vi "Main.vi"() -> ()   [LabVIEW 2011]
uses:
  GUI/Graph/Plot selector.ctl
  Application Structure/User Control/User Indikator.ctl
  Application Structure/User Control/Super User bool indikator.ctl
  GUI/Shart Time Selector.ctl
  GUI/Analog Var Disp 0 sif.ctl
  GUI/Status indicator Black Small.ctl
  GUI/Controls/Graphical rep/Tool Angle.ctl
  Measurments Handling/Cat Alm temp.ctl
  GUI/Status indicator white.ctl
  Measurments Handling/Cat Alm Press.ctl
  Measurments Handling/Cat Alm Gen.ctl
  Measurments Handling/Cat Alm Pow.ctl
  Measurments Handling/Digital GUI/Digital Display cluster.ctl
  Measurments Handling/Digital GUI/Digital Disp small indicator.ctl
  Measurments Handling/Digital GUI/Digital Tricolour Display cluster.ctl
  Measurments Handling/Digital GUI/Digital Tricolour Disp small indicator.ctl
  GUI/Controls/Tristate/Tristate left.ctl
  GUI/Controls/Tristate/Tristate right.ctl
  GUI/Controls/Slips boolean.ctl
  GUI/Controls/Pressure failing boolean long.ctl
  Tool/Tab with tool type tabs.ctl
  GUI/Analog Var Disp Large.ctl
  GUI/Controls/Signal Bar Graph.ctl
  Application Structure/Loop ID.ctl
  emi Lib/System 01/1 - GUI/Background/emi_System Colors.ctl
  emi Lib/System 01/1 - GUI/Background/Private/_emi_ Color defenition.ctl
  emi Lib/Basic/0 - General/Graphix/Private/emi_List Of Graphix.ctl
  Application Structure/System ID.ctl
  emi Lib/System 01/0 - General/S&E reporting/Private/_emi_ S&E Message type.ctl
  emi cndiates/E&S/Monitor/Actino S&E monitor.ctl
  Application Structure/QSM State List.ctl
  Sequence automation/Sequence steps config..ctl
  Sequence automation/Single criteria cluster.ctl
  Sequence automation/Criteria types.ctl
  Sequence automation/Boolean operation.ctl
  Application Structure/Options/Action GFV Settings.ctl
  <vilib>/Platform/TimedLoop/XDataNode/timing_clust.ctl
  <vilib>/Platform/TimedLoop/XDataNode/nitl_modes.ctl
  <vilib>/Platform/TimedLoop/XDataNode/wakeup.ctl
  PCP interface/High Level/PCP High Level Commands.ctl
  PCP interface/PSU Type.ctl
  GUI/Controll refrence groups.ctl
  GUI/Graph/Annotations Tip Strip FGV_cluster.ctl
  Application Structure/Dialog Loop/Dialog selection cluster.ctl
  Application Structure/Dialog box ID.ctl
  Application Structure/Mem Ctls/Mem Ctl Custer.ctl
  Application Structure/Mem Ctls/Mem Graph Ctl Custer.ctl
  GUI/Graph/Y scale cluster.ctl
  GUI/Graph vindu/Settigner fra Main.ctl
  Annotation/Annotation Message.ctl
  Annotation/Actin Annotatino Holder.ctl
  PCP interface/High Level/PCP High Level Telegram.ctl
  Tool/Stroker/def/Tool specific commands.ctl
  Tool/List of tools.ctl
  Events/User Event List.ctl
  emi cndiates/E&S/reate/S&E Event source.ctl
  Tool/Variable List Tool Analog.ctl
  Measurments Handling/Common/Variable List Common Digital.ctl
  Tool/Variable List Tool Digital.ctl
  Measurments Handling/Status Digitalish.ctl
  GUI/Graph/Annotations Tip Strip FGV_data cluster.ctl
  <vilib>/Utility/miscctls.llb/LVPoint32TypeDef.ctl
  <vilib>/event_ctls.llb/eventvkey.ctl
  Sequence automation/Complete sequence cluster holder.ctl
  Sequence automation/User input.ctl
  Measurments Handling/Common/Variable List Common Analog.ctl
  emi Lib/System 01/0 - General/App/Loop control 2/Private/_emi_SMLoop Control Single.vi
  emi Lib/System 01/0 - General/App/Loop control 2/Private/_emi_SMLoop Get State Single.vi
  emi Lib/System 01/0 - General/emi_Set System ID.vi
  emi Lib/System 01/0 - General/App/Loop control 2/Private/_emi_ SMLoop start condition.vi
  emi Lib/System 01/0 - General/App/Loop control 2/Private/_emi_ SMLoop Error Check.vi
  emi Lib/Basic/0 - General/Error/emi_Is Error.vi
  emi Lib/System 01/0 - General/App/Loop control 2/Private/_emi_SMLoop Register new.vi
  emi Lib/System 01/0 - General/emi_Read System ID.vi
  emi Lib/Basic/0 - General/App/emi_Is Dev enviroment.vi
  emi Lib/System 01/0 - General/S&E reporting/emi_Send S&E Error message.vi
  emi Lib/Basic/0 - General/Error/emi_ Is Error state.vi
  emi Lib/System 01/0 - General/Private/_emi_GFV System ID.vi
  emi Lib/System 01/0 - General/S&E reporting/Private/_emi_S&E Q Generator.vi
  Application Structure/QSM/QSM Q holder.vi
  emi Lib/System 01/1 - GUI/Profiling Mar-In/Splash & About/Private/emi_Splash&About Screen.vi
  <vilib>/Utility/VariantDataType/GetNumericInfo.vi
  emi Lib/System 01/0 - General/App/Loop control/Private/_emi_GFV Loop Enable.vi
  emi Lib/System 01/0 - General/App/Loop control/Private/_emi_GFV Loop Linking.vi
  GUI/GFV GUI PCP shown connected.vi
  emi Lib/Basic/1 - GUI/Control tools/emi_Control Enable & Visibility.vi
  emi Lib/Basic/1 - GUI/Control tools/Private/emi_Control enable and visibility array.vi
  emi Lib/System 01/0 - General/Debug/Private/_emi_GFV Debug Disp.vi
  emi Lib/System 01/0 - General/App/Private/_emi_GFV App Close.vi
  emi Lib/System 01/0 - General/App/Loop control/Private/_emi_GFV Loop Running.vi
  emi Lib/Basic/0 - General/App/emi_Application Folder.vi
  emi Lib/System 01/0 - General/App/Loop control 2/Private/_emi_ SMLoop Restart.vi
  emi Lib/System 01/0 - General/App/Loop control 2/Private/_emi_ SMLoop Restart Counter.vi
  emi Lib/System 01/0 - General/App/Loop control/Private/_emi_GFV stop a loop so it can reset.vi
  emi Lib/Basic/0 - General/Time/Private/emi_Time offset holder.vi
  Measurments Handling/Get Modem Status Digital Vars.vi
  <vilib>/Platform/TimedLoop/XDataNode/XDataNode.xnode
  <vilib>/Platform/TimedLoop/XDataNode/XDNodeRunTimeDep.lvlib
  Measurments Handling/Action Analog Handler.ctl
panel:
  out "Subsea Bar Graph":T1 {"Gain" format="%#.0f"; "Signal Quality" format="%#.0f"}
  out "Topside Bar Graph":T1 {"Gain" format="%#.0f"; "Signal Quality" format="%#.0f"}
  in  "Annotation Tip Strip":string
  out "Chart 1":dbl[][](graph)
  in  "Start Run":bool
  in  "String Check Rec":bool
  out "Recording":bool
  in  "Inspect Upper Chart":bool caption="Inspect Chart"
  out "Beagle Panel":T2 caption="Depth"
  out "Annotation Chart":dbl(graph)
  in  "Calculate resistance":bool caption="Upd"
  in  "Start Motor":bool
  in  "Start Telemetry":bool
  out "Tool":T2 caption="Depth"
  out "PCP Control":T5 caption="Depth"
  out "Type tab 2":T7
  out "Str Error Tens1":u16(ring) caption="Error Strk P2"
  out "Strok Tension Sub 1":T2 caption="Upper Tension Sub"
  out "Stroker  2":dbl(slide) caption="Stroker position" scale=0.0..500.0
  out "Strok Pressure 1":T2 caption="Pressure1"
  out "Strok Pressure 2":T2 caption="Pressure2"
  out "Strok Solenoid":T2 caption="Solenoid"
  out "Str Error P1":u16(ring) caption="Error Strk P1"
  out "Str Error P2":u16(ring) caption="Error Strk P2"
  out "Str Error Sol":u16(ring) caption="Error Strk olenoid"
  out "Error Dr Sol":u16(ring)
  out "Error Dr P2":u16(ring)
  out "Error Dr P1":u16(ring)
  out "Dr Solenoid":T2 caption="Solenoid"
  out "Dr Pressure 2":T2 caption="Pressure2"
  out "Dr Pressure 1":T2 caption="Pressure1"
  out "Error Tr Tension Sub 1":u16(ring) caption="Error Dr Sol"
  out "Trac Tension Sub 1":T2 caption="Upper Tension Sub"
  out "Trac Tension Sub 2":T2 caption="Lower Tension Sub"
  out "Error Tr Tension Sub 2":u16(ring) caption="Error Dr Sol"
  out "Type tab 3":T7
  in  "Stroker Tension Sub Zero":bool caption="Solonoid 1 On"
  out "Upper Tension Sub":T8={"Value"=nan, "Unit"="", "Status"=0}
  out "Trac - Lower Tension Sub":T8={"Value"=nan, "Unit"="", "Status"=0} caption="Lower Tension Sub"
  out "Trac - Upper Tension Sub":T8={"Value"=nan, "Unit"="", "Status"=0} caption="Upper Tension Sub"
  in  "Tractor Tension Sub Zero":bool caption="Solonoid 1 On"
  out "Type tab 1":T7
  in  "Force Zero":bool caption="Solonoid 1 On"
  in  "Stroker force limit":dbl=0.5 caption="tonne" min=0.5 step=0.1
  out "Slips total":bool
  out "Stroker":dbl(slide) caption="Stroker position" scale=0.0..500.0
  in  "Stroker Anchor out":bool caption="Solonoid 1 On"
  in  "Stroker Anchor in":bool caption="Solonoid 1 On"
  out "Stroke extenstion":T10={"Value"=nan, "Unit"="", "Status"=0} caption="Resistance" {"Value" format="%#.0f"}
  out "Moving left":T11
  out "Moving right":T12
  out "Stroke force":T10={"Value"=nan, "Unit"="", "Status"=0} caption="Resistance" {"Value" format="%.1f"}
  out "\"Stroke in\" Pressure":T10={"Value"=nan, "Unit"="", "Status"=0} caption="Resistance"
  out "\"Stroke out\" Pressure":T10={"Value"=nan, "Unit"="", "Status"=0} caption="Resistance"
  out "Slips Venstre":T13
  out "Slips Høyre":T13
  out "pressure falling":T14
  in  "Stroker Stroke Stop":bool caption="Solonoid 1 On"
  in  "Stroke setpoint":dbl(slide) caption="mm" min=0.0 step=1.0 scale=0.0..500.0 scale format="%.0g"
  in  "Stroker Stroke Go To":bool caption="Solonoid 1 On"
  in  "Stroker Stroke In":bool caption="Solonoid 1 On"
  in  "Stroker Stroke Out":bool caption="Solonoid 1 On"
  out "Distance from target:":dbl caption="Target seeking" format="%.1f"
  in  "Driller Anchor in":bool caption="Solonoid 1 On"
  in  "Driller Anchor out":bool caption="Solonoid 1 On"
  out "Dr Oil filling mode":T2 caption="Oil filling mode"
  out "Drill bit direaction":T2 caption="Mill Bit direction"
  in  "Driller Stroke out":bool caption="Solonoid 1 On"
  in  "Driller Stroke in":bool caption="Solonoid 1 On"
  in  "Driller Oil filling mode":bool caption="Solonoid 1 On"
  out "Weight on bit":T10={"Value"=nan, "Unit"="", "Status"=0} caption="Resistance" {"Value" format="%#.1f"}
  out "Driller RPM":T10={"Value"=nan, "Unit"="", "Status"=0} caption="RPM" {"Value" format="%#.1f"}
  out "Torque":T10={"Value"=nan, "Unit"="", "Status"=0} caption="Resistance" {"Value" format="%#.1f"}
  in  "Driller RPM":dbl(slide) caption="RPM" min=0.0 max=600.0 scale=0.0..600.0
  in  "Driller Stop":bool
  in  "Driller A Dir":bool
  in  "Driller Dir B":bool
  out "Slips":T13
  out "Sequence user input name":string
  in  "Sequence user input":dbl min=25.0 max=500.0
  out "Next step":string
  out "Current step":string
  out "Time spent on sequence step":string
  out "Sequence progress":string
  in  "Approve step":bool
  in  "Stopp sequence":bool
  in  "Start sequence":bool
  in  "Sequence to run":u16(ring) items=["Default", "demo", "tyts"]
  in  "Relays off":bool caption="Solenoid 1 Off"
  in  "Relays on":bool caption="All Relays"
  out "Tool Rotation":T15 scale=0.0..360.0 scale format="%#.0f"
  out "Relay Status":T5 caption="Depth"
  in  "Upd Default resistance":bool caption="Upd"
  in  "Force Default resistance":bool caption="Force"
  in  "Resistance(Ohm)":dbl=40.0 min=0.0 max=1200.0 format="%#.0f"
  out "HV out":T5 caption="Depth"
  out "PSU":T2 caption="Depth"
  out "PCP":T2 caption="Depth"
  out "Alarms":string[][](table)
  out "Power Level":T16
  out "General level":T17
  out "Press level":T18
  out "Temp level":T19
  out "Tool Angle":T15 caption="Tool Inclination" scale=0.0..180.0
  in  "Create Anotation":bool
  in  "Inspect Lower Chart":bool caption="Inspect Chart"
  out "Controller Temp.":T10={"Value"=nan, "Unit"="", "Status"=0} caption="Tool Temperature"
  in  "Plot G2 R2":T20 {"Line Width" items=["0", "1", "2", "3", "4", "5"]; "Var Tag" items=[""=0, "HVPSU Head Voltage(V)"=1, "HVPSU Current(A)"=3, "Winch Depth(m)"=5, "Winch Line Speed(m/min)"=6, "Winch Wire Tension(kg)"=7, "Tool Max Temperature(degC)"=8, "Tool Acceleration Sum(g)"=15, "Tool Inclination(deg)"=16, "Tool Rotation(deg)"=17, "Head Voltage(V)"=27, "Stroke Extension(mm)"=38, "Stroke Force(tonne)"=41, "Stroker Upper Tension Sub(kg)"=44, "Tractor Upper Tension Sub(kg)"=48, "Tractor Lower Tension Sub(kg)"=49, "-"=100, "HVPSU TS Voltage(V)"=2, "Tool (Controller) Temperature(degC)"=9, "Tool Acceleration X(g)"=12, "Tool Acceleration Y(g)"=13, "Tool Acceleration Z(g)"=14, "PSU Temp(degC)"=26, "Upper Tension Sub Temp(degC)"=30, "Tool Upper Tension Sub Raw(kg)"=31, "Lower Tension Sub Temp(degC)"=32, "Tool Lower Tension Sub Raw(kg)"=33, "Stroke In Force(tonne)"=39, "Stroke Out Force(tonne)"=40, "Stroker Pressure 1(bar)"=42, "Stroker Pressure 2(bar)"=43, "Tool Temperature sensor(degC)"=52, "Tool Motor Current(A)"=54, "TS_Signal_Quality(NA)"=58, "TS_Gain(NA)"=60, "DH_Signal_Quality(NA)"=61, "DH_Gain(NA)"=63, "Link_Status(NA)"=64, "-"=101, "PCP Cable Resistance(Ohm)"=4, "Tool Supply Voltage(V)"=10, "Tool (Controller) Current(A)"=11, "Tool GP Sensor 1(V)"=18, "Tool GP Sensor 2(V)"=19, "Tool (Pressure 1) Temperature(degC)"=20, "Tool Pressure 1 RAW(bar)"=21, "Tool (Pressure 2) Temperature(degC)"=22, "Tool Pressure 2 RAW(bar)"=23, "Tool (Solenoid) Temperature(degC)"=24, "Tool Solenoid Position(m)"=25, "PSU Main Voltage out(V)"=28, "PSU Main Current out(A)"=29, "Tool Motor Voltage(V)"=53, "Tool Motor Torque(tonne)"=55, "Tool weight on bit(tonne)"=56, "Tool Motor RPM(RPM)"=57, "TS_PCB_Temp(degC)"=59, "DH_PCB_Temp(degC)"=62]}
  in  "Plot G2 R1":T20 {"Line Width" items=["0", "1", "2", "3", "4", "5"]; "Var Tag" items=[""=0, "HVPSU Head Voltage(V)"=1, "HVPSU Current(A)"=3, "Winch Depth(m)"=5, "Winch Line Speed(m/min)"=6, "Winch Wire Tension(kg)"=7, "Tool Max Temperature(degC)"=8, "Tool Acceleration Sum(g)"=15, "Tool Inclination(deg)"=16, "Tool Rotation(deg)"=17, "Head Voltage(V)"=27, "Stroke Extension(mm)"=38, "Stroke Force(tonne)"=41, "Stroker Upper Tension Sub(kg)"=44, "Tractor Upper Tension Sub(kg)"=48, "Tractor Lower Tension Sub(kg)"=49, "-"=100, "HVPSU TS Voltage(V)"=2, "Tool (Controller) Temperature(degC)"=9, "Tool Acceleration X(g)"=12, "Tool Acceleration Y(g)"=13, "Tool Acceleration Z(g)"=14, "PSU Temp(degC)"=26, "Upper Tension Sub Temp(degC)"=30, "Tool Upper Tension Sub Raw(kg)"=31, "Lower Tension Sub Temp(degC)"=32, "Tool Lower Tension Sub Raw(kg)"=33, "Stroke In Force(tonne)"=39, "Stroke Out Force(tonne)"=40, "Stroker Pressure 1(bar)"=42, "Stroker Pressure 2(bar)"=43, "Tool Temperature sensor(degC)"=52, "Tool Motor Current(A)"=54, "TS_Signal_Quality(NA)"=58, "TS_Gain(NA)"=60, "DH_Signal_Quality(NA)"=61, "DH_Gain(NA)"=63, "Link_Status(NA)"=64, "-"=101, "PCP Cable Resistance(Ohm)"=4, "Tool Supply Voltage(V)"=10, "Tool (Controller) Current(A)"=11, "Tool GP Sensor 1(V)"=18, "Tool GP Sensor 2(V)"=19, "Tool (Pressure 1) Temperature(degC)"=20, "Tool Pressure 1 RAW(bar)"=21, "Tool (Pressure 2) Temperature(degC)"=22, "Tool Pressure 2 RAW(bar)"=23, "Tool (Solenoid) Temperature(degC)"=24, "Tool Solenoid Position(m)"=25, "PSU Main Voltage out(V)"=28, "PSU Main Current out(A)"=29, "Tool Motor Voltage(V)"=53, "Tool Motor Torque(tonne)"=55, "Tool weight on bit(tonne)"=56, "Tool Motor RPM(RPM)"=57, "TS_PCB_Temp(degC)"=59, "DH_PCB_Temp(degC)"=62]}
  out "Chart 2":dbl[][](graph)
  in  "Plot G2 L2":T20 {"Line Width" items=["0", "1", "2", "3", "4", "5"]; "Var Tag" items=[""=0, "HVPSU Head Voltage(V)"=1, "HVPSU Current(A)"=3, "Winch Depth(m)"=5, "Winch Line Speed(m/min)"=6, "Winch Wire Tension(kg)"=7, "Tool Max Temperature(degC)"=8, "Tool Acceleration Sum(g)"=15, "Tool Inclination(deg)"=16, "Tool Rotation(deg)"=17, "Head Voltage(V)"=27, "Stroke Extension(mm)"=38, "Stroke Force(tonne)"=41, "Stroker Upper Tension Sub(kg)"=44, "Tractor Upper Tension Sub(kg)"=48, "Tractor Lower Tension Sub(kg)"=49, "-"=100, "HVPSU TS Voltage(V)"=2, "Tool (Controller) Temperature(degC)"=9, "Tool Acceleration X(g)"=12, "Tool Acceleration Y(g)"=13, "Tool Acceleration Z(g)"=14, "PSU Temp(degC)"=26, "Upper Tension Sub Temp(degC)"=30, "Tool Upper Tension Sub Raw(kg)"=31, "Lower Tension Sub Temp(degC)"=32, "Tool Lower Tension Sub Raw(kg)"=33, "Stroke In Force(tonne)"=39, "Stroke Out Force(tonne)"=40, "Stroker Pressure 1(bar)"=42, "Stroker Pressure 2(bar)"=43, "Tool Temperature sensor(degC)"=52, "Tool Motor Current(A)"=54, "TS_Signal_Quality(NA)"=58, "TS_Gain(NA)"=60, "DH_Signal_Quality(NA)"=61, "DH_Gain(NA)"=63, "Link_Status(NA)"=64, "-"=101, "PCP Cable Resistance(Ohm)"=4, "Tool Supply Voltage(V)"=10, "Tool (Controller) Current(A)"=11, "Tool GP Sensor 1(V)"=18, "Tool GP Sensor 2(V)"=19, "Tool (Pressure 1) Temperature(degC)"=20, "Tool Pressure 1 RAW(bar)"=21, "Tool (Pressure 2) Temperature(degC)"=22, "Tool Pressure 2 RAW(bar)"=23, "Tool (Solenoid) Temperature(degC)"=24, "Tool Solenoid Position(m)"=25, "PSU Main Voltage out(V)"=28, "PSU Main Current out(A)"=29, "Tool Motor Voltage(V)"=53, "Tool Motor Torque(tonne)"=55, "Tool weight on bit(tonne)"=56, "Tool Motor RPM(RPM)"=57, "TS_PCB_Temp(degC)"=59, "DH_PCB_Temp(degC)"=62]}
  in  "Plot G2 L1":T20 {"Line Width" items=["0", "1", "2", "3", "4", "5"]; "Var Tag" items=[""=0, "HVPSU Head Voltage(V)"=1, "HVPSU Current(A)"=3, "Winch Depth(m)"=5, "Winch Line Speed(m/min)"=6, "Winch Wire Tension(kg)"=7, "Tool Max Temperature(degC)"=8, "Tool Acceleration Sum(g)"=15, "Tool Inclination(deg)"=16, "Tool Rotation(deg)"=17, "Head Voltage(V)"=27, "Stroke Extension(mm)"=38, "Stroke Force(tonne)"=41, "Stroker Upper Tension Sub(kg)"=44, "Tractor Upper Tension Sub(kg)"=48, "Tractor Lower Tension Sub(kg)"=49, "-"=100, "HVPSU TS Voltage(V)"=2, "Tool (Controller) Temperature(degC)"=9, "Tool Acceleration X(g)"=12, "Tool Acceleration Y(g)"=13, "Tool Acceleration Z(g)"=14, "PSU Temp(degC)"=26, "Upper Tension Sub Temp(degC)"=30, "Tool Upper Tension Sub Raw(kg)"=31, "Lower Tension Sub Temp(degC)"=32, "Tool Lower Tension Sub Raw(kg)"=33, "Stroke In Force(tonne)"=39, "Stroke Out Force(tonne)"=40, "Stroker Pressure 1(bar)"=42, "Stroker Pressure 2(bar)"=43, "Tool Temperature sensor(degC)"=52, "Tool Motor Current(A)"=54, "TS_Signal_Quality(NA)"=58, "TS_Gain(NA)"=60, "DH_Signal_Quality(NA)"=61, "DH_Gain(NA)"=63, "Link_Status(NA)"=64, "-"=101, "PCP Cable Resistance(Ohm)"=4, "Tool Supply Voltage(V)"=10, "Tool (Controller) Current(A)"=11, "Tool GP Sensor 1(V)"=18, "Tool GP Sensor 2(V)"=19, "Tool (Pressure 1) Temperature(degC)"=20, "Tool Pressure 1 RAW(bar)"=21, "Tool (Pressure 2) Temperature(degC)"=22, "Tool Pressure 2 RAW(bar)"=23, "Tool (Solenoid) Temperature(degC)"=24, "Tool Solenoid Position(m)"=25, "PSU Main Voltage out(V)"=28, "PSU Main Current out(A)"=29, "Tool Motor Voltage(V)"=53, "Tool Motor Torque(tonne)"=55, "Tool weight on bit(tonne)"=56, "Tool Motor RPM(RPM)"=57, "TS_PCB_Temp(degC)"=59, "DH_PCB_Temp(degC)"=62]}
  in  "HV AV":bool
  in  "HV ON":bool caption="HV PÅ"
  out "Tension":T10={"Value"=nan, "Unit"="", "Status"=0}
  out "Speed":T10={"Value"=nan, "Unit"="", "Status"=0} {"Value" format="%.1f"}
  out "Depth":T10={"Value"=nan, "Unit"="", "Status"=0} {"Value" format="%.1f"}
  out "Resistance":T10={"Value"=nan, "Unit"="", "Status"=0}
  out "Current":T10={"Value"=nan, "Unit"="", "Status"=0} {"Value" format="%.1f"}
  out "Alarm":bool
  out "Voltage Topside":T10={"Value"=nan, "Unit"="", "Status"=0}
  in  "Chart Visible Time selector":T21=enum."1 minute" caption="Time"
  in  "Plot G1 R2":T20 {"Line Width" items=["0", "1", "2", "3", "4", "5"]; "Var Tag" items=[""=0, "HVPSU Head Voltage(V)"=1, "HVPSU Current(A)"=3, "Winch Depth(m)"=5, "Winch Line Speed(m/min)"=6, "Winch Wire Tension(kg)"=7, "Tool Max Temperature(degC)"=8, "Tool Acceleration Sum(g)"=15, "Tool Inclination(deg)"=16, "Tool Rotation(deg)"=17, "Head Voltage(V)"=27, "Stroke Extension(mm)"=38, "Stroke Force(tonne)"=41, "Stroker Upper Tension Sub(kg)"=44, "Tractor Upper Tension Sub(kg)"=48, "Tractor Lower Tension Sub(kg)"=49, "-"=100, "HVPSU TS Voltage(V)"=2, "Tool (Controller) Temperature(degC)"=9, "Tool Acceleration X(g)"=12, "Tool Acceleration Y(g)"=13, "Tool Acceleration Z(g)"=14, "PSU Temp(degC)"=26, "Upper Tension Sub Temp(degC)"=30, "Tool Upper Tension Sub Raw(kg)"=31, "Lower Tension Sub Temp(degC)"=32, "Tool Lower Tension Sub Raw(kg)"=33, "Stroke In Force(tonne)"=39, "Stroke Out Force(tonne)"=40, "Stroker Pressure 1(bar)"=42, "Stroker Pressure 2(bar)"=43, "Tool Temperature sensor(degC)"=52, "Tool Motor Current(A)"=54, "TS_Signal_Quality(NA)"=58, "TS_Gain(NA)"=60, "DH_Signal_Quality(NA)"=61, "DH_Gain(NA)"=63, "Link_Status(NA)"=64, "-"=101, "PCP Cable Resistance(Ohm)"=4, "Tool Supply Voltage(V)"=10, "Tool (Controller) Current(A)"=11, "Tool GP Sensor 1(V)"=18, "Tool GP Sensor 2(V)"=19, "Tool (Pressure 1) Temperature(degC)"=20, "Tool Pressure 1 RAW(bar)"=21, "Tool (Pressure 2) Temperature(degC)"=22, "Tool Pressure 2 RAW(bar)"=23, "Tool (Solenoid) Temperature(degC)"=24, "Tool Solenoid Position(m)"=25, "PSU Main Voltage out(V)"=28, "PSU Main Current out(A)"=29, "Tool Motor Voltage(V)"=53, "Tool Motor Torque(tonne)"=55, "Tool weight on bit(tonne)"=56, "Tool Motor RPM(RPM)"=57, "TS_PCB_Temp(degC)"=59, "DH_PCB_Temp(degC)"=62]}
  in  "Plot G1 R1":T20={"Var Tag"=0, "Color"=16776704, "Line Width"=0} {"Line Width" items=["0", "1", "2", "3", "4", "5"]; "Var Tag" items=[""=0, "HVPSU Head Voltage(V)"=1, "HVPSU Current(A)"=3, "Winch Depth(m)"=5, "Winch Line Speed(m/min)"=6, "Winch Wire Tension(kg)"=7, "Tool Max Temperature(degC)"=8, "Tool Acceleration Sum(g)"=15, "Tool Inclination(deg)"=16, "Tool Rotation(deg)"=17, "Head Voltage(V)"=27, "Stroke Extension(mm)"=38, "Stroke Force(tonne)"=41, "Stroker Upper Tension Sub(kg)"=44, "Tractor Upper Tension Sub(kg)"=48, "Tractor Lower Tension Sub(kg)"=49, "-"=100, "HVPSU TS Voltage(V)"=2, "Tool (Controller) Temperature(degC)"=9, "Tool Acceleration X(g)"=12, "Tool Acceleration Y(g)"=13, "Tool Acceleration Z(g)"=14, "PSU Temp(degC)"=26, "Upper Tension Sub Temp(degC)"=30, "Tool Upper Tension Sub Raw(kg)"=31, "Lower Tension Sub Temp(degC)"=32, "Tool Lower Tension Sub Raw(kg)"=33, "Stroke In Force(tonne)"=39, "Stroke Out Force(tonne)"=40, "Stroker Pressure 1(bar)"=42, "Stroker Pressure 2(bar)"=43, "Tool Temperature sensor(degC)"=52, "Tool Motor Current(A)"=54, "TS_Signal_Quality(NA)"=58, "TS_Gain(NA)"=60, "DH_Signal_Quality(NA)"=61, "DH_Gain(NA)"=63, "Link_Status(NA)"=64, "-"=101, "PCP Cable Resistance(Ohm)"=4, "Tool Supply Voltage(V)"=10, "Tool (Controller) Current(A)"=11, "Tool GP Sensor 1(V)"=18, "Tool GP Sensor 2(V)"=19, "Tool (Pressure 1) Temperature(degC)"=20, "Tool Pressure 1 RAW(bar)"=21, "Tool (Pressure 2) Temperature(degC)"=22, "Tool Pressure 2 RAW(bar)"=23, "Tool (Solenoid) Temperature(degC)"=24, "Tool Solenoid Position(m)"=25, "PSU Main Voltage out(V)"=28, "PSU Main Current out(A)"=29, "Tool Motor Voltage(V)"=53, "Tool Motor Torque(tonne)"=55, "Tool weight on bit(tonne)"=56, "Tool Motor RPM(RPM)"=57, "TS_PCB_Temp(degC)"=59, "DH_PCB_Temp(degC)"=62]}
  in  "Plot G1 L2":T20={"Var Tag"=0, "Color"=11776947, "Line Width"=0} {"Line Width" items=["0", "1", "2", "3", "4", "5"]; "Var Tag" items=[""=0, "HVPSU Head Voltage(V)"=1, "HVPSU Current(A)"=3, "Winch Depth(m)"=5, "Winch Line Speed(m/min)"=6, "Winch Wire Tension(kg)"=7, "Tool Max Temperature(degC)"=8, "Tool Acceleration Sum(g)"=15, "Tool Inclination(deg)"=16, "Tool Rotation(deg)"=17, "Head Voltage(V)"=27, "Stroke Extension(mm)"=38, "Stroke Force(tonne)"=41, "Stroker Upper Tension Sub(kg)"=44, "Tractor Upper Tension Sub(kg)"=48, "Tractor Lower Tension Sub(kg)"=49, "-"=100, "HVPSU TS Voltage(V)"=2, "Tool (Controller) Temperature(degC)"=9, "Tool Acceleration X(g)"=12, "Tool Acceleration Y(g)"=13, "Tool Acceleration Z(g)"=14, "PSU Temp(degC)"=26, "Upper Tension Sub Temp(degC)"=30, "Tool Upper Tension Sub Raw(kg)"=31, "Lower Tension Sub Temp(degC)"=32, "Tool Lower Tension Sub Raw(kg)"=33, "Stroke In Force(tonne)"=39, "Stroke Out Force(tonne)"=40, "Stroker Pressure 1(bar)"=42, "Stroker Pressure 2(bar)"=43, "Tool Temperature sensor(degC)"=52, "Tool Motor Current(A)"=54, "TS_Signal_Quality(NA)"=58, "TS_Gain(NA)"=60, "DH_Signal_Quality(NA)"=61, "DH_Gain(NA)"=63, "Link_Status(NA)"=64, "-"=101, "PCP Cable Resistance(Ohm)"=4, "Tool Supply Voltage(V)"=10, "Tool (Controller) Current(A)"=11, "Tool GP Sensor 1(V)"=18, "Tool GP Sensor 2(V)"=19, "Tool (Pressure 1) Temperature(degC)"=20, "Tool Pressure 1 RAW(bar)"=21, "Tool (Pressure 2) Temperature(degC)"=22, "Tool Pressure 2 RAW(bar)"=23, "Tool (Solenoid) Temperature(degC)"=24, "Tool Solenoid Position(m)"=25, "PSU Main Voltage out(V)"=28, "PSU Main Current out(A)"=29, "Tool Motor Voltage(V)"=53, "Tool Motor Torque(tonne)"=55, "Tool weight on bit(tonne)"=56, "Tool Motor RPM(RPM)"=57, "TS_PCB_Temp(degC)"=59, "DH_PCB_Temp(degC)"=62]}
  in  "Plot G1 L1":T20={"Var Tag"=0, "Color"=16860, "Line Width"=0} {"Line Width" items=["0", "1", "2", "3", "4", "5"]; "Var Tag" items=[""=0, "HVPSU Head Voltage(V)"=1, "HVPSU Current(A)"=3, "Winch Depth(m)"=5, "Winch Line Speed(m/min)"=6, "Winch Wire Tension(kg)"=7, "Tool Max Temperature(degC)"=8, "Tool Acceleration Sum(g)"=15, "Tool Inclination(deg)"=16, "Tool Rotation(deg)"=17, "Head Voltage(V)"=27, "Stroke Extension(mm)"=38, "Stroke Force(tonne)"=41, "Stroker Upper Tension Sub(kg)"=44, "Tractor Upper Tension Sub(kg)"=48, "Tractor Lower Tension Sub(kg)"=49, "-"=100, "HVPSU TS Voltage(V)"=2, "Tool (Controller) Temperature(degC)"=9, "Tool Acceleration X(g)"=12, "Tool Acceleration Y(g)"=13, "Tool Acceleration Z(g)"=14, "PSU Temp(degC)"=26, "Upper Tension Sub Temp(degC)"=30, "Tool Upper Tension Sub Raw(kg)"=31, "Lower Tension Sub Temp(degC)"=32, "Tool Lower Tension Sub Raw(kg)"=33, "Stroke In Force(tonne)"=39, "Stroke Out Force(tonne)"=40, "Stroker Pressure 1(bar)"=42, "Stroker Pressure 2(bar)"=43, "Tool Temperature sensor(degC)"=52, "Tool Motor Current(A)"=54, "TS_Signal_Quality(NA)"=58, "TS_Gain(NA)"=60, "DH_Signal_Quality(NA)"=61, "DH_Gain(NA)"=63, "Link_Status(NA)"=64, "-"=101, "PCP Cable Resistance(Ohm)"=4, "Tool Supply Voltage(V)"=10, "Tool (Controller) Current(A)"=11, "Tool GP Sensor 1(V)"=18, "Tool GP Sensor 2(V)"=19, "Tool (Pressure 1) Temperature(degC)"=20, "Tool Pressure 1 RAW(bar)"=21, "Tool (Pressure 2) Temperature(degC)"=22, "Tool Pressure 2 RAW(bar)"=23, "Tool (Solenoid) Temperature(degC)"=24, "Tool Solenoid Position(m)"=25, "PSU Main Voltage out(V)"=28, "PSU Main Current out(A)"=29, "Tool Motor Voltage(V)"=53, "Tool Motor Torque(tonne)"=55, "Tool weight on bit(tonne)"=56, "Tool Motor RPM(RPM)"=57, "TS_PCB_Temp(degC)"=59, "DH_PCB_Temp(degC)"=62]}
  in  "Voltage Output Override enable":bool caption="HV Manual"
  in  "Tool voltage setpoint(V)":dbl(slide) caption="Tool Voltage" min=0.0 max=450.0 step=1.0 scale=0.0..450.0
  in  "Common Wire Res OR enable":bool caption="OR"
  in  "About":bool
  in  "Options":bool
  out "Voltage Down Hole":T10={"Value"=nan, "Unit"="", "Status"=0} caption="Voltage Downhole(PCP)"
  out "Recording Status":string
  out "User ID":T22
  # "Beagle"
  # "Current Alarms"
  # "Winch"
  # "PSU"
  # "Tool"
  # "Relays"
  # "PCP Control"
  # "Sequence automation"
  # "G"
  # "G"
  # "Tension Subs"
  # "Tension Subs"
  # "Anchor"
  # "Stroke"
  # "Anchor"
  # "Stroke"
  # "Bit control"
  # "Mill Bit"
  # "Mode"
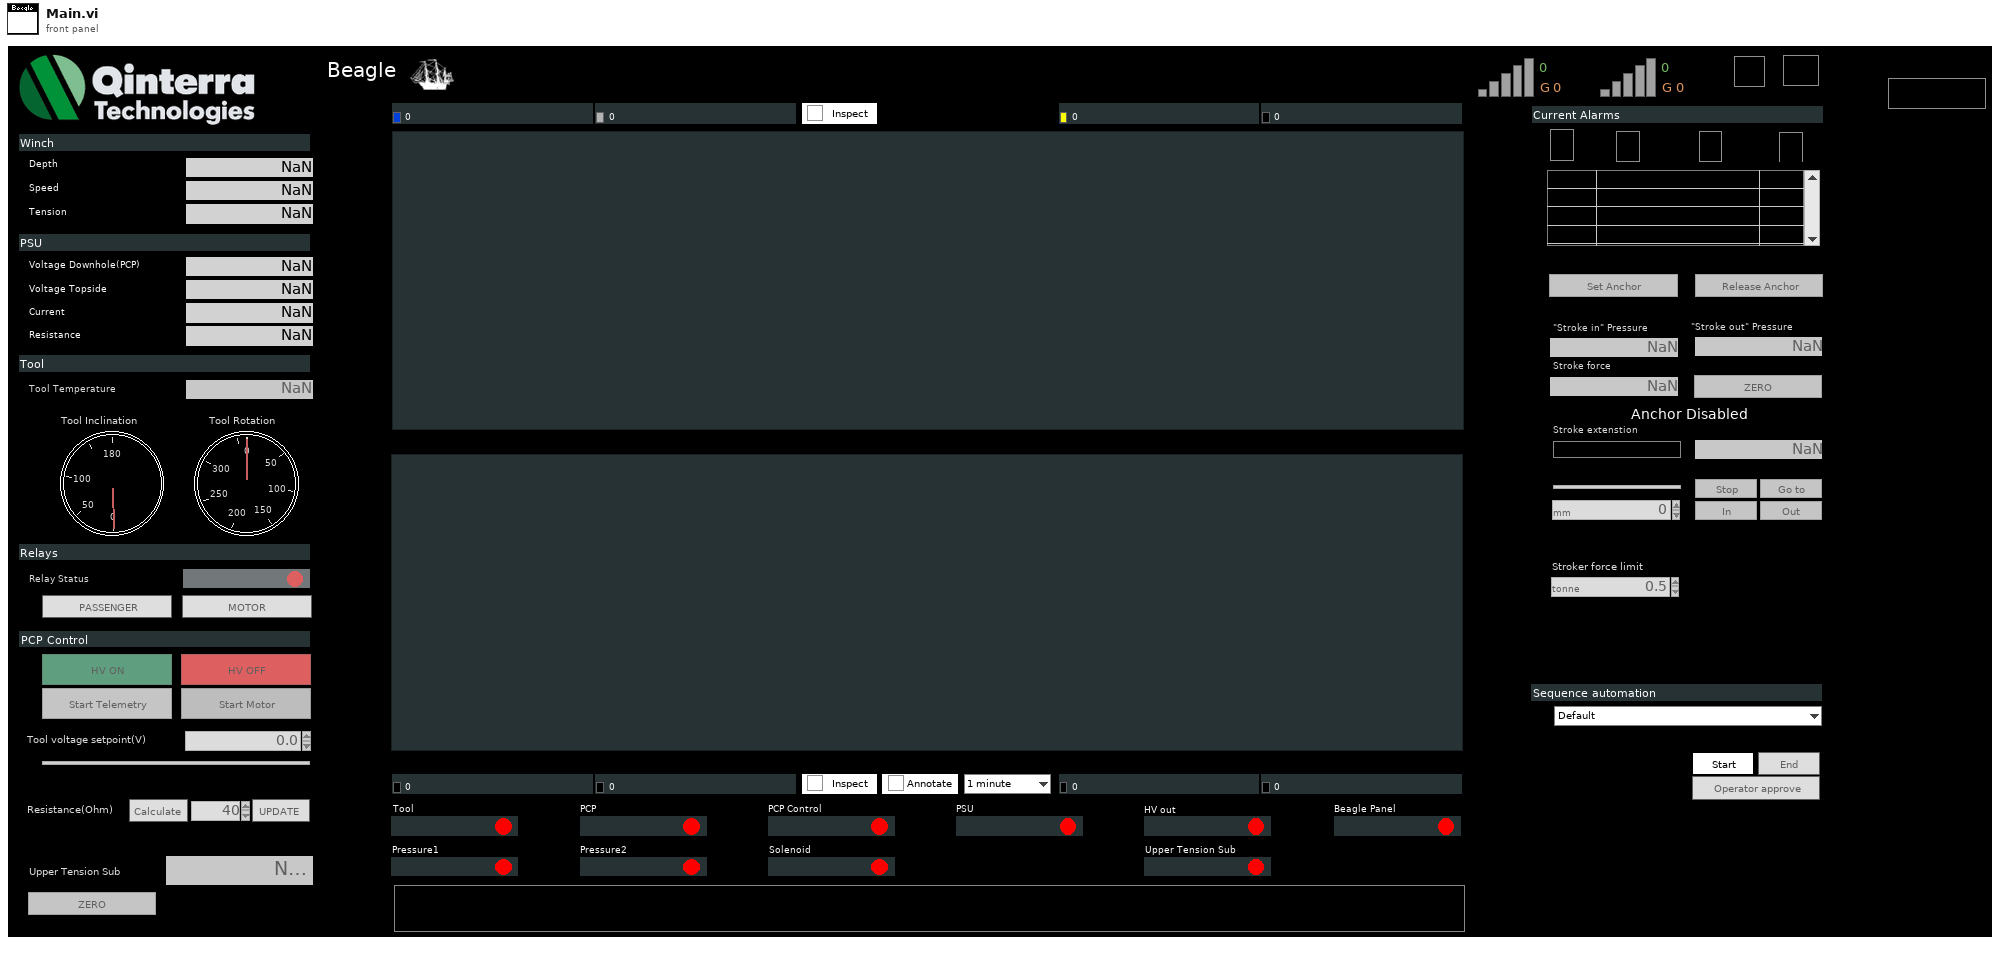
[diagram p1: front panel]
types:
  T1 = typedef "Signal Bar Graph.ctl" = cluster{"Bar Graph":cluster{"Boolean":bool, "Boolean 2":bool, "Boolean 3":bool, "Boolean 4":bool, "Boolean 5":bool}, "Signal Quality":dbl, "Gain":dbl}
  T2 = typedef "Digital Display cluster.ctl" = cluster{"ON/OFF TEXT":string, "Val":T3, "Status":T4}
  T3 = typedef "Digital Disp small indicator.ctl" = u16
  T4 = typedef "Status indicator white.ctl" = u16
  T5 = typedef "Digital Tricolour Display cluster.ctl" = cluster{"ON/OFF TEXT":string, "Val":T6, "Status":T4}
  T6 = typedef "Digital Tricolour Disp small indicator.ctl" = u16
  T7 = typedef "Tab with tool type tabs.ctl" = enum32{"Stroker", "Driller", "Tractor"}
  T8 = typedef "Analog Var Disp Large.ctl" = cluster{"Value":dbl, "Unit":string, "Status":T9}
  T9 = typedef "Status indicator Black Small.ctl" = u16
  T10 = typedef "Analog Var Disp 0 sif.ctl" = cluster{"Value":dbl, "Unit":string, "Status":T9}
  T11 = typedef "Tristate left.ctl" = u16
  T12 = typedef "Tristate right.ctl" = u16
  T13 = typedef "Slips boolean.ctl" = bool
  T14 = typedef "Pressure failing boolean long.ctl" = bool
  T15 = typedef "Tool Angle.ctl" = dbl
  T16 = typedef "Cat Alm Pow.ctl" = cluster{"Power Alarm":bool, "Power Level":T4}
  T17 = typedef "Cat Alm Gen.ctl" = cluster{"General Alarm":bool, "General level":T4}
  T18 = typedef "Cat Alm Press.ctl" = cluster{"Pressure Alarm":bool, "Pressure level":T4}
  T19 = typedef "Cat Alm temp.ctl" = cluster{"Temperature Alarm":bool, "Tempreature level":T4}
  T20 = typedef "Plot selector.ctl" = cluster{"Var Tag":u16, "Color":u32, "Line Width":u16}
  T21 = typedef "Shart Time Selector.ctl" = enum16{"10 Seconds", "1 minute", "5 minutes", "10 minutes", "30 minutes", "1 Hour"}
  T22 = typedef "User Indikator.ctl" = cluster{"User Name":string, "Super User":T23}
  T23 = typedef "Super User bool indikator.ctl" = bool
  T24 = typedef "Loop ID.ctl" = enum16{"Main-QSM", "Main-Dialog", "Main-Ind Upd", "Main-Graph Upd", "Main-Debug", "Main-DebugW1", "Main-DebugW2", "Main-SE Handler", "Interface-PCP", "Interface-CANbus", "Interface-Modem", "Var Handling-Beat", "Var Handling-From PCP", "Var Handling-File storage", "Var Handling-From Simulator", "GUI-GrphW Mast", "GUI-GrphW Slav", "SIM-Tool W1", "SIM-Tool W2", "Alm-Sound", "LEIN-motor", "Tool data gatherer Qer", "Tool Data LEIN STAT2 dekoder", "Indicator Value Update", "Tool STAT2 dedicated reader", "Tool ID handler", "Detail View L1", "Detail View L2", "Main display enable view", "Sequence runner", "Voltage setpoint", "Resistance setpoint", "Stroker Wizard L1", "Stroker Wizard L2", "Alarm Handling", "Annotations Tip Strip", "Magna Interface", "Modem Status", "Var Handling - Modem Status", "Power interface detector"}
  T25 = typedef "Sequence steps config..ctl" = cluster{"Enabled":bool, "Criteria 1":T26, "C1 op C2":T28, "Criteria 2":T26, "Action index":i32, "Action Name":string, "Action value":dbl}
  T26 = typedef "Single criteria cluster.ctl" = cluster{"Criteria":T27, "Time or analog value":dbl, "Primary IO index":i32, "Secondary  IO index":i32, "User_input":bool}
  T27 = typedef "Criteria types.ctl" = enum16{"No criteria(True)", "Time(s)", "Analog IO over", "Analog IO over or equal", "Analog IO under", "Analog IO under or equal", "Analog IO 1 minus Analog IO 2 over", "Digital IO True", "Digital IO False", "Operator approval"}
  T28 = typedef "Boolean operation.ctl" = enum16{"And", "Or", "Xor", "Nand", "Nor", "Nxor", "Implies"}
  T29 = enum16{"GET", "SET", "Get from Ini", "Put in Ini"}
  T30 = typedef "QSM State List.ctl" = enum16{"Idle", "Init <<<Start>>>", "Init Reg Controlers", "Init Stroker Ref FGV", "Init Driller Ref FGV", "Init Tractor Ref FGV", "Init All loops", "Init Mem Ctls", "Init GUI", "Init<<<End>>>", "Show options", "Options updated", "Show User Dialog", "User Updated", "Show About", "Show Help", "Debug Visibility", "End Application", "Mem Ctls", "Mem Graphs", "Post", "-------------", "Dialog Common Analog", "Chart Init", "Chart Var Selector Rings init", "Chart Read Settings from INI", "Chart Clear", "Chart Selection Changed", "Chart Time Changed", "Graph Dialog Show", "Annotation, New", "Annotation Created", "PCP CMD", "Show Welcome screen", "Dialog Tool analog", "Update PCP resistance", "Tool CMD", "Chart single autoscale", "Tool connenction state", "Show detailed view", "Sequences updated", "Show stroker wizard", "Change tool", "Reset Telemetry", "Update control units", "Stop Logging", "Start New Loggfile", "Log Init", "Copy INI files"}
  T31 = typedef "Actino S&E monitor.ctl" = enum16{"GET(type history)", "SET S&E", "(Re)Init", "Get Error state", "Get  Alarm state", "Get All", "Get last  250", "Get Alarm History"}
  T32 = typedef "_emi_ S&E Message type.ctl" = enum16{"Error/Warning", "Note", "Debug", "Event", "Alarm Analog", "Alarm Digital", "Annotation"}
  T33 = typedef "emi_System Colors.ctl" = cluster{"Main Top Panels":T34, "Main Botom Panels":T34, "Graphs":T34, "Dialogs":T34}
  T34 = typedef "_emi_ Color defenition.ctl" = cluster{"Type":T35, "Dark/Primary Color":u32, "Light/Secondary Color":u32, "Extra Color":u32}
  T35 = typedef "emi_List Of Graphix.ctl" = enum16{"FlatColor", "SharpGrad", "ShallowGrad", "GlasGradBord", "GlasGrad", "GlasGradBord 2"}
  T36 = typedef "System ID.ctl" = enum16{"Host"}
  T37 = typedef "XDNodeRunTimeDep.lvlib/timing_clust.ctl" = cluster{"Expected End [f-1]":u64, "Actual End [f-1]":u64, "Finished Late? [f-1]":bool, "Expected End [i-1]":u64, "Actual End [i-1]":u64, "Finished Late? [i-1]":bool, "Expected Start [i]":u64, "Actual Start [i]":u64, "Expected Start [f]":u64, "Actual Start [f]":u64, "Source Name":string, "Structure Name":string, "Period":i64, "Deadline":i64, "Offset":i64, "Start":i64, "Priority":i32, "Timeout":i32, "Mode":T38, "Wakeup Reason":T39, "Error":errorcluster, "Source Type":string, "Secondary Source Type":string, "Global End Time":u64, "Global Start Time":u64, "Frame Duration":u64, "Iteration Duration":u64, "Assigned CPU":i32, "I/O Scan Engine Mode":u32}
  T38 = typedef "XDNodeRunTimeDep.lvlib/nitl_modes.ctl" = enum32{"No Change", "Process missed periods, maintain original phase", "Discard missed periods, maintain original phase", "Process missed periods, ignore original phase", "Discard missed periods, ignore original phase"}
  T39 = typedef "XDNodeRunTimeDep.lvlib/wakeup.ctl" = enum32{"Normal", "Aborted", "Asynchronous wakeup", "Timing source error", "Timed loop error", "Timeout"}
  T40 = typedef "PCP High Level Commands.ctl" = enum16{"HVPSU HV ON", "HVPSU HV OFF", "PCP PC", "PCP Local", "Update Motor Voltage", "Update Cable Resistance", "Final Motor Voltage", "Final Resistance"}
  T41 = typedef "PSU Type.ctl" = enum16{"Unipower", "Magna 8.3A", "Magna 12A", "None"}
  T42 = typedef "Action GFV Settings.ctl" = enum16{"Init", "Get From INI", "Put In INI", "Get Settings", "Get Update Index", "Set Setting"}
  T43 = typedef "Controll refrence groups.ctl" = enum16{"Controller. gen", "Controller . High G", "Stroker", "PCP Online", "PCP Local", "PCP HV On", "Driller", "Stroker Cmd Buttons", "Stroker Anchor Cmd Buttons", "Controller Relay Buttons", "PCP Start Telemetry", "PCP Start Motor", "Tractor", "Modem Status"}
  T44 = typedef "Annotations Tip Strip FGV_cluster.ctl" = cluster{"Annotation Chart Ref":refnum<vi>, "Tip Strip Ref":refnum<vi>}
  T45 = enum8{"Enabled", "Disabled", "Disabled and Grayed Out"}
  T46 = typedef "Dialog selection cluster.ctl" = cluster{"ID":T47, "Details":variant}
  T47 = typedef "Dialog box ID.ctl" = enum16{"About dialog Box", "Options dialog box", "User dialog Box", "Custom dialog...", "Variables Common Analog", "Annotation", "Welcome screen", "Variables Tool Analog", "High G graph display", "Sequence setup", "Unused"}
  T48 = typedef "Mem Ctl Custer.ctl" = cluster{"Tool Voltage  SP":dbl, "Default Resistance(Ohm)":dbl, "Force Default resistance":bool, "Upd Default resistance":bool, "Sequence user input":dbl}
  T49 = typedef "Mem Graph Ctl Custer.ctl" = cluster{"Chart Visible Time selector":T21, "Plot G1 L1":T20, "Plot G1 L2":T20, "Plot G1 R1":T20, "Plot G1 R2":T20, "Plot G2 L1":T20, "Plot G2 L2":T20, "Plot G2 R1":T20, "Plot G2 R2":T20, "G1 Y scale 0":T50, "G1 Y scale 1":T50, "G2 Y scale 0":T50, "G2 Y scale 1":T50}
  T50 = typedef "Y scale cluster.ctl" = cluster{"Maximum":dbl, "Minimum":dbl, "Autoscaling":i32}
  T51 = typedef "Settigner fra Main.ctl" = cluster{"Start Time":timestamp, "Numb Sec Shown":i32, "Plot  L1":T20, "Plot  L2":T20, "Plot  R1":T20, "Plot  R2":T20, "Left Y-scale":T50, "Right Y-scale":T50}
  T52 = typedef "Annotation Message.ctl" = cluster{"Annotation":string, "User":string, "time":timestamp}
  T53 = typedef "Actin Annotatino Holder.ctl" = enum16{"GET Single", "GET All", "GET Time Period", "GET Index", "Get Size", "Add Single", "Replace Single", "Delete Single", "SET All"}
  T54 = typedef "PCP High Level Telegram.ctl" = cluster{"PCP":T40, "SP":dbl}
  T55 = typedef "Tool specific commands.ctl" = enum16{"controller relay 1 on", "controller relay 1 off", "controller relay 2 on", "controller relay 2 off", "Solonoid 1 (master) on", "Solonoid 1 (master) off", "Solonoid 2 (Stroker) on", "Solonoid 2 (Stroker) off", "Solonoid 3 (Anchor) on", "Solonoid 3 (Anchor) off", "Controller relay 1 & 2 on", "Controller relay 1 & 2 off", "Controller relay 1 on, 2 off", "Controller relay 1 off, 2 on", "STROKER tool: Stop Force Mon", "High-G Stop", "High-G Get data", "High-G Stop Get data", "STROKER tool: Stroke out", "STROKER tool: Stroke in", "STROKER tool: Stroke stop", "STROKER tool: Stroke go to", "STROKER tool: Stop Homing", "STROKER tool: Start Force Mon dir in", "STROKER tool: Start Force Mon dir out", "Controller STOP"}
  T56 = typedef "List of tools.ctl" = enum16{"Stroker", "Driller", "Tractor"}
  T57 = typedef "S&E Event source.ctl" = enum16{"User", "Instrument", "Application", "Windows"}
  T58 = typedef "Action Analog Handler.ctl" = enum16{"GET value", "GET Single Frequenzy", "GET All Values", "GET Waveform", "Get Numb Var", "SET Value", "START Buffer", "REG Variable", "BUF size(total antal sekund)", "PULS", "Get a Value at time", "Set initial waveform"}
  T59 = cluster{"Graphs Updated":bool, "Do motor update":bool, "Motor voltage":dbl, "P 3.PSU type DO NOT USE":T41}
  T60 = typedef "Options  All pages and custom.ctl" = cluster{"P 1 (App)":T61, "P 2":T62, "P 3":T63, "P 4":T65, "P 5":T70, "P 6 (Err)":T71, "P 7 (Expert)":T72, "P 8 (Depth)":T74, "C 1":T75, "C 2":T76}
  T61 = typedef "Options Page 1 (App).ctl" = cluster{"Result files":path, "PCP Interface":string, "Tractor/Stroker Interface":string, "Tractor Interface":string, "Modem Status Interface":string, "Audible Alarm":bool, "Force alarm on Technical":bool, "Force alarm on HH":bool, "Force alarm on LL":bool, "Force alarm on H":bool, "Force alarm on L":bool}
  T62 = typedef "Options Page 2.ctl" = cluster{"Solenoid & Relay latching time":u16, "Tractor relay 1":dbl, "Tractor relay 2":dbl, "Tractor Solenoid limit":dbl}
  T63 = typedef "Options Page 3.ctl" = cluster{"Min resistance":dbl, "Max resistance":dbl, "Head voltage range":T64, "Max voltage jump":dbl, "Maximum resistance change":dbl, "Start Telemetry Voltage":dbl, "Start Telemetry Timeout":dbl, "Start Motor Voltage":dbl, "Stop Motor Voltage":dbl, "Pass Mode Warning Voltage":dbl, "Relay Switch Voltage":dbl, "Relay Status Loss Voltage":dbl, "Samples to average":i32, "PSU type DO NOT USE":T41, "Magna OVP":dbl, "Magna Current Limit":dbl}
  T64 = typedef "PCP type List.ctl" = enum16{"0 - 350V", "0 - 450V", "0 - 600V"}
  T65 = typedef "Options Page 4.ctl" = cluster{"Solenoid & Relay latching time":u16, "Stroker relay 1":dbl, "Stroker Relay 2":dbl, "Stroker Solenoid limit":dbl, "Force det.":T66, "Stroke force lim.":dbl, "Anchor Enabled Pressure":dbl, "Tacometer puls":dbl, "Default anchor behavior":T67, "Default stroker behavior":T68, "Default stroker force limit (tonne)":dbl, "Slips Size":T69}
  T66 = typedef "Stroke force selector.ctl" = enum16{"Stroke in = node 1", "Strok out = node 1"}
  T67 = typedef "Default anchor behavior.ctl" = enum16{"Do nothing", "Set Anchor", "Release Anchor"}
  T68 = typedef "Default stroker behavior.ctl" = enum16{"Do nothing", "Stop", "Go Out", "Go In"}
  T69 = typedef "Slips Type Radio.ctl" = enum32{"No Selection", "338 MRS", "3,9 MRS"}
  T70 = typedef "Options Page 5.ctl" = cluster{"Solenoid & Relay latching time":u16, "Driller relay 1":dbl, "Driller Relay 2":dbl, "Driller  Solenoid limit":dbl}
  T71 = typedef "Options Page 6 (Err).ctl" = cluster{"Error and event files":path}
  T72 = typedef "Options Page 7 (Expert).ctl" = cluster{"Show Debug":bool, "Log debug messages":bool, "Additional debug messages":bool, "Start Beagle with Simulator data":bool, "Workshop mode":bool, "Modem baud":u16, "enumCANCOM":bool, "Modem sim":T73, "Telemetry Timeout Disable":i32, "Buffer size":i32, "Upd regular data":bool, "Cable comp":cluster{"VMOD1 Voltage(V)":dbl, "VMOD2 Voltage(V)":dbl}}
  T73 = typedef "Modem simulation setup.ctl" = cluster{"Modem dealay sim":bool, "Sim baud Tx":u16, "Bit Error fraction Tx":dbl, "Sim baud Rx":u16, "Bit Error fraction Rx":dbl}
  T74 = typedef "Options Page 8 (Depth).ctl" = cluster{"Winch Spool Circumference":dbl, "Winch Pulses per Revolution":dbl, "Current Depth":dbl}
  T75 = typedef "Options Custom 1.ctl" = cluster{"Depth Updated":bool, "Depth Offset":dbl}
  T76 = typedef "Options Custom 2.ctl" = cluster{"Placeholder":bool}
  T77 = typedef "RDd return.ctl" = cluster{"AI":T78, "Depth counter(Raw)":i32, "General Ratemeter":dbl, "Digital ports":T79}
  T78 = typedef "RA return Analog I.ctl" = cluster{"HVPSU voltage output (AI 1)":dbl, "HVPSU current output (AI 2)":dbl, "PCP Motor voltage, head voltage (AI 3)":dbl, "PCP Cable resistance (AI 4)":dbl, "Cable tension (AI 5)":dbl, "CCL (AI 6)":dbl}
  T79 = typedef "RP return digital IO.ctl" = cluster{"DO -  HVPSU HV Off":bool, "DO -  HVPSU HV On":bool, "DI -  Unused 1":bool, "DO -  Local(T) / PC(F) mode":bool, "DI - Unused 2":bool, "DI - HVPSU HV On(T)":bool, "DI - PCP Local control(T)":bool, "DI - HVPSU On(T)":bool}
  T80 = typedef "Graph default cluseter.ctl" = cluster{"UL1":T20, "UL2":T20, "UR1":T20, "UR2":T20, "LL1":T20, "LL2":T20, "LR1":T20, "LR2":T20}
  T81 = typedef "Complete sequence cluster holder.ctl" = cluster{"Sequence Name":string, "User input 1":T82, "Steps":T25[]}
  T82 = typedef "User input.ctl" = cluster{"Input name":string, "Minimum value ":dbl, "Maximum value":dbl, "Default value":dbl, "User inp enabled":bool}
  T83 = typedef "User Event List.ctl" = enum16{"ESCAPE", "HV ON", "HV OFF", "HV SP Start adjusting", "HV SP Adjusted", "Sequence Started", "Stop Tool Operation", "Start Telemetry Operation", "Start Motor Operation", "Stroker Activated", "Driller Activated", "Tractor Activated", "Reset Telemetry", "Stop Telemetry", "Stop Motor Operation", "Cable Resistance Updated", "Cable Resistance Update Failed", "String Check Recording Started", "String Check Recording Stopped", "STROKER tool: Stroke enable Solenoid ON", "STROKER tool: Stroke enable Solenoid OFF", "STROKER tool: Stroke direction Solenoid ON", "STROKER tool: Stroke direction Solenoid OFF", "STROKER tool: Anchor Solenoid ON", "STROKER tool: Anchor Solenoid OFF", "Stroker - Set force and pressure to ZERO", "Stroker - Set tension subs to ZERO", "Mono Relay ON - PASS mode", "Hepta Relay ON - PASS mode", "Mono Relay OFF - MOTOR mode", "Hepta Relay OFF - MOTOR mode", "Relays set to passenger mode", "Relays set to motor mode", "Tractor - Set Tension Subs to ZERO", "High-G monitoring Stop", "High-G data retreival requested", "High-G data stop retreival requested", "High-G data retreived", "STROKER tool: Stroker position override sent", "Stroker Stop", "Stroker Extend", "Stroker Retract", "Stroker go to Position", "Controller Stop command", "Node clear error", "STROKER tool: Stroke stop homing", "STROKER tool: Start Monitoring", "STROKER tool: Stop Monitoring", "Sequence start", "Sequence stop", "Sequence stopped", "Sequence step approved", "Sequence action", "Failed sequence step, Retry", "Failed sequence step, Continue", "Failed sequence step, Abort", "Run Started", "Run Stopped"}
  T84 = typedef "Variable List Tool Analog.ctl" = enum16{"Tool Max Temperature", "Tool (Controller) Temperature", "Tool Supply Voltage", "Tool (Controller) Current", "Tool Acceleration X", "Tool Acceleration Y", "Tool Acceleration Z", "Tool Acceleration Sum", "Tool Inclination", "Tool Rotation", "Tool GP Sensor 1", "Tool GP Sensor 2", "Tool (Pressure 1) Temperature", "Tool Pressure 1 RAW", "Tool (Pressure 2) Temperature", "Tool Pressure 2 RAW", "Tool (Solenoid) Temperature", "Tool Solenoid Position", "PSU Temp", "Head Voltage", "PSU Main Voltage out", "PSU Main Current out", "Upper Tension Sub Temp", "Tool Upper Tension Sub Raw", "Lower Tension Sub Temp", "Tool Lower Tension Sub Raw", "Tool Var27 - Reserved", "Tool Var28 - Reserved", "Tool Var29 - Reserved", "Tool Var30 - Reserved", "Stroke Extension", "Stroke In Force", "Stroke Out Force", "Stroke Force", "Stroker Pressure 1", "Stroker Pressure 2", "Stroker Upper Tension Sub", "Stroker Lower Tension Sub", "Stroker Var09 - Reserved", "Stroker Var10 - Reserved", "Tractor Upper Tension Sub", "Tractor Lower Tension Sub", "Tractor Var03 - Reserved", "Tractor Var04 - Reserved", "Tool Temperature sensor", "Tool Motor Voltage", "Tool Motor Current", "Tool Motor Torque", "Tool weight on bit", "Tool Motor RPM"}
  T85 = typedef "Fixed Analog Channel Definition.ctl" = cluster{"ID":u16, "Name":string, "Quantity":T86, "Unit":string, "Maximum upd":T87, "Comment":string, "Help file Name":string, "Help file Section ":string, "Category":T88, "User adjustable Scaling":bool, "Default Scaling":T89, "Default Unit":i32, "Classification":T90}
  T86 = typedef "Quantity enum.ctl" = enum16{"NA", "Acceleration", "Angle", "Current", "Force", "Distance", "Pressure", "Resistance", "Rotational Speed", "Speed", "Temperature", "Tension", "Torque", "Voltage", "Weight"}
  T87 = typedef "Update frequensies.ctl" = enum16{"2 Hz", "1 Hz", "0.1 Hz"}
  T88 = typedef "Channel catagory Enum.ctl" = enum16{"No Category", "Power", "Temperature", "Pressure"}
  T89 = typedef "Scaling.ctl" = cluster{"Gain":dbl, "Offset":dbl}
  T90 = typedef "Channel Classification Enum.ctl" = enum16{"Basic", "Advanced", "Expert", "Unused"}
  T91 = typedef "User Setting Analog Channel Bg.ctl" = cluster{"Scaling":T89, "Limits and responces":T92, "Allow Graph selection by user":bool, "Unit":u16}
  T92 = typedef "Alarm Setup Analog.ctl" = cluster{"Technical Error(NA)":T93, "LL":T93, "L":T93, "H":T93, "HH":T93, "Limits":T95}
  T93 = typedef "Alarm Responce.ctl" = cluster{"Action":T94, "Alarm":bool}
  T94 = typedef "Action List.ctl" = enum16{"No Action", "Stop Motor", "Turn Off HV"}
  T95 = typedef "Limits.ctl" = cluster{"LL":dbl, "L":dbl, "H":dbl, "HH":dbl}
  T96 = typedef "Project infor with project path.ctl" = cluster{"Project path":path, "data":T97, "Comment":string}
  T97 = typedef "Project in icluster.ctl" = cluster{"Job and Site":T98, "Tool":T100, "Run Information":T101}
  T98 = typedef "Job and site cluster.ctl" = cluster{"Project Number":string, "Client Company":string, "Country":T99, "Field":string, "Rig":string, "Well":string}
  T99 = typedef "List of all contrys(combo box).ctl" = string
  T100 = typedef "Tool registration ID.ctl" = cluster{"Tractor type":string, "Tool":string, "Serial #":string}
  T101 = typedef "Run Information.ctl" = cluster{"Active Run":bool, "String Check Rec":bool, "Run Number":i32, "Time of File Start":string}
  T102 = typedef "_emi_ SMLoop sates.ctl" = enum16{"Init", "Standby", "Start", "Normal Operation", "Stop", "Error Handling", "End", "Post"}
  T103 = cluster{"Op button disabled":bool, "Perform action":bool, "Step index":i32, "Action time":timestamp, "Sequences":T81}
  T104 = typedef "Variable List Common Digital.ctl" = enum16{"PCP Connected", "PCP PC Control", "HV PSU connected", "HV PSU HV Active", "Modem Connected", "Tool Connected", "CanBus interface"}
  T105 = typedef "Variable List Tool Digital.ctl" = enum16{"Tool Error Controller", "Tool Stopped Controller", "Tool Relay 1", "Tool Relay 2", "Tool Both Relays", "Tool node Pressure 1", "Tool Error Pressure 1", "Tool Stopped Pressure 1", "Tool node Pressure 2", "Tool Error Pressure 2", "Tool Stopped Pressure 2", "Tool node Solenoid", "Tool Error Solenoid", "Tool Stopped Solenoid", "Tool Solenoid 1", "Tool Solenoid 2", "Tool Solenoid 3", "Tool node PSU", "Tool Error PSU", "Tool Stopped PSU", "Upper Tension Sub", "Tool Error Upper Tension Sub", "Tool Stopped Upper Tension Sub", "Lower Tension Sub", "Tool Error Lower Tension Sub", "Tool Stopped Lower Tension Sub", "Stroke Target seeking", "Stroke Moving Out", "Stroke Moving Inn", "Stroke valves set for Out", "Stroke valves set for In", "Stroke In (force)", "Stroke Out (force)", "Stroke Force decreasing(in)", "Stroke Force decreasing(out)", "Stroke Force change not correct", "Stroke SLIPS established P1", "Stroke SLIPS established P2", "Stroke SLIPS established", "Stroke Pressure Monitor Ongoing", "Stroke Pressure Monitor Ending ", "Tool Stroke enable Valve", "Tool Stroke direction Valve", "Tool Anchor Valve", "Stroker Var19 - Reserved", "Stroker Var20 - Reserved", "Stroker Var21 - Reserved", "Stroker Var22 - Reserved", "Stroker Var23 - Reserved", "Stroker Var24 - Reserved", "Tractor Var1 - Reserved", "Tractor Var2 - Reserved", "Tractor Var3 - Reserved", "Tractor Var4 - Reserved", "Tractor Var5 - Reserved", "Tractor Var6 - Reserved", "Tractor Var7 - Reserved", "Tractor Var8 - Reserved", "Oil filling mode", "Mill Bit Direction", "Position control", "Anchor", "Driller Var5 - Reserved", "Driller Var6 - Reserved", "Driller Var7 - Reserved", "Driller Var8 - Reserved"}
  T106 = typedef "Catagorised alarm state.ctl" = cluster{"Alarm":bool, "Status":T107}
  T107 = typedef "Status Indikator Helper.ctl" = enum16{"Norm", "L", "H", "LL", "HH", "Value", "Technical"}
  T108 = typedef "Status Digitalish.ctl" = enum16{"NA", "False", "True"}
  T109 = typedef "Variable List Common Analog.ctl" = enum16{"HVPSU Head Voltage", "HVPSU TS Voltage", "HVPSU Current", "PCP Cable Resistance", "Winch Depth", "Winch Line Speed", "Winch Wire Tension"}
  T110 = cluster{"Delayed update":bool, "Itt between upd":i32}
  T111 = typedef "Annotations Tip Strip FGV_data cluster.ctl" = cluster{"Enabled":bool, "Point32":T112}
  T112 = typedef "LVPoint32TypeDef.ctl" = cluster{"Horizontal":i32, "Vertical":i32}
  T113 = typedef "eventvkey.ctl" = enum16{"ASCII", "Enter", "Return", "Shift", "Ctrl", "Alt", "Cmd", "Opt", "Caps", "NumLock", "Clear", "Break", "Up", "Down", "Left", "Right", "Insert", "Delete", "Home", "End", "PageUp", "PageDown", "Escape", "Help", "Pause", "ScrollLock", "F1", "F2", "F3", "F4", "F5", "F6", "F7", "F8", "F9", "F10", "F11", "F12", "F13", "F14", "F15", "F16", "F17", "F18", "F19", "F20", "F21", "F22", "F23", "F24", "Play", "VolumeUp", "VolumeDown", "Mute", "Two Byte Char"}
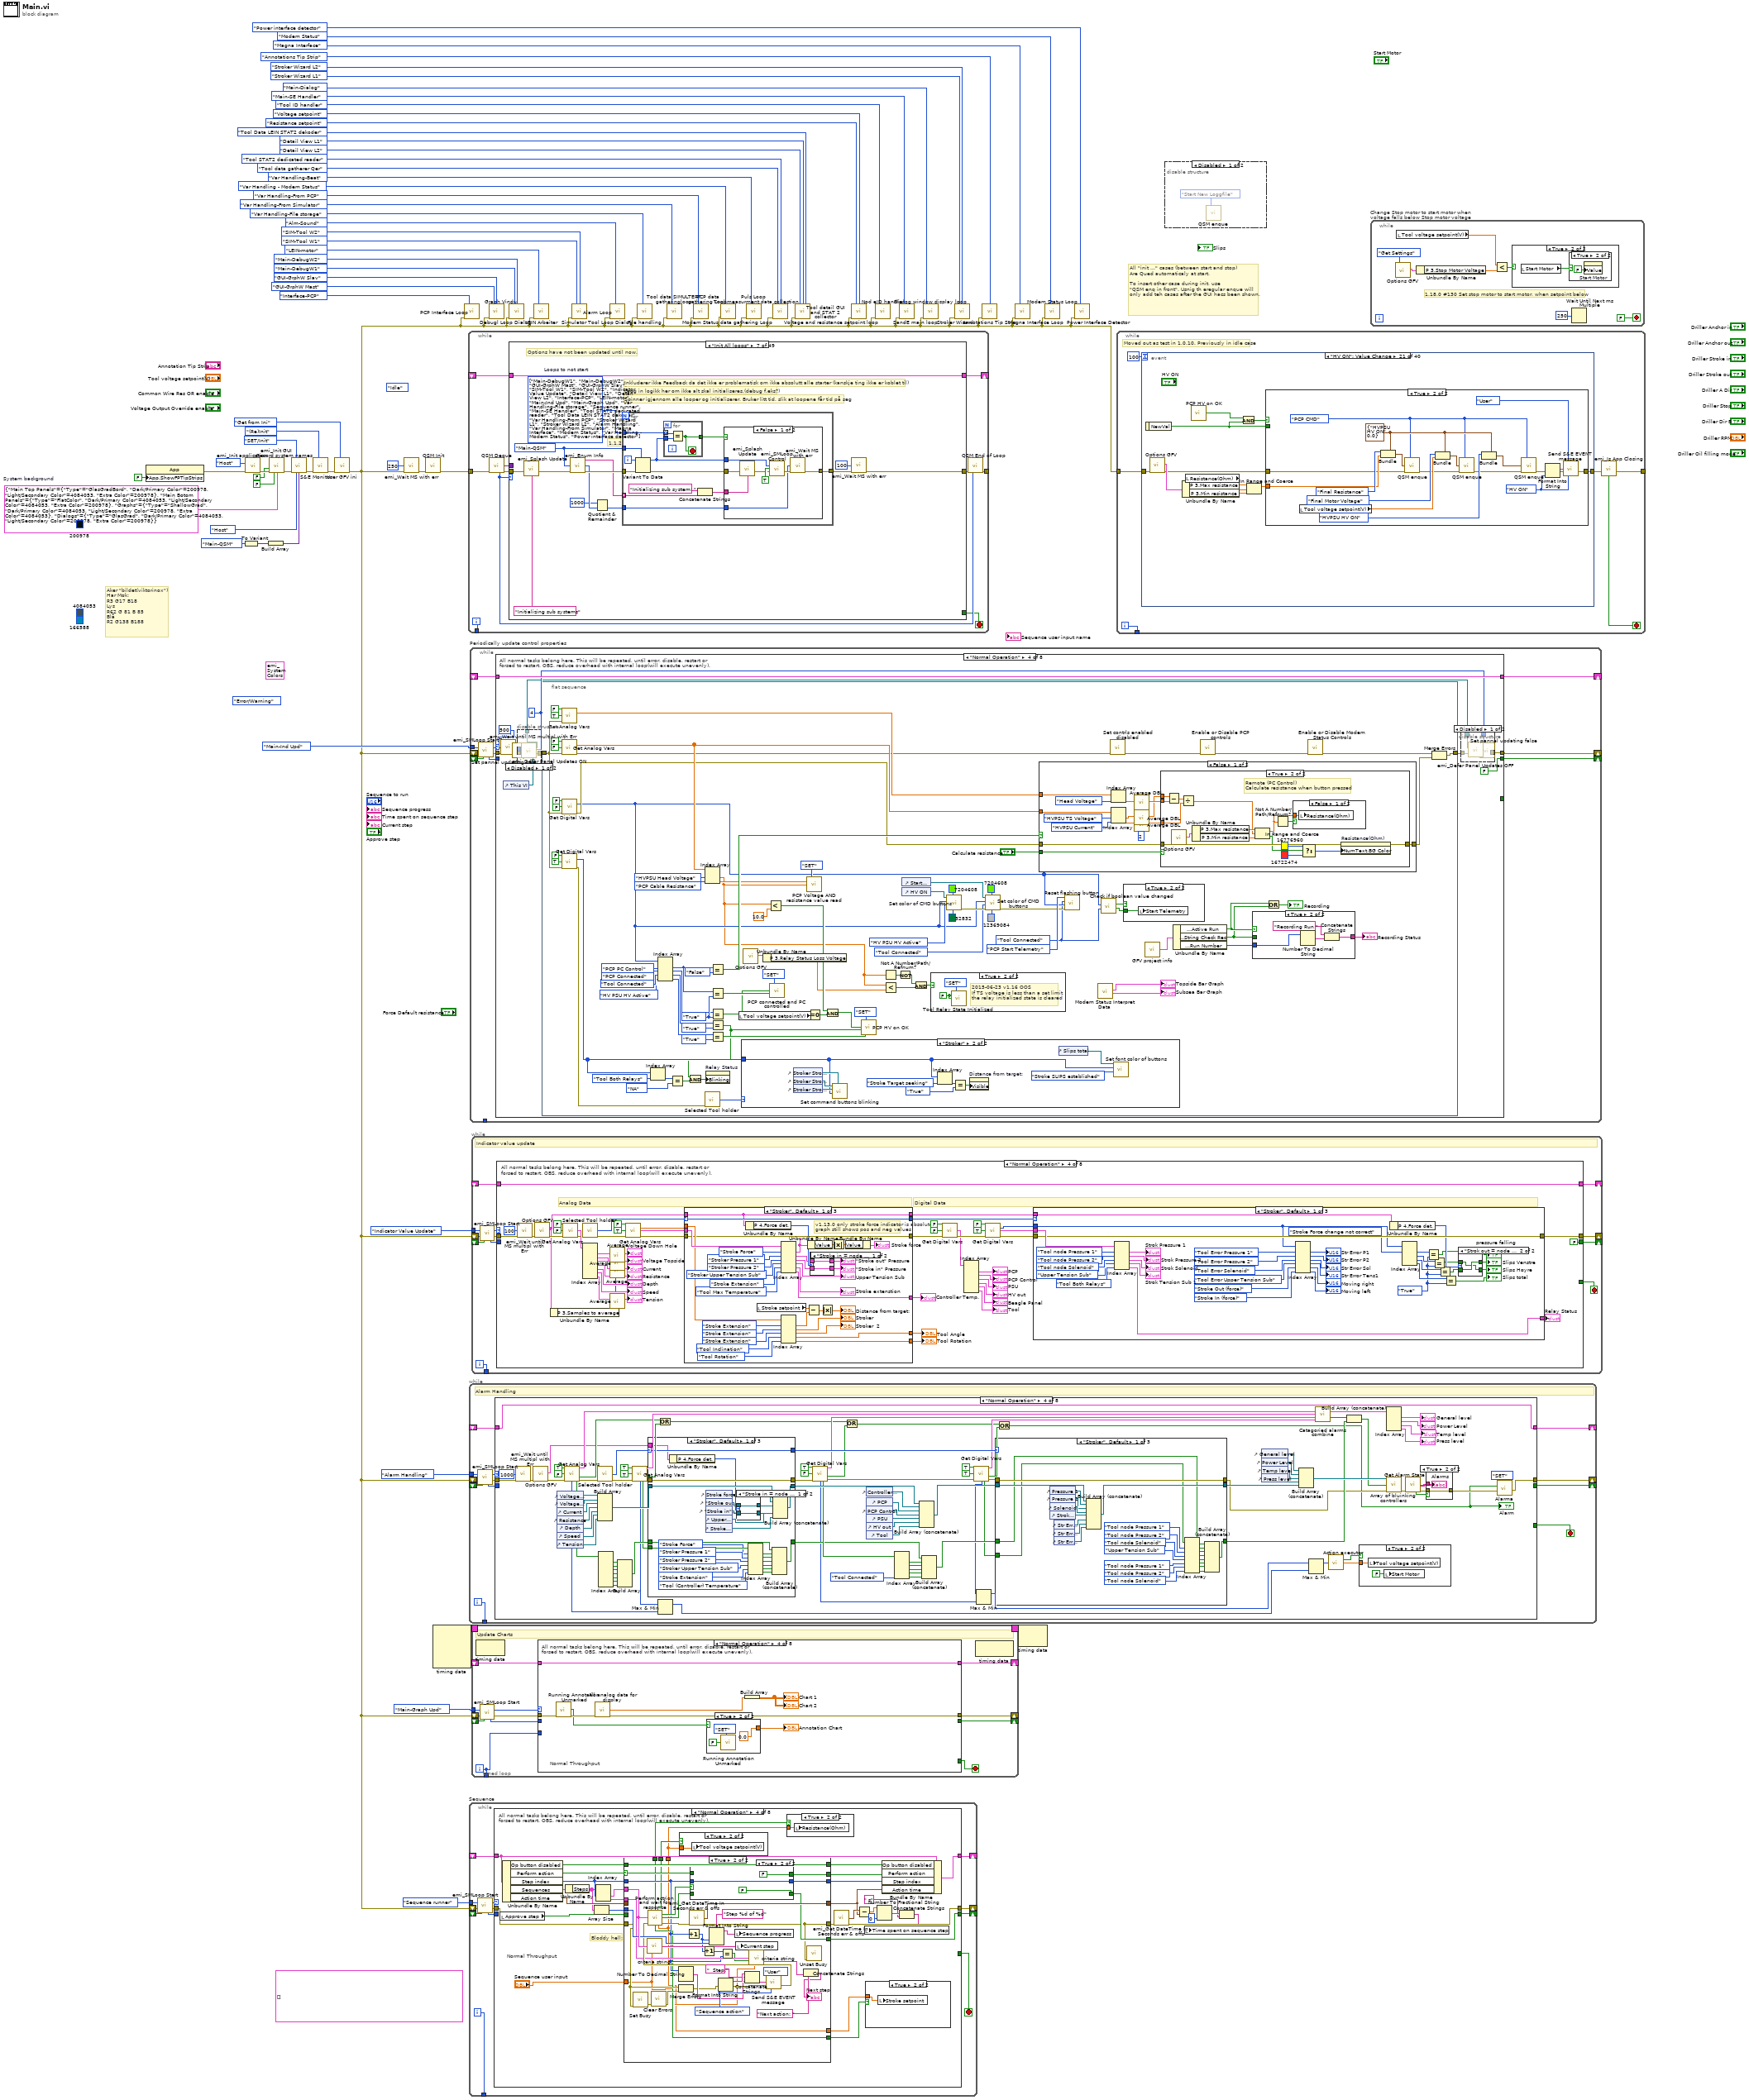
[diagram p0: block diagram]
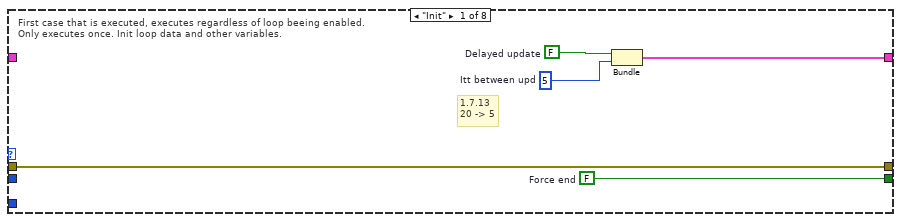
[diagram p5: hidden frame]
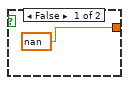
[diagram p8: hidden frame]
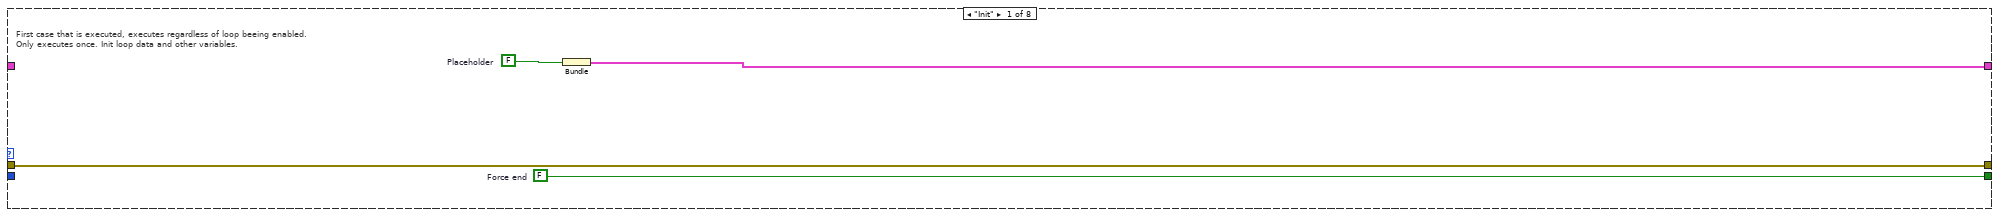
[diagram p13: hidden frame]
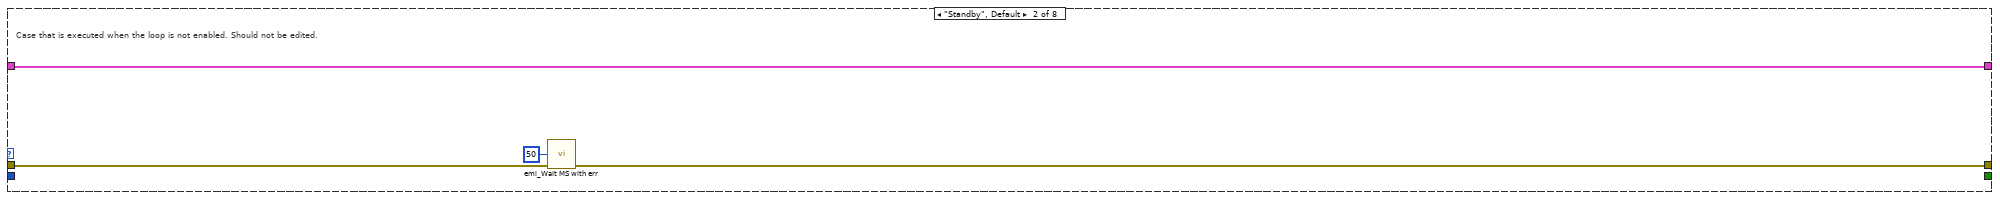
[diagram p14: hidden frame]
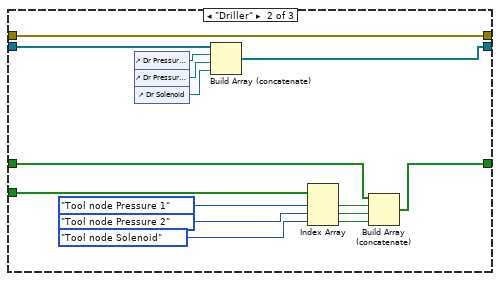
[diagram p18: hidden frame]
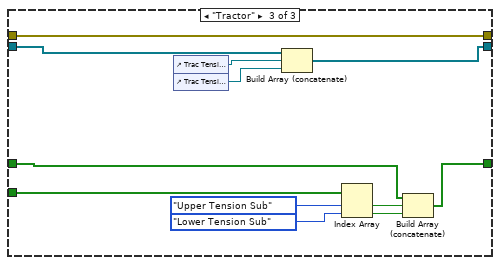
[diagram p19: hidden frame]
diagram:
  (unwired) T25[] [] ("Steps")
  (unwired) QSM_State_List."Idle" ("State")
  (unwired) _emi__S&E_Message_type."Error/Warning" ("Type")
  (unwired) u32 200978 ("Dark/Primary Color")
  (unwired) u32 4084053 ("Light/Secondary Color")
  (unwired) u32 166588 ("Extra Color")
  (unwired) T33 {"Main Top Panels"={"Type"=enum."GlasGradBord 2", "Dark/Primary Color"=0, "Light/Secondary Color"=9868950, "Extra Color"=0}, "Main Botom Panels"={"Type"=enum."FlatColor", "Dark/Primary Color"=11776947, "Light/Secondary Color"=11776947, "Extra Color"=0}, "Graphs"={"Type"=enum."ShallowGrad", "Dark/Primary Color"=11776947, "Light/Secondary Color"=0, "Extra Color"=11776947}, "Dialogs"={"Type"=enum."GlasGrad", "Dark/Primary Color"=16448250, "Light/Secondary Color"=11776947, "Extra Color"=0}} ("System background")
  w57 = T33 {"Main Top Panels"={"Type"=enum."GlasGradBord", "Dark/Primary Color"=200978, "Light/Secondary Color"=4084053, "Extra Color"=200978}, "Main Botom Panels"={"Type"=enum."FlatColor", "Dark/Primary Color"=4084053, "Light/Secondary Color"=4084053, "Extra Color"=200978}, "Graphs"={"Type"=enum."ShallowGrad", "Dark/Primary Color"=4084053, "Light/Secondary Color"=200978, "Extra Color"=4084053}, "Dialogs"={"Type"=enum."GlasGrad", "Dark/Primary Color"=4084053, "Light/Secondary Color"=200978, "Extra Color"=200978}}  # System background
  # "Aker \"bildet(viktorinox\")\nHar Møk:\nR3 G17 B18\nLys\nR62 G 81 B 85\nBlå\nR2 G138 B188"
  # "All \"init ...\" cases (between start and stop)\nAre Qued automaticaly at start.\n\nTo insert other case during init, use\n\"QSM enq in front\". Usnig th eregular enque will \nonly add teh cases after the GUI hacs been shown."
  n1 = property class="App"("App.ShowFPTipStrips"=FALSE ("Application:Show FP Tip Strips")) -> (error out=w9:errorcluster)  [unwired: 2 in, 1 out]
  n2 = To Variant(anything=Loop_ID."Main-QSM" ("Loop ID")) -> (Variant=w48:variant)
  n3 = call "emi_Init application.vi"("System ID(0)"=System_ID."Host" ("Loop ID"), "error in (no error)"=w9) -> ("error out"=w58:errorcluster)  [unwired: 13 in]
  n4 = Build Array(w48) -> (w47:variant[])
  n5 = call "emi_Init GUI.vi"("Change GUI background(T)"=FALSE ("Change graph backgrounds(T)"), "error in"=w58, "Change graph backgrounds(T)"=FALSE, "System background"=w57) -> ("error out"=w52:errorcluster)  [unwired: 11 in]
  n6 = call "Record system names.vi"("Action(GET)"=enum16{"GET", "SET/Init"}."SET/Init", "error in (no error)"=w52, "System type"=System_ID."Host" ("Loop ID"), "System Loops"=w47) -> ("error out"=w36:errorcluster)  [unwired: 7 in, 4 out]
  n7 = call "S&E Monitor.vi"("Action(GET 250)"=Actino_S&E_monitor."(Re)Init", "error in (no error)"=w36) -> ("error out"=w21:errorcluster)  [unwired: 12 in, 1 out]
  n8 = call "User GFV ini.vi"("Action(GET)"=T29."Get from Ini", "error in (no error)"=w21) -> ("error out"=w2:errorcluster)  [unwired: 12 in, 1 out]
  n9 = call "emi_Wait MS with err.vi"("milliseconds to wait(0)"=u32 250, "error in (no error)"=w2) -> ("error out"=w23:errorcluster)  [unwired: 13 in]
  n10 = call "QSM Init.vi"("error in"=w23) -> ("error out"=w24:errorcluster)  [unwired: 14 in]
  n11 = node-c288() -> (w12:T37)  [unwired: 4 in]
  n12 = call "PCP Interface Loop.vi"("PCP IO Loop ID"=Loop_ID."Interface-PCP" ("Loop ID"), "error in (no error)"=w2) -> ()  [unwired: 14 in]
  n13 = while {
    shift-right: [w66] -> _
    shift-left: _ -> [w65]
    tunnel: [w60] -> _
    tunnel: [w63] -> _
    tunnel: w24 -> [w59]
    i -> [w60]
    stop <- w61 stop-if-true
    n14 = call "QSM Deque.vi"("error in"=w59) -> ("Anything"=w67:variant, "State"=w62:T30, "error out"=w68:errorcluster)  [unwired: 12 in]
    n15 = case shown="\"Init All loops\"" w62 {
      tunnel: w68 -> [w71 w112 w162 w190 w209 w217 w230 w257 w300 w317 w370 w404 w414 w440 w453 w458 w469 w480 w500 w518 w559 w565 w571 w578 w609 w631 w704 w745 w802 w842 w870 w894 w910 w937 w946 w948 w961 w990 w999 w1004 w1011 w1021 w1031 w1052 w1062 w1071 w1083 w1114 w1213]
      tunnel: w67 -> [_ _ _ _ _ _ _ _ _ _ _ _ _ _ _ w460 _ _ _ _ _ _ _ _ _ _ _ _ _ w831 _ w893 w911 _ _ _ w960 w989 w998 _ _ _ w1026 _ _ _ _ _ _]
      tunnel: [w75 w115 w163 w191 w210 w218 w232 w267 w302 w322 w374 w405 w418 w441 w454 w462 w470 w472 w512 w516 w564 w566 w572 w580 w610 w657 w705 w722 w803 w848 w882 w896 w902 w941 w947 w949 w962 w992 w1000 w1005 w1012 w1022 w1035 w1060 w1065 w1073 w1085 w1112 w1223] -> w66
      tunnel: w65 -> [w76 _ w163 w191 w210 w218 w232 w267 w302 w322 w374 w405 w418 w441 w454 w462 w470 w472 w512 w516 w564 w566 w572 w580 w610 w657 w705 w723 w803 w848 w882 w896 w898 w941 w947 w949 w962 w992 w1000 w1005 w1012 w1022 w1035 w1060 w1065 w1073 w1085 w1112 w1223]
      tunnel: [w77 w102 w162 w190 w209 w217 w219 w259 w276 w304 w369 w397 w413 w419 w449 w461 w467 w493 w508 w521 w556 w565 w567 w577 w608 w638 w687 w725 w801 w847 w878 w885 w904 w936 w942 w948 w952 w976 w994 w1003 w1007 w1020 w1024 w1049 w1061 w1067 w1084 w1113 w1212] -> w64
      tunnel: [FALSE _ _ _ _ _ _ _ _ _ _ _ _ _ _ _ _ _ _ _ _ _ _ _ _ _ _ _ _ _ _ _ _ _ _ _ _ _ _ _ _ _ _ _ _ _ _ _ _] -> w61
      frame "Idle", Default {
        n16 = flat-sequence {
          tunnel: w71 -> [w79]
          tunnel: [w79] -> w70
          frame #0 {
            # "Pre 1.0.10 this \nheld the event \ncase"
            n17 = Wait Until Next ms Multiple(millisecond multiple=u32 25) -> ()  [unwired: 1 out]
          }
        }
        n18 = call "PSU interface to use GFV.vi"() -> ("PSU type  out"=w69:T41)  [unwired: 14 in, 1 out]
        n19 = Unbundle By Name(w76) -> ("Do motor update"=w73:bool, "Motor voltage"=w72:dbl)
        n20 = case shown="True" w73 {
          tunnel: w70 -> [w81 w84]
          tunnel: w72 -> [_ w86]
          tunnel: [w81 w83] -> w77
          tunnel: w69 -> [_ w82]
          frame False {
          }
          frame True {
            n21 = call "Send PCP command.vi"("PSU type"=w82, "PCP"=PCP_High_Level_Commands."Final Motor Voltage", "SP"=w86, "error out 2"=w84) -> ("error out"=w87:errorcluster)  [unwired: 8 in, 3 out]
            n22 = call <vilib>:"Clear Errors.vi"("error in (no error)"=w87) -> ("error out"=w83:errorcluster)  [unwired: 6 in]
          }
        }
        n23 = Bundle By Name(cluster=w76, "Do motor update"=FALSE ("Do moter update")) -> (w75:T59)
      }
      frame "Init <<<Start>>>" {
        w99 = FALSE  # Do motor update
        w100 = 0.0  # Motor voltage
        w116 = FALSE  # Graphs Updated
        # "v1.17 2015-09-10\nMoved reading of all INI files here so\nthe old values are not lost when the\n\noperator use the Exit buttons in the \nearly project configuration dialogs"
        # "Changes to the PSU type setting will not be\napplied until the next time Beagle is started\nhence the original status has to be maintained"
        # "Loopene skal ikke være startet her, så holder"
        n24 = call "emi_Splash Update.vi"("error In"=w112, "Task Text"="Initializing main QSM data carrier" ("Status text")) -> ("error out"=w107:errorcluster)  [unwired: 13 in]
        n25 = call "emi_Splash Update.vi"("error In"=w107, "Task Text"="Retrieving stored settings" ("Status text")) -> ("error out"=w97:errorcluster)  [unwired: 13 in]
        n26 = call "Options GFV.vi"("error in (no error)"=w97, "Action(Get Settings)"=Action_GFV_Settings."Init") -> ("error out"=w109:errorcluster)  [unwired: 15 in, 2 out]
        n27 = call "Options GFV.vi"("error in (no error)"=w109, "Action(Get Settings)"=Action_GFV_Settings."Get From INI") -> ("error out"=w92:errorcluster)  [unwired: 15 in, 2 out]
        n28 = call "Normal User Default Chart holder FGV.vi"("Action(GET)"=T29."Get from Ini", "error in (no error)"=w92) -> ("error out"=w91:errorcluster)  [unwired: 12 in, 1 out]
        n29 = call "MEM Graph Holder.vi"("Action(GET)"=T29."Get from Ini", "error in (no error)"=w91) -> ("error out"=w90:errorcluster)  [unwired: 12 in, 1 out]
        n30 = call "MEM Ctl Holder.vi"("Action(GET)"=T29."Get from Ini", "error in (no error)"=w90) -> ("error out"=w89:errorcluster)  [unwired: 12 in, 1 out]
        n31 = call "emi_Splash Update.vi"("error In"=w89, "Task Text"="Loading automation sequences" ("Status text")) -> ("error out"=w98:errorcluster)  [unwired: 13 in]
        n32 = call "emi_Splash Update.vi"("error In"=w98, "Task Text"="Implementing stored options" ("Status text")) -> ("error out"=w104:errorcluster)  [unwired: 13 in]
        n33 = call "QSM enque in front.vi"("State"=QSM_State_List."Options updated", "error in"=w104) -> ("error out"=w103:errorcluster)  [unwired: 13 in]
        n34 = call "QSM enque in front.vi"("State"=QSM_State_List."Tool connenction state", "Value"=FALSE, "error in"=w103) -> ("error out"=w102:errorcluster)  [unwired: 12 in]
        n35 = Bundle("Graphs Updated"=w116, "Do motor update"=w99, "Motor voltage"=w100, "P 3.PSU type DO NOT USE"=PSU_Type."None") -> (w115:T59)  [unwired: 1 in]
      }
      frame "Init Reg Controlers" {
        n36 = control-ref of="Controller Temp."() -> (w147:refnum<vi>)
        n37 = control-ref of="Relay Status"() -> (w146:refnum<vi>)
        n38 = control-ref of="Tool Angle"() -> (w149:refnum<vi>)
        n39 = control-ref of="Tool Rotation"() -> (w148:refnum<vi>)
        n40 = control-ref of="Relays off"() -> (w159:refnum<vi>)
        n41 = control-ref of="Relays on"() -> (w117:refnum<vi>)
        n42 = Build Array(w159, w117) -> (w161:refnum<vi>[])
        n43 = Build Array(w149, w148, w147, w146) -> (w150:refnum<vi>[])
        n44 = control-ref of="Upd Default resistance"() -> (w133:refnum<vi>)
        n45 = control-ref of="Calculate resistance"() -> (w130:refnum<vi>)
        n46 = control-ref of="Resistance(Ohm)"() -> (w134:refnum<vi>)
        n47 = control-ref of="Tool voltage setpoint(V)"() -> (w128:refnum<vi>)
        n48 = call "Control refrence holder.vi"("Action(GET)"=enum16{"GET", "SET"}."SET", "Controll collection"=Controll_refrence_groups."Controller Relay Buttons", "Controlls in"=w161) -> ()  [unwired: 11 in, 2 out]
        n49 = call "Control refrence holder.vi"("Action(GET)"=enum16{"GET", "SET"}."SET", "Controll collection"=Controll_refrence_groups."Controller. gen", "Controlls in"=w150) -> ()  [unwired: 11 in, 2 out]
        n50 = Build Array(w128, w134, w133, w130) -> (w132:refnum<vi>[])
        n51 = call "Control refrence holder.vi"("Action(GET)"=enum16{"GET", "SET"}."SET", "Controll collection"=Controll_refrence_groups."PCP Local", "Controlls in"=w132) -> ()  [unwired: 11 in, 2 out]
        n52 = control-ref of="HV ON"() -> (w141:refnum<vi>)
        n53 = Build Array(w141) -> (w139:refnum<vi>[])
        n54 = control-ref of="Annotation Chart"() -> (w124:refnum<vi>)
        n55 = control-ref of="Annotation Tip Strip"() -> (w123:refnum<vi>)
        n56 = call "Control refrence holder.vi"("Action(GET)"=enum16{"GET", "SET"}."SET", "Controll collection"=Controll_refrence_groups."PCP HV On", "Controlls in"=w139) -> ()  [unwired: 11 in, 2 out]
        n57 = control-ref of="HV AV"() -> (w152:refnum<vi>)
        n58 = control-ref of="Topside Bar Graph"() -> (w122:refnum<vi>)
        n59 = control-ref of="Subsea Bar Graph"() -> (w121:refnum<vi>)
        n60 = Bundle(cluster=T44 {"Annotation Chart Ref"=refnum, "Tip Strip Ref"=refnum} ("References in"), "Annotation Chart Ref"=w124, "Tip Strip Ref"=w123) -> (w125:T44)
        n61 = Build Array(w152) -> (w155:refnum<vi>[])
        n62 = Build Array(w122, w121) -> (w119:refnum<vi>[])
        n63 = call "Annotations Tip Strip Ref FGV.vi"("Action(GET)"=T29."SET", "References in"=w125) -> ()  [unwired: 12 in, 2 out]
        n64 = call "Control refrence holder.vi"("Action(GET)"=enum16{"GET", "SET"}."SET", "Controll collection"=Controll_refrence_groups."PCP Online", "Controlls in"=w155) -> ()  [unwired: 11 in, 2 out]
        n65 = control-ref of="Start Motor"() -> (w140:refnum<vi>)
        n66 = Build Array(w140) -> (w142:refnum<vi>[])
        n67 = call "Control refrence holder.vi"("Action(GET)"=enum16{"GET", "SET"}."SET", "Controll collection"=Controll_refrence_groups."Modem Status", "Controlls in"=w119) -> ()  [unwired: 11 in, 2 out]
        n68 = control-ref of="Start Telemetry"() -> (w135:refnum<vi>)
        n69 = call "Control refrence holder.vi"("Action(GET)"=enum16{"GET", "SET"}."SET", "Controll collection"=Controll_refrence_groups."PCP Start Motor", "Controlls in"=w142) -> ()  [unwired: 11 in, 2 out]
        n70 = Build Array(w135) -> (w138:refnum<vi>[])
        n71 = call "Control refrence holder.vi"("Action(GET)"=enum16{"GET", "SET"}."SET", "Controll collection"=Controll_refrence_groups."PCP Start Telemetry", "Controlls in"=w138) -> ()  [unwired: 11 in, 2 out]
      }
      frame "Init Stroker Ref FGV" {
        # "Initialize FGV with stroker control references"
        n72 = control-ref of="Force Zero"() -> (w166:refnum<vi>)
        n73 = control-ref of="Stroker Tension Sub Zero"() -> (w165:refnum<vi>)
        n74 = control-ref of="Stroker Stroke In"() -> (w184:refnum<vi>)
        n75 = control-ref of="Stroker Stroke Out"() -> (w185:refnum<vi>)
        n76 = control-ref of="Stroker Stroke Go To"() -> (w188:refnum<vi>)
        n77 = control-ref of="Stroker Stroke Stop"() -> (w187:refnum<vi>)
        n78 = control-ref of="Stroke Extension"() -> (w174:refnum<vi>)
        n79 = control-ref of="\"Stroke in\" Pressure"() -> (w170:refnum<vi>)
        n80 = control-ref of="\"Stroke out\" Pressure"() -> (w169:refnum<vi>)
        n81 = control-ref of="Stroke force"() -> (w168:refnum<vi>)
        n82 = control-ref of="Upper Tension Sub"() -> (w164:refnum<vi>)
        n83 = control-ref of="Stroker force limit"() -> (w167:refnum<vi>)
        n84 = control-ref of="Stroke setpoint"() -> (w172:refnum<vi>)
        n85 = control-ref of="Stroker"() -> (w173:refnum<vi>)
        n86 = control-ref of="Stroker  2"() -> (w171:refnum<vi>)
        n87 = Build Array(w184, w185, w188, w187) -> (w186:refnum<vi>[])
        n88 = Build Array(w172, w173, w174, w171, w170, w169, w168, w167, w166, w164, w165) -> (w176:refnum<vi>[])
        n89 = call "Control refrence holder.vi"("Action(GET)"=enum16{"GET", "SET"}."SET", "Controll collection"=Controll_refrence_groups."Stroker Cmd Buttons", "Controlls in"=w186) -> ()  [unwired: 11 in, 2 out]
        n90 = call "Control refrence holder.vi"("Action(GET)"=enum16{"GET", "SET"}."SET", "Controll collection"=Controll_refrence_groups."Stroker", "Controlls in"=w176) -> ()  [unwired: 11 in, 2 out]
        n91 = control-ref of="Stroker Anchor in"() -> (w179:refnum<vi>)
        n92 = control-ref of="Stroker Anchor out"() -> (w178:refnum<vi>)
        n93 = Build Array(w179, w178) -> (w182:refnum<vi>[])
        n94 = call "Control refrence holder.vi"("Action(GET)"=enum16{"GET", "SET"}."SET", "Controll collection"=Controll_refrence_groups."Stroker Anchor Cmd Buttons", "Controlls in"=w182) -> ()  [unwired: 11 in, 2 out]
      }
      frame "Init Driller Ref FGV" {
        # "Initialize FGV with driller control references"
        n95 = control-ref of="Driller Anchor out"() -> (w205:refnum<vi>)
        n96 = control-ref of="Driller Anchor in"() -> (w204:refnum<vi>)
        n97 = control-ref of="Driller Stroke in"() -> (w203:refnum<vi>)
        n98 = control-ref of="Driller Stroke out"() -> (w202:refnum<vi>)
        n99 = control-ref of="Driller Oil filling mode"() -> (w198:refnum<vi>)
        n100 = control-ref of="Driller A Dir"() -> (w196:refnum<vi>)
        n101 = control-ref of="Driller Stop"() -> (w194:refnum<vi>)
        n102 = control-ref of="Driller Dir B"() -> (w192:refnum<vi>)
        n103 = control-ref of="Dr Oil filling mode"() -> (w201:refnum<vi>)
        n104 = control-ref of="Drill bit direaction"() -> (w200:refnum<vi>)
        n105 = control-ref of="Weight on drill bit"() -> (w199:refnum<vi>)
        n106 = control-ref of="Torque"() -> (w197:refnum<vi>)
        n107 = control-ref of="RPM"() -> (w195:refnum<vi>)
        n108 = control-ref of="Driller RPM"() -> (w193:refnum<vi>)
        n109 = Build Array(w205, w204, w203, w202, w201, w200, w199, w198, w197, w196, w195, w194, w193, w192) -> (w206:refnum<vi>[])
        n110 = call "Control refrence holder.vi"("Action(GET)"=enum16{"GET", "SET"}."SET", "Controll collection"=Controll_refrence_groups."Driller", "Controlls in"=w206) -> ()  [unwired: 11 in, 2 out]
      }
      frame "Init Tractor Ref FGV" {
        # "Initialize FGV with tractor control references"
        n111 = control-ref of="Tractor Tension Sub Zero"() -> (w213:refnum<vi>)
        n112 = control-ref of="Trac - Upper Tension Sub"() -> (w211:refnum<vi>)
        n113 = control-ref of="Trac - Lower Tension Sub"() -> (w212:refnum<vi>)
        n114 = Build Array(w211, w212, w213) -> (w214:refnum<vi>[])
        n115 = call "Control refrence holder.vi"("Action(GET)"=enum16{"GET", "SET"}."SET", "Controll collection"=Controll_refrence_groups."Tractor", "Controlls in"=w214) -> ()  [unwired: 11 in, 2 out]
      }
      frame "Init All loops" {
        w225 = T24[] [enum."Main-DebugW1", enum."Main-DebugW2", enum."GUI-GrphW Mast", enum."GUI-GrphW Slav", enum."SIM-Tool W1", enum."SIM-Tool W2", enum."Indicator Value Update", enum."Detail View L1", enum."Detail View L2", enum."Interface-PCP", enum."LEIN-motor", enum."Main-Ind Upd", enum."Main-Graph Upd", enum."Var Handling-File storage", enum."Sequence runner", enum."Main-SE Handler", enum."Tool STAT2 dedicated reader", enum."Tool Data LEIN STAT2 dekoder", enum."Var Handling-From PCP", enum."Stroker Wizard L1", enum."Stroker Wizard L2", enum."Alarm Handling", enum."Var Handling-From Simulator", enum."Magna Interface", enum."Modem Status", enum."Var Handling - Modem Status", enum."Power interface detector"] items=["Main-QSM", "Main-Dialog", "Main-Ind Upd", "Main-Graph Upd", "Main-Debug", "Main-DebugW1", "Main-DebugW2", "Main-SE Handler", "Interface-PCP", "Interface-CANbus", "Interface-Modem", "Var Handling-Beat", "Var Handling-From PCP", "Var Handling-File storage", "Var Handling-From Simulator", "GUI-GrphW Mast", "GUI-GrphW Slav", "SIM-Tool W1", "SIM-Tool W2", "Alm-Sound", "LEIN-motor", "Tool data gatherer Qer", "Tool Data LEIN STAT2 dekoder", "Indicator Value Update", "Tool STAT2 dedicated reader", "Tool ID handler", "Detail View L1", "Detail View L2", "Main display enable view", "Sequence runner", "Voltage setpoint", "Resistance setpoint", "Stroker Wizard L1", "Stroker Wizard L2", "Alarm Handling", "Annotations Tip Strip", "Magna Interface", "Modem Status", "Var Handling - Modem Status", "Power interface detector"]  # Loops to not start
        w227 = Loop_ID."Main-QSM" ("Loop ID")
        # "1.1.2"
        # "Spinner igjennom alle looper og initialiserer. Bruker litt tid, slik at loopene får tid på seg"
        # "Legg in logikk her om ikke alt skal initialiseres.(debug f.eks?)"
        # "Options have not been updated until now,"
        # "Inkluderer ikke Feedback da det ikke er problematisk om ikke absolutt alle starter (kanskje ting ikke er koblet til)"
        n116 = call "emi_Splash Update.vi"("error In"=w230, "Task Text"="Initializing sub systems" ("Status text")) -> ("error out"=w226:errorcluster)  [unwired: 13 in]
        n117 = call "emi_Enum Info.vi"("Enum"=w227, "error in (no error)"=w226) -> ("Text Elements"=w228:string[], "Numeric Value"=w224:u64, "error out"=w229:errorcluster)  [unwired: 10 in, 1 out]
        n118 = Quotient & Remainder(x=u64 1000 ("y"), y=w224) -> (floor(x/y)=w222:u64)  [unwired: 1 out]
        n119 = for {
          tunnel: w229 -> [w238]
          tunnel: w228 -> [w243] mode=indexing
          tunnel: w227 -> [w240]
          tunnel: [w239] -> w221
          tunnel: w225 -> [w236]
          tunnel: w222 -> [w233]
          i -> [w241]
          n120 = Variant To Data(error in=w238, type=w240, Variant=w241) -> (data=w235:T24, error out=w237:errorcluster)
          n121 = for {
            tunnel: w236 -> [w246] mode=indexing
            tunnel: w235 -> [w247]
            tunnel: [w245] -> w234
            stop <- w245 stop-if-true
            n122 = Equal?(x=w246, y=w247) -> (x = y?=w245:bool)
          }
          n123 = Concatenate Strings("Initializing sub system: " ("Status text"), w243) -> (w242:string)
          n124 = case shown="False" w234 {
            tunnel: w242 -> [w255 _]
            tunnel: w235 -> [w254 _]
            tunnel: [w251 w256] -> w239
            tunnel: w237 -> [w250 w256]
            tunnel: w233 -> [w248 _]
            frame False {
              n125 = call "emi_Splash Update.vi"("error In"=w250, "Task Text"=w255) -> ("error out"=w249:errorcluster)  [unwired: 13 in]
              n126 = call-poly "emi_SMLoop Control.vi"("Loop ID in"=w254, "Enable"=TRUE, "error in (no error)"=w249) -> ("error out"=w252:errorcluster)  [unwired: 11 in, 1 out]
              n127 = call "emi_Wait MS with err.vi"("milliseconds to wait(0)"=w248, "error in (no error)"=w252) -> ("error out"=w251:errorcluster)  [unwired: 13 in]
            }
            frame True {
              # "Loopen skal ikke auto startes"
            }
          }
        }
        n128 = call "emi_Wait MS with err.vi"("milliseconds to wait(0)"=u32 100, "error in (no error)"=w221) -> ("error out"=w219:errorcluster)  [unwired: 13 in]
      }
      frame "Init Mem Ctls" {
        w258 = FALSE ("Start Motor")
        # "This case initializes some of the controls on the front panel"
        n129 = call "MEM Ctl Holder.vi"("Action(GET)"=T29."GET", "error in (no error)"=w257) -> ("Mem Ctl Out"=w266:T48, "error out"=w271:errorcluster)  [unwired: 12 in]
        n130 = call "Options GFV.vi"("error in (no error)"=w271) -> ("Options"=w273:T60, "error out"=w260:errorcluster)  [unwired: 16 in, 1 out]
        n131 = Unbundle By Name(w266) -> ("Default Resistance(Ohm)"=w272:dbl, "Force Default resistance"=w274:bool, "Sequence user input"=w265:dbl)
        n132 = Unbundle By Name(w273) -> ("P 3.Max resistance"=w270:dbl, "P 3.Min resistance"=w269:dbl)
        n133 = local write "Tool voltage setpoint(V)"(0.0 ("Tool voltage setpoint(V)")) -> ()
        n134 = local write "Start Motor"(w258) -> ()
        n135 = local write "Start Telemetry"(w258) -> ()
        n136 = In Range and Coerce(upper limit=w270, x=w272, lower limit=w269) -> (coerced(x)=w262:dbl)  [unwired: 1 out]
        n137 = local write "Force Default resistance"(w274) -> ()
        n138 = local write "Sequence user input"(w265) -> ()
        n139 = local write "Resistance(Ohm)"(w262) -> ()
        n140 = call "PCP Resistance Setpoint.vi"("Action(GET)"=enum16{"GET", "SET"}."SET", "PCP Res setpoint"=w262) -> ()  [unwired: 12 in, 2 out]
        n141 = property on="Resistance(Ohm)" class="DigNum (strict)"(error in=w260, "NumText.BG Color"=u32 16777216) -> (error out=w259:errorcluster)  [unwired: 1 in, 1 out]
      }
      frame "Init GUI" {
        w295 = T45."Disabled and Grayed Out" ("Disabled")
        # "trengs bare når under Labview"
        n142 = call "emi_Splash Update.vi"("error In"=w300, "Task Text"="Initializing Main GUI" ("Status text")) -> ("error out"=w291:errorcluster)  [unwired: 13 in]
        n143 = call "Enable or Disable PCP controls.vi"("error in (no error)"=w291) -> ("error out"=w290:errorcluster)  [unwired: 14 in]
        n144 = control-ref of="Options"() -> (w299:refnum<vi>)
        n145 = local write "Sequence user input name"("" ("Sequence user input name")) -> ()
        n146 = call "Set contrls enabled disabled.vi"("error in (no error)"=w290) -> ("error out"=w289:errorcluster)  [unwired: 14 in]
        n147 = property on="Sequence user input" class="DigNum (strict)"("Visible"=FALSE) -> ()  [unwired: 2 in, 2 out]
        n148 = property on="Annotation Tip Strip" class="Str"("Visible"=FALSE) -> ()  [unwired: 2 in, 2 out]
        n149 = property class="Bool (strict)"(reference=w299, error in=w289, "DisabledEnum"=T45."Enabled" ("Disabled")) -> (reference out=w296:refnum<vi>, error out=w297:errorcluster)
        n150 = Close Reference(reference=w296, error in (no error)=w297) -> (error out=w277:errorcluster)
        n151 = property on="Approve step" class="Bool (strict)"(error in=w277, "DisabledEnum"=w295) -> (error out=w294:errorcluster)  [unwired: 1 in, 1 out]
        n152 = property on="Stopp sequence" class="Bool (strict)"(error in=w294, "DisabledEnum"=w295) -> (error out=w288:errorcluster)  [unwired: 1 in, 1 out]
        n153 = call "Set pressed button green.vi"("Init"=TRUE, "error in (no error)"=w288, "Controll collection"=Controll_refrence_groups."Stroker Cmd Buttons") -> ("error out"=w287:errorcluster)  [unwired: 8 in]
        n154 = call "Set pressed button green.vi"("Init"=TRUE, "error in (no error)"=w287, "Controll collection"=Controll_refrence_groups."Stroker Anchor Cmd Buttons") -> ("error out"=w281:errorcluster)  [unwired: 8 in]
        n155 = call "Set pressed button green.vi"("Init"=TRUE, "error in (no error)"=w281, "Controll collection"=Controll_refrence_groups."PCP Start Telemetry") -> ("error out"=w280:errorcluster)  [unwired: 8 in]
        n156 = property on="Distance from target:" class="DigNum (strict)"(error in=w280, "Visible"=FALSE) -> (error out=w276:errorcluster)  [unwired: 1 in, 1 out]
      }
      frame "Init<<<End>>>" {
        # "1.3"
        # "En del ulogisk her\nTODO: Welcome en del av splash,\noppdatering under veis)"
        # "Close \nsplash \nscreen"
        n157 = call "emi_Splash Update.vi"("error In"=w317, "Task Text"="Starting Debug interface" ("Status text")) -> ("error out"=w315:errorcluster)  [unwired: 13 in]
        n158 = call "emi_Splash Update.vi"("error In"=w315, "Task Text"="Finalizing initialization" ("Status text")) -> ("error out"=w316:errorcluster)  [unwired: 13 in]
        n159 = call "emi_Splash Update.vi"("error In"=w316, "Task Text"="Displaying GUI" ("Status text")) -> ("error out"=w319:errorcluster)  [unwired: 13 in]
        n160 = call "emi_Splash Close.vi"("Fade time s(0)"=0.0, "error In"=w319) -> ("error out"=w312:errorcluster)  [unwired: 13 in]
        n161 = call "emi_Wait MS with err.vi"("milliseconds to wait(0)"=u32 0, "error in (no error)"=w312) -> ("error out"=w311:errorcluster)  [unwired: 13 in]
        n162 = call "Welcome window.vi"("error in (no error)"=w311) -> ("OK"=w309:bool, "Quick start"=w306:bool, "error out"=w308:errorcluster)  [unwired: 12 in]
        n163 = case shown="True" w309 {
          tunnel: [w326 w332] -> w310
          tunnel: w308 -> [w325 w330]
          tunnel: [w323 w331] -> w307
          tunnel: w306 -> [_ w329]
          frame False {
            w326 = T30[] [enum."End Application"] items=["Idle", "Init <<<Start>>>", "Init Reg Controlers", "Init Stroker Ref FGV", "Init Driller Ref FGV", "Init Tractor Ref FGV", "Init All loops", "Init Mem Ctls", "Init GUI", "Init<<<End>>>", "Show options", "Options updated", "Show User Dialog", "User Updated", "Show About", "Show Help", "Debug Visibility", "End Application", "Mem Ctls", "Mem Graphs", "Post", "-------------", "Dialog Common Analog", "Chart Init", "Chart Var Selector Rings init", "Chart Read Settings from INI", "Chart Clear", "Chart Selection Changed", "Chart Time Changed", "Graph Dialog Show", "Annotation, New", "Annotation Created", "PCP CMD", "Show Welcome screen", "Dialog Tool analog", "Update PCP resistance", "Tool CMD", "Chart single autoscale", "Tool connenction state", "Show detailed view", "Sequences updated", "Show stroker wizard", "Change tool", "Reset Telemetry", "Update control units", "Stop Logging", "Start New Loggfile", "Log Init", "Copy INI files"]
            n164 = call "emi_Splash Update.vi"("error In"=w325, "Task Text"="Application Closed" ("Status text")) -> ("error out"=w323:errorcluster)  [unwired: 13 in]
          }
          frame True {
            n165 = case shown="False" w329 {
              tunnel: w330 -> [w337 w344]
              tunnel: [w333 w344] -> w327
              tunnel: [w334 TRUE ("OK")] -> w328
              frame False {
                n166 = call "Project selector.vi"("error in (no error)"=w337) -> ("OK"=w335:bool, "error out"=w336:errorcluster)  [unwired: 13 in]
                n167 = case shown="True" w335 {
                  selector: w335 -> [w339 _]
                  tunnel: w336 -> [w338 w342]
                  tunnel: [w339 w341] -> w334
                  tunnel: [w338 w340] -> w333
                  frame False {
                  }
                  frame True {
                    n168 = call "COM Port Initial Dialog.vi"("error in (no error)"=w342) -> ("OK"=w341:bool, "error out"=w340:errorcluster)  [unwired: 13 in]
                  }
                }
              }
              frame True {
              }
            }
            n169 = case shown="True" w328 {
              tunnel: [w347 w364] -> w332
              tunnel: [w345 w357] -> w331
              tunnel: w327 -> [w346 w349]
              frame False {
                w347 = T30[] [enum."End Application"] items=["Idle", "Init <<<Start>>>", "Init Reg Controlers", "Init Stroker Ref FGV", "Init Driller Ref FGV", "Init Tractor Ref FGV", "Init All loops", "Init Mem Ctls", "Init GUI", "Init<<<End>>>", "Show options", "Options updated", "Show User Dialog", "User Updated", "Show About", "Show Help", "Debug Visibility", "End Application", "Mem Ctls", "Mem Graphs", "Post", "-------------", "Dialog Common Analog", "Chart Init", "Chart Var Selector Rings init", "Chart Read Settings from INI", "Chart Clear", "Chart Selection Changed", "Chart Time Changed", "Graph Dialog Show", "Annotation, New", "Annotation Created", "PCP CMD", "Show Welcome screen", "Dialog Tool analog", "Update PCP resistance", "Tool CMD", "Chart single autoscale", "Tool connenction state", "Show detailed view", "Sequences updated", "Show stroker wizard", "Change tool", "Reset Telemetry", "Update control units", "Stop Logging", "Start New Loggfile", "Log Init", "Copy INI files"]
                n170 = call "emi_Splash Update.vi"("error In"=w346, "Task Text"="Application Closed" ("Status text")) -> ("error out"=w345:errorcluster)  [unwired: 13 in]
              }
              frame True {
                # "Added 1.3\nTo allow the loops\ntime to start"
                n171 = call "Selected Tool holder.vi"("error in (no error)"=w349) -> ("Tool out"=w356:T56, "error out"=w360:errorcluster)  [unwired: 13 in]
                n172 = To Unsigned Word Integer(number=w356) -> (unsigned 16bit integer=→"Type tab 1" →"Type tab 2" →"Type tab 3":u16)
                n173 = call "Start Processes.vi"("error in (no error)"=w360) -> ("error out"=w361:errorcluster)  [unwired: 10 in]
                n174 = call "emi_Wait MS with err.vi"("milliseconds to wait(0)"=u32 100, "error in (no error)"=w361) -> ("error out"=w362:errorcluster)  [unwired: 13 in]
                n175 = call "emi_FP Show.vi"("error in (no error)"=w362) -> ("error out"=w358:errorcluster)  [unwired: 13 in, 1 out]
                n176 = call <vilib>:"Unset Busy.vi"() -> ("error out"=w359:errorcluster)  [unwired: 11 in]
                n177 = Merge Errors(w358, w359) -> (w357:errorcluster)
                n178 = Build Array(QSM_State_List."Log Init" ("element"), QSM_State_List."Chart Init" ("element"), QSM_State_List."Sequences updated" ("element"), QSM_State_List."Options updated" ("State"), QSM_State_List."User Updated" ("State"), QSM_State_List."Update control units" ("State")) -> (w364:T30[])
              }
            }
          }
        }
        n179 = for {
          tunnel: w307 -> [w368]
          tunnel: [w367] -> w303
          tunnel: w310 -> [w366] mode=indexing
          n180 = call "QSM enque in front.vi"("State"=w366, "error in"=w368) -> ("error out"=w367:errorcluster)  [unwired: 13 in]
        }
        n181 = call "emi_Wait MS with err.vi"("milliseconds to wait(0)"=u32 50, "error in (no error)"=w303) -> ("error out"=w304:errorcluster)  [unwired: 13 in]
      }
      frame "Show options" {
        n182 = call "Dialog Selector SIC.vi"("error in (no error)"=w370) -> ("Dialog Selector Q"=w372:refnum<queue>, "error out"=w373:errorcluster)  [unwired: 13 in]
        n183 = Enqueue Element At Opposite End(queue=w372, element=T46 {"ID"=enum."Options dialog box", "Details"=variant}, error in (no error)=w373) -> (error out=w369:errorcluster)  [unwired: 1 in, 2 out]
      }
      frame "Options updated" {
        w382 = u32 700  # Reply timeout
        w386 = 0.0 ("Scale.Range:Minimum")
        n184 = call "Options GFV.vi"("error in (no error)"=w404, "Action(Get Settings)"=Action_GFV_Settings."Get Settings") -> ("Options"=w376:T60, "error out"=w401:errorcluster)  [unwired: 15 in, 1 out]
        n185 = Unbundle By Name(w376) -> ("P 1 (App).PCP Interface"=w400:string, "P 3.Max resistance"=w394:dbl, "P 3.Min resistance"=w393:dbl, "P 3.Head voltage range"=w390:T64)
        n186 = Unbundle By Name(w376) -> ("P 7 (Expert).Modem baud"=w383:u16, "P 7 (Expert).Modem sim"=w384:T73)
        n187 = call "Selected Tool holder.vi"() -> ("Tool out"=w381:T56)  [unwired: 14 in, 1 out]
        n188 = Unbundle By Name(w376) -> ("P 1 (App).Modem Status Interface"=w375:string)
        n189 = case shown="\"Tractor\"" w381 {
          tunnel: w376 -> [w407 w409]
          tunnel: [w406 w408] -> w380
          frame "Stroker", Default {
            n190 = Unbundle By Name(w407) -> ("P 1 (App).Tractor/Stroker Interface"=w406:string)
          }
          frame "Tractor" {
            n191 = Unbundle By Name(w409) -> ("P 1 (App).Tractor/Stroker Interface"=w408:string)
          }
        }
        n192 = call "PCP Interface settings.vi"("Action(GET)"=enum16{"GET", "SET"}."SET", "PCP VISA  name  in"=w400, "error in (no error)"=w401) -> ("error out"=w396:errorcluster)  [unwired: 11 in, 1 out]
        n193 = call "LEIN m serial Interface settings.vi"("baud rate"=w383, "Action(GET)"=enum16{"GET", "SET"}."SET", "Reply timeout"=w382, "LEIN m serial VISA  name  in"=w380, "Modem sim in"=w384, "error in (no error)"=w396) -> ("error out"=w379:errorcluster)  [unwired: 4 in, 5 out]
        n194 = local read "Tool voltage setpoint(V)"() -> (w387:dbl)
        n195 = call "Modem Status Interface settings.vi"("Action(GET)"=enum16{"GET", "SET"}."SET", "Modem Status VISA  name  in"=w375, "error in (no error)"=w379) -> ("error out"=w378:errorcluster)  [unwired: 10 in, 2 out]
        n196 = local read "Resistance(Ohm)"() -> (w392:dbl)
        n197 = call "PCP ype to max range.vi"("PCP/PSU range"=w390) -> ("Scale.Range:Maximum"=w388:dbl)  [unwired: 14 in]
        n198 = property on="Tool voltage setpoint(V)" class="Slide (strict)"(error in=w378, "Maximum"=w388, "Scale.Maximum"=w388, "Minimum"=w386, "Scale.Minimum"=w386) -> (error out=w389:errorcluster)  [unwired: 1 in, 1 out]
        n199 = In Range and Coerce(upper limit=w388, x=w387, lower limit=w386) -> (coerced(x)=w385:dbl)  [unwired: 1 out]
        n200 = In Range and Coerce(upper limit=w394, x=w392, lower limit=w393) -> (coerced(x)=w391:dbl)  [unwired: 1 out]
        n201 = local write "Tool voltage setpoint(V)"(w385) -> ()
        n202 = local write "Resistance(Ohm)"(w391) -> ()
        n203 = Build Array(QSM_State_List."Debug Visibility" ("State")) -> (w398:T30[])
        n204 = for {
          tunnel: w389 -> [w412]
          tunnel: [w411] -> w397
          tunnel: w398 -> [w410] mode=indexing
          n205 = call "QSM enque.vi"("State"=w410, "error in"=w412) -> ("error out"=w411:errorcluster)  [unwired: 13 in]
        }
      }
      frame "Show User Dialog" {
        n206 = call "Dialog Selector SIC.vi"("error in (no error)"=w414) -> ("Dialog Selector Q"=w416:refnum<queue>, "error out"=w417:errorcluster)  [unwired: 13 in]
        n207 = Enqueue Element At Opposite End(queue=w416, element=T46 {"ID"=enum."User dialog Box", "Details"=variant}, error in (no error)=w417) -> (error out=w413:errorcluster)  [unwired: 1 in, 2 out]
      }
      frame "User Updated" {
        # "Disable controls if not superuser"
        # "Chart has to be updated with the channels\nvalid for that user. \n\nA superuser can change channels\non the fly, whereas a normal user has a fixed\ngraph selection"
        n208 = call "User GFV ini.vi"("Action(GET)"=T29."GET", "error in (no error)"=w440) -> ("User ID out"=w430:T22, "error out"=w424:errorcluster)  [unwired: 12 in]
        "User ID" <- w430
        n209 = Unbundle By Name(w430) -> ("Super User"=w428:T23)
        n210 = control-ref of="Plot G1 L1"() -> (w438:refnum<vi>)
        n211 = control-ref of="Plot G1 L2"() -> (w437:refnum<vi>)
        n212 = control-ref of="Plot G1 R1"() -> (w436:refnum<vi>)
        n213 = control-ref of="Plot G1 R2"() -> (w435:refnum<vi>)
        n214 = control-ref of="Plot G2 L1"() -> (w434:refnum<vi>)
        n215 = control-ref of="Plot G2 L2"() -> (w433:refnum<vi>)
        n216 = control-ref of="Plot G2 R1"() -> (w432:refnum<vi>)
        n217 = control-ref of="Plot G2 R2"() -> (w431:refnum<vi>)
        n218 = Select(t=T45."Enabled" ("Disabled"), s=w428, f=T45."Disabled" ("Disabled")) -> (s? t:f=w425:T45)
        n219 = Build Array(w438, w437, w436, w435, w434, w433, w432, w431) -> (w429:refnum<vi>[])
        n220 = for {
          tunnel: w429 -> [w448] mode=indexing
          tunnel: w425 -> [w447]
          shift-right: [w446] -> w420
          shift-left: w424 -> [w445]
          n221 = property class="Clust (strict)"(reference=w448, error in=w445, "DisabledEnum"=w447) -> (error out=w446:errorcluster)  [unwired: 1 out]
        }
        n222 = Build Array(QSM_State_List."Chart Read Settings from INI" ("State"), QSM_State_List."Chart Selection Changed" ("State")) -> (w421:T30[])
        n223 = for {
          tunnel: w421 -> [w442] mode=indexing
          shift-right: [w444] -> w419
          shift-left: w420 -> [w443]
          n224 = call "QSM enque.vi"("State"=w442, "error in"=w443) -> ("error out"=w444:errorcluster)  [unwired: 13 in]
        }
      }
      frame "Show About" {
        n225 = call "Dialog Selector SIC.vi"("error in (no error)"=w453) -> ("Dialog Selector Q"=w451:refnum<queue>, "error out"=w452:errorcluster)  [unwired: 13 in]
        n226 = Enqueue Element At Opposite End(queue=w451, element=T46 {"ID"=enum."About dialog Box", "Details"=variant}, error in (no error)=w452) -> (error out=w449:errorcluster)  [unwired: 1 in, 2 out]
      }
      frame "Show Help" {
        # "Lag en egen en for dette"
        n227 = Variant To Data(type="", Variant=w460) -> (data=w456:string, error out=w457:errorcluster)  [unwired: 1 in]
        n228 = case shown="No Error" w457 {
          selector: w457 -> [_ w464]
          tunnel: w456 -> [w463 _]
          tunnel: [w463 _] -> w455
          frame No Error {
          }
          frame Error {
            n229 = call <vilib>:"Clear Errors.vi"("error in (no error)"=w464) -> ()  [unwired: 6 in, 1 out]
          }
        }
        n230 = call "Open App Help file.vi"("Help Tag (\"\")"=w455, "error In"=w458) -> ("error out"=w461:errorcluster)  [unwired: 13 in]
      }
      frame "Debug Visibility" {
        n231 = call "emi_Get Debug Disp status.vi"("error in (no error)"=w469) -> ("Debug Disp"=w466:bool, "error out"=w468:errorcluster)  [unwired: 13 in]
        n232 = call-poly "emi_SMLoop Control.vi"("Loop ID in"=Loop_ID."Main-DebugW1" ("Loop ID"), "Enable"=w466, "error in (no error)"=w468) -> ("error out"=w467:errorcluster)  [unwired: 11 in, 1 out]
      }
      frame "End Application" {
        w487 = u32 1000  # ms
        # "Do not need to send when Magna is used\nthis is handled by the process"
        # "Send PSU Shutdown command and\ngive time for completion of the command\nbefore all the loops are terminated"
        # "Perform aditional \nend tasks here.\nApplication will be ended in post"
        n233 = call "PCP Last data GFV.vi"("Action(GET)"=enum16{"GET", "SET"}."GET", "error in (no error)"=w480) -> ("ms since last data"=w488:u32, "PCP Data out"=w486:T77, "error out"=w485:errorcluster)  [unwired: 11 in]
        n234 = call "PSU interface to use GFV.vi"() -> ("PSU type  out"=w471:T41)  [unwired: 14 in, 1 out]
        n235 = Unbundle By Name(w486) -> ("Digital ports.DO -  HVPSU HV On"=w475:bool)
        n236 = Less?(x=w488, y=w487) -> (x < y?=w476:bool)
        n237 = Equal?(x=w471, y=PSU_Type."Unipower") -> (x = y?=w474:bool)
        n238 = Compound Arithmetic op=AND(w474, w476, w475) -> (w473:bool)
        n239 = case shown="True" w473 {
          tunnel: w485 -> [w496 w499]
          tunnel: [w496 w497] -> w479
          tunnel: w471 -> [_ w498]
          frame False {
          }
          frame True {
            n240 = call "PCP OFF With the Power.vi"("PSU type"=w498, "error In"=w499) -> ("error out"=w497:errorcluster)  [unwired: 13 in]
          }
        }
        n241 = call "emi_Window Store Position in Ini.vi"("error in (no error)"=w479) -> ("error out"=w494:errorcluster)  [unwired: 13 in, 1 out]
        n242 = call "emi_Defer Panel Updates ON(w.cursor).vi"("error in (no error)"=w494) -> ("error out"=w495:errorcluster)  [unwired: 13 in, 1 out]
        n243 = call "emi_Close all Loops.vi"("error in (no error)"=w495) -> ("error out"=w478:errorcluster)  [unwired: 14 in]
        n244 = call "QSM enque.vi"("State"=QSM_State_List."Copy INI files", "error in"=w478) -> ("error out"=w481:errorcluster)  [unwired: 13 in]
        n245 = call "QSM enque.vi"("State"=QSM_State_List."Mem Graphs", "error in"=w481) -> ("error out"=w483:errorcluster)  [unwired: 13 in]
        n246 = call "QSM enque.vi"("State"=QSM_State_List."Mem Ctls", "error in"=w483) -> ("error out"=w490:errorcluster)  [unwired: 13 in]
        n247 = call "QSM enque.vi"("State"=QSM_State_List."Post", "error in"=w490) -> ("error out"=w493:errorcluster)  [unwired: 13 in]
      }
      frame "Mem Ctls" {
        # "Write settings to INI file when shutting down. \nSettings will be remembered at next startup"
        n248 = local read "Tool voltage setpoint(V)"() -> (w506:dbl)
        n249 = local read "Force Default resistance"() -> (w504:bool)
        n250 = local read "Sequence user input"() -> (w502:dbl)
        n251 = local read "Resistance(Ohm)"() -> (w505:dbl)
        n252 = Bundle By Name(cluster=T48 {"Tool Voltage  SP"=0.0, "Default Resistance(Ohm)"=0.0, "Force Default resistance"=FALSE, "Upd Default resistance"=FALSE, "Sequence user input"=1.0} ("Mem Ctl In"), "Tool Voltage  SP"=w506, "Default Resistance(Ohm)"=w505, "Force Default resistance"=w504, "Upd Default resistance"=FALSE, "Sequence user input"=w502) -> (w501:T48)
        n253 = call "MEM Ctl Holder.vi"("Action(GET)"=T29."SET", "Mem Ctl In"=w501, "error in (no error)"=w500) -> ("error out"=w510:errorcluster)  [unwired: 11 in, 1 out]
        n254 = call "MEM Ctl Holder.vi"("Action(GET)"=T29."Put in Ini", "error in (no error)"=w510) -> ("error out"=w508:errorcluster)  [unwired: 12 in, 1 out]
      }
      frame "Mem Graphs" {
        # "Writes the graph configuration to INI file if Super user"
        n255 = Unbundle By Name(w516) -> ("Graphs Updated"=w515:bool)
        n256 = call "User GFV ini.vi"("Action(GET)"=T29."GET", "error in (no error)"=w518) -> ("User ID out"=w519:T22, "error out"=w517:errorcluster)  [unwired: 12 in]
        n257 = Unbundle(w519) -> ("Super User"=w514:T23)  [unwired: 1 out]
        n258 = And(x=w515, y=w514) -> (x .and. y?=w513:T23)
        n259 = case shown="True" w513 {
          tunnel: [w522 w525] -> w521
          tunnel: w517 -> [w522 w524]
          frame False {
          }
          frame True {
            w547 = 1 ("Active Y Scale")
            w546 = 0 ("Active Y Scale")
            n260 = control-ref of="Chart 2"() -> (w548:refnum<vi>)
            n261 = control-ref of="Chart 1"() -> (w549:refnum<vi>)
            n262 = Build Array(w549, w549, w548, w548) -> (w545:refnum<vi>[])
            n263 = Build Array(w546, w547, w546, w547) -> (w544:i32[])
            n264 = local read "Chart Visible Time selector"() -> (w540:T21)
            n265 = for {
              shift-right: [w554] -> w523
              shift-left: w524 -> [w555]
              tunnel: [w553] -> w550 mode=indexing
              tunnel: w545 -> [w552] mode=indexing
              tunnel: w544 -> [w551] mode=indexing
              n266 = call "Graph Get Y scale Settings.vi"("error in (no error)"=w555, "Active Y Scale"=w551, "Chart Ref"=w552) -> ("error out"=w554:errorcluster, "Y scale"=w553:T50)  [unwired: 7 in]
            }
            n267 = local read "Plot G1 R1"() -> (w535:T20)
            n268 = local read "Plot G1 R2"() -> (w534:T20)
            n269 = local read "Plot G2 R1"() -> (w531:T20)
            n270 = local read "Plot G2 R2"() -> (w530:T20)
            n271 = local read "Plot G1 L1"() -> (w537:T20)
            n272 = local read "Plot G1 L2"() -> (w536:T20)
            n273 = local read "Plot G2 L1"() -> (w533:T20)
            n274 = local read "Plot G2 L2"() -> (w532:T20)
            n275 = Index Array(array=w550) -> (element #1=w529:T50, element #2=w528:T50, element #3=w527:T50, element #4=w526:T50)  [unwired: 4 in]
            n276 = Bundle By Name(cluster=T49 {"Chart Visible Time selector"=enum."1 minute", "Plot G1 L1"={"Var Tag"=0, "Color"=0, "Line Width"=0}, "Plot G1 L2"={"Var Tag"=0, "Color"=0, "Line Width"=0}, "Plot G1 R1"={"Var Tag"=0, "Color"=0, "Line Width"=0}, "Plot G1 R2"={"Var Tag"=0, "Color"=0, "Line Width"=0}, "Plot G2 L1"={"Var Tag"=0, "Color"=0, "Line Width"=0}, "Plot G2 L2"={"Var Tag"=0, "Color"=0, "Line Width"=0}, "Plot G2 R1"={"Var Tag"=0, "Color"=0, "Line Width"=0}, "Plot G2 R2"={"Var Tag"=0, "Color"=0, "Line Width"=0}, "G1 Y scale 0"={"Maximum"=0.0, "Minimum"=0.0, "Autoscaling"=0}, "G1 Y scale 1"={"Maximum"=0.0, "Minimum"=0.0, "Autoscaling"=0}, "G2 Y scale 0"={"Maximum"=0.0, "Minimum"=0.0, "Autoscaling"=0}, "G2 Y scale 1"={"Maximum"=0.0, "Minimum"=0.0, "Autoscaling"=0}} ("Mem Graph Ctl In"), "Chart Visible Time selector"=w540, "Plot G1 L1"=w537, "Plot G1 L2"=w536, "Plot G1 R1"=w535, "Plot G1 R2"=w534, "Plot G2 L1"=w533, "Plot G2 L2"=w532, "Plot G2 R1"=w531, "Plot G2 R2"=w530, "G1 Y scale 0"=w529, "G1 Y scale 1"=w528, "G2 Y scale 0"=w527, "G2 Y scale 1"=w526) -> (w538:T49)
            n277 = call "MEM Graph Holder.vi"("Action(GET)"=T29."SET", "Mem Graph Ctl In"=w538, "error in (no error)"=w523) -> ("error out"=w541:errorcluster)  [unwired: 11 in, 1 out]
            n278 = call "MEM Graph Holder.vi"("Action(GET)"=T29."Put in Ini", "error in (no error)"=w541) -> ("error out"=w525:errorcluster)  [unwired: 12 in, 1 out]
          }
        }
      }
      frame "Post" {
        n279 = Build Array(Loop_ID."Main-QSM" ("Loop ID"), Loop_ID."Main-SE Handler" ("element")) -> (w561:T24[])
        n280 = call "emi_Wait for loops to stop.vi"("Loop exlusion[0,..]"=w561, "Timeout ms(5000)"=5000, "error in (no error)"=w559) -> ("error out"=w558:errorcluster)  [unwired: 12 in]
        n281 = call "emi_Defer Panel Updates OFF(w.cursor).vi"("error in (no error)"=w558) -> ("error out"=w557:errorcluster)  [unwired: 13 in, 1 out]
        n282 = call "emi_Close Application.vi"("error in (no error)"=w557) -> ("error out"=w556:errorcluster)  [unwired: 14 in]
      }
      frame "-------------" {
        # "Do not add code\nShould never be called"
      }
      frame "Dialog Common Analog" {
        n283 = call "Dialog Selector SIC.vi"("error in (no error)"=w571) -> ("Dialog Selector Q"=w569:refnum<queue>, "error out"=w570:errorcluster)  [unwired: 13 in]
        n284 = Enqueue Element At Opposite End(queue=w569, element=T46 {"ID"=enum."Variables Common Analog", "Details"=variant}, error in (no error)=w570) -> (error out=w567:errorcluster)  [unwired: 1 in, 2 out]
      }
      frame "Chart Init" {
        # "2014-06-16 OOS: This case is only called once now. Maybe it should be removed."
        # "This case calls all tasks that are necessary to initialize the charts\nThis case should be called when initializing, changing user, or changing tool"
        n285 = Build Array(QSM_State_List."Chart Var Selector Rings init" ("State"), QSM_State_List."Chart Read Settings from INI" ("State"), QSM_State_List."Chart Clear" ("State"), QSM_State_List."Chart Selection Changed" ("State")) -> (w576:T30[])
        n286 = for {
          tunnel: w578 -> [w583]
          tunnel: [w582] -> w577
          tunnel: w576 -> [w581] mode=indexing
          n287 = call "QSM enque.vi"("State"=w581, "error in"=w583) -> ("error out"=w582:errorcluster)  [unwired: 13 in]
        }
      }
      frame "Chart Var Selector Rings init" {
        # "#temp"
        # "This case initializes the Variable Selectors for the plots with the channel names\nThe charts are initiated with one plot for each channel"
        n288 = call "Get Channel List.vi"("Force all(F)"=FALSE, "error in"=w609) -> ("Numb Elements"=w594:i32, "Names"=w597:string[], "Ring list"=w586:cluster{"String":string, "Value":u16}[], "error out"=w607:errorcluster)  [unwired: 9 in, 1 out]
        n289 = control-ref of="Var Tag"() -> (w590:refnum<vi>)
        n290 = control-ref of="Var Tag"() -> (w589:refnum<vi>)
        n291 = control-ref of="Var Tag"() -> (w588:refnum<vi>)
        n292 = control-ref of="Var Tag"() -> (w587:refnum<vi>)
        n293 = control-ref of="Var Tag"() -> (w593:refnum<vi>)
        n294 = control-ref of="Var Tag"() -> (w592:refnum<vi>)
        n295 = control-ref of="Var Tag"() -> (w602:refnum<vi>)
        n296 = control-ref of="Var Tag"() -> (w601:refnum<vi>)
        n297 = Build Array (concatenate)(cluster{"String":string, "Value":i32} {"String"="", "Value"=0}, w586) -> (w604:cluster{"String":string, "Value":i32}[])
        n298 = Build Array(w590, w589, w588, w587, w593, w592, w602, w601) -> (w603:refnum<vi>[])
        n299 = for {
          tunnel: w607 -> [w629]
          tunnel: w604 -> [w625]
          tunnel: w603 -> [w626] mode=indexing
          tunnel: [w628] -> w606
          tunnel: [w627] -> w605 mode=indexing
          (unwired) u16 0 ("Value")
          # "1.4. Val = 0 removed"
          n300 = property class="Ring (strict)"(reference=w626, error in=w629, "StringsAndValues[]"=w625) -> (reference out=w627:refnum<vi>, error out=w628:errorcluster)
        }
        n301 = control-ref of="Chart 1"() -> (w600:refnum<vi>)
        n302 = control-ref of="Chart 2"() -> (w591:refnum<vi>)
        n303 = Build Array(w600, w591) -> (w598:refnum<vi>[])
        n304 = Close Reference(reference=w605, error in (no error)=w606) -> (error out=w599:errorcluster)
        n305 = for {
          tunnel: w599 -> [w615]
          tunnel: w598 -> [w614] mode=indexing
          tunnel: [w618] -> w596
          tunnel: [w617] -> w595 mode=indexing
          tunnel: w597 -> [w616]
          tunnel: w594 -> [w611]
          n306 = property class="WFChart (strict)"(reference=w614, error in=w615, "LegPlotMin"=w611) -> (reference out=w612:refnum<vi>, error out=w613:errorcluster)
          n307 = for {
            tunnel: w613 -> [w624]
            tunnel: [w623] -> w618
            tunnel: [w622] -> w617
            tunnel: w612 -> [w621]
            tunnel: w616 -> [w619] mode=indexing
            i -> [w620]
            (unwired) FALSE ("Plot.Visible")
            n308 = property class="WFChart (strict)"(reference=w621, error in=w624, "Active Plot"=w620, "Plot.Plot Name"=w619) -> (reference out=w622:refnum<vi>, error out=w623:errorcluster)
          }
        }
        n309 = Close Reference(reference=w595, error in (no error)=w596) -> (error out=w608:errorcluster)
      }
      frame "Chart Read Settings from INI" {
        w640 = 1 ("Active Y Scale")
        w639 = 0 ("Active Y Scale")
        # "v1.17.0 2015-09-10\nRead from INI has been\nmoved to the earlier init\ncases to ensure that the\nold settings are remembered\nwhen the operator presses\nEXIT in the config dialogs"
        # "Super user"
        # "Normal user"
        # "This case initializes the graphs with selected channels and Y-axis values.\nIf a superuser is logged in, the last graph settings that were used for the selected tools is loaded\nIf a normal user is logged in, the default graph configuration is loaded"
        n310 = call "User GFV ini.vi"("Action(GET)"=T29."GET") -> ("User ID out"=w655:T22)  [unwired: 13 in, 1 out]
        n311 = call "Normal User Default Chart holder FGV.vi"("Action(GET)"=T29."GET", "error in (no error)"=w631) -> ("Mem Ctl Out"=w653:T80, "error out"=w630:errorcluster)  [unwired: 12 in]
        n312 = Unbundle(w655) -> ("Super User"=w654:T23)  [unwired: 1 out]
        n313 = call "MEM Graph Holder.vi"("Action(GET)"=T29."GET", "error in (no error)"=w630) -> ("Mem Graph Ctl Out"=w633:T49, "error out"=w632:errorcluster)  [unwired: 12 in]
        n314 = Unbundle By Name(w633) -> ("Chart Visible Time selector"=w661:T21, "G1 Y scale 0"=w659:T50, "G1 Y scale 1"=w660:T50, "G2 Y scale 0"=w644:T50, "G2 Y scale 1"=w643:T50)
        n315 = case shown="True" w654 {
          tunnel: w633 -> [_ w684]
          tunnel: w653 -> [w675 _]
          tunnel: [w674 w683] -> w652
          tunnel: [w673 w682] -> w651
          tunnel: [w672 w681] -> w650
          tunnel: [w671 w680] -> w649
          tunnel: [w670 w679] -> w648
          tunnel: [w669 w678] -> w647
          tunnel: [w668 w677] -> w646
          tunnel: [w667 w676] -> w645
          frame False {
            n316 = Unbundle By Name(w675) -> ("UL1"=w674:T20, "UL2"=w673:T20, "UR1"=w672:T20, "UR2"=w671:T20, "LL1"=w670:T20, "LL2"=w669:T20, "LR1"=w668:T20, "LR2"=w667:T20)
          }
          frame True {
            n317 = Unbundle By Name(w684) -> ("Plot G1 L1"=w683:T20, "Plot G1 L2"=w682:T20, "Plot G1 R1"=w681:T20, "Plot G1 R2"=w680:T20, "Plot G2 L1"=w679:T20, "Plot G2 L2"=w678:T20, "Plot G2 R1"=w677:T20, "Plot G2 R2"=w676:T20)
          }
        }
        n318 = local write "Chart Visible Time selector"(w661) -> ()
        n319 = local write "Plot G1 L1"(w652) -> ()
        n320 = local write "Plot G1 L2"(w651) -> ()
        n321 = local write "Plot G1 R1"(w650) -> ()
        n322 = local write "Plot G1 R2"(w649) -> ()
        n323 = local write "Plot G2 L1"(w648) -> ()
        n324 = local write "Plot G2 L2"(w647) -> ()
        n325 = local write "Plot G2 R1"(w646) -> ()
        n326 = local write "Plot G2 R2"(w645) -> ()
        n327 = Build Array(w659, w660, w644, w643) -> (w637:T50[])
        n328 = control-ref of="Chart 1"() -> (w642:refnum<vi>)
        n329 = control-ref of="Chart 2"() -> (w641:refnum<vi>)
        n330 = Build Array(w642, w642, w641, w641) -> (w635:refnum<vi>[])
        n331 = Build Array(w639, w640, w639, w640) -> (w636:i32[])
        n332 = for {
          shift-right: [w666] -> w638
          shift-left: w632 -> [w665]
          tunnel: w637 -> [w664] mode=indexing
          tunnel: w636 -> [w663] mode=indexing
          tunnel: w635 -> [w662] mode=indexing
          n333 = call "Graph Initialize Y scale.vi"("error in (no error)"=w665, "Y scale"=w664, "Active Y Scale"=w663, "Chart Ref"=w662) -> ("error out"=w666:errorcluster)  [unwired: 7 in]
        }
      }
      frame "Chart Clear" {
        w689 = 0.2 ("X Scale.Offset and Multiplier:Multiplier")
        # "Set annotation chart properties"
        # "Clears chart and sets correct timing"
        n334 = local read "Chart Visible Time selector"() -> (w691:T21)
        n335 = feedback #1(0) -> (w696:i32)
        n336 = Increment(x=w696) -> (x+1=w694:i32)
        n337 = feedback-in #1(w694) -> ()
        n338 = control-ref of="Annotation Chart"() -> (w697:refnum<vi>)
        n339 = control-ref of="Chart 1"() -> (w703:refnum<vi>)
        n340 = control-ref of="Chart 2"() -> (w702:refnum<vi>)
        n341 = case shown="\"1 Hour\"" w691 {
          tunnel: [10.0 ("X Scale.Range:Maximum") 60.0 ("X Scale.Range:Maximum") 300.0 ("X Scale.Range:Maximum") 600.0 ("X Scale.Range:Maximum") 1800.0 ("X Scale.Range:Maximum") 3600.0 ("X Scale.Range:Maximum")] -> w692
          frame "10 Seconds" {
          }
          frame "1 minute" {
          }
          frame "5 minutes" {
          }
          frame "10 minutes" {
          }
          frame "30 minutes" {
          }
          frame "1 Hour" {
          }
        }
        n342 = Get Date/Time In Seconds() -> (seconds since 1Jan1904=w701:timestamp)
        n343 = Build Array(w703, w702) -> (w700:refnum<vi>[])
        n344 = To Double Precision Float(number=w701) -> (double precision float=w688:dbl)
        n345 = Add(x=w688, y=w692) -> (x+y=w690:dbl)
        n346 = for {
          tunnel: w704 -> [w720]
          tunnel: [w718] -> w693
          tunnel: w700 -> [w716] mode=indexing
          tunnel: dbl[][] [] ("initialized array") -> [w715]
          tunnel: w690 -> [w714]
          tunnel: w688 -> [w713]
          tunnel: w689 -> [w712]
          n347 = property class="WFChart (strict)"(reference=w716, error in=w720, "History Data"=w715, "XScale.Offset"=w713, "XScale.Multiplier"=w712, "XScale.Minimum"=w713, "XScale.RngStart"=w713, "XScale.Maximum"=w714) -> (reference out=w717:refnum<vi>, error out=w719:errorcluster)
          n348 = Close Reference(reference=w717, error in (no error)=w719) -> (error out=w718:errorcluster)
        }
        n349 = property class="WFChart (strict)"(reference=w697, error in=w693, "History Data"=dbl[] [] ("initialized array"), "XScale.Offset"=w688, "XScale.Multiplier"=w689, "XScale.Minimum"=w688, "XScale.RngStart"=w688, "XScale.Maximum"=w690) -> (reference out=w699:refnum<vi>, error out=w698:errorcluster)
        n350 = Close Reference(reference=w699, error in (no error)=w698) -> (error out=w687:errorcluster)
      }
      frame "Chart Selection Changed" {
        w737 = u32 1 ("element")
        w740 = u32 0  # y scale
        # "Loads selected channels into plot"
        n351 = call "Get Channel List.vi"("error in"=w745) -> ("Numb Elements"=w743:i32, "error out"=w724:errorcluster)  [unwired: 10 in, 3 out]
        n352 = control-ref of="Chart 1"() -> (w744:refnum<vi>)
        n353 = control-ref of="Chart 2"() -> (w735:refnum<vi>)
        n354 = Build Array(w740, w740, w737, w737) -> (w726:u32[])
        n355 = Build Array("Plot G1 L1", "Plot G1 L2", "Plot G1 R1", "Plot G1 R2") -> (w732:T20[])
        n356 = Build Array("Plot G2 L1", "Plot G2 L2", "Plot G2 R1", "Plot G2 R2") -> (w731:T20[])
        n357 = Build Array(w726, w726) -> (w734:u32[][])
        n358 = Build Array(w744, w735) -> (w736:refnum<vi>[])
        n359 = Build Array(w732, w731) -> (w733:T20[][])
        n360 = for {
          tunnel: w736 -> [w756] mode=indexing
          tunnel: w724 -> [w755]
          tunnel: w743 -> [w754]
          tunnel: w733 -> [w751] mode=indexing
          tunnel: w734 -> [w750] mode=indexing
          tunnel: [w748] -> w725
          tunnel: [w746] -> _ mode=indexing
          i -> [w746]
          n361 = for {
            N: w754 -> [_]
            shift-right: [w783] -> w752
            shift-left: w755 -> [w782]
            shift-right: [w781] -> w753
            shift-left: w756 -> [w784]
            i -> [w780]
            n362 = property class="WFChart (strict)"(reference=w784, error in=w782, "Plot.Visible?"=FALSE ("Plot.Visible"), "Active Plot"=w780) -> (reference out=w781:refnum<vi>, error out=w783:errorcluster)
          }
          n363 = for {
            tunnel: w751 -> [w762] mode=indexing
            tunnel: w750 -> [w759] mode=indexing
            tunnel: [w758] -> _ mode=indexing
            shift-right: [w763] -> w747
            shift-left: w753 -> [w766]
            shift-right: [w765] -> w749
            shift-left: w752 -> [w764]
            i -> [w758]
            n364 = Unbundle(w762) -> ("Var Tag"=w761:u16, "Color"=w760:u32, "Line Width"=w757:u16)
            n365 = case shown="1, Default" w761 {
              selector: w761 -> [_ w773]
              tunnel: w766 -> [w768 w778]
              tunnel: [w767 w777] -> w765
              tunnel: w764 -> [w767 w776]
              tunnel: [w768 w775] -> w763
              tunnel: w760 -> [_ w771]
              tunnel: w759 -> [_ w770]
              tunnel: w757 -> [_ w769]
              frame 0 {
              }
              frame 1, Default {
                n366 = Decrement(x=w773) -> (x-1=w774:u16)
                n367 = property class="WFChart (strict)"(reference=w778, error in=w776, "Active Plot"=w774, "Plot.Visible?"=TRUE ("Plot.Visible"), "Plot.Plot Color"=w771, "Plot.YScaleIdx"=w770, "Plot.Line Width"=w769) -> (reference out=w775:refnum<vi>, error out=w777:errorcluster)
              }
            }
          }
          n368 = Close Reference(reference=w747, error in (no error)=w749) -> (error out=w748:errorcluster)
        }
        n369 = Bundle By Name(cluster=w723, "Graphs Updated"=TRUE) -> (w722:T59)
      }
      frame "Chart Time Changed" {
        w791 = 2 ("Index(0)")
        n370 = call "Set pannel updating true.vi"("error in"=w802, "Index(0)"=w791) -> ("error out"=w793:errorcluster)  [unwired: 5 in]
        n371 = call "emi_Defer Panel Updates ON.vi"("error in (no error)"=w793) -> ("error out"=w795:errorcluster)  [unwired: 13 in, 1 out]
        n372 = Get Date/Time In Seconds() -> (seconds since 1Jan1904=w787:timestamp)
        n373 = control-ref of="Chart 1"() -> (w800:refnum<vi>)
        n374 = control-ref of="Chart 2"() -> (w797:refnum<vi>)
        n375 = control-ref of="Annotation Chart"() -> (w796:refnum<vi>)
        n376 = To Double Precision Float(number=w787) -> (double precision float=w785:dbl)
        n377 = case shown="\"10 minutes\"" "Chart Visible Time selector" {
          tunnel: [10.0 ("X Scale.Range:Maximum") 60.0 ("X Scale.Range:Maximum") 300.0 ("X Scale.Range:Maximum") 600.0 ("X Scale.Range:Maximum") 1800.0 ("X Scale.Range:Maximum") 3600.0 ("X Scale.Range:Maximum")] -> w786
          frame "10 Seconds" {
          }
          frame "1 minute" {
          }
          frame "5 minutes" {
          }
          frame "10 minutes" {
          }
          frame "30 minutes" {
          }
          frame "1 Hour" {
          }
        }
        n378 = Build Array(w800, w797, w796) -> (w798:refnum<vi>[])
        n379 = for {
          tunnel: w795 -> [w806]
          tunnel: w798 -> [w807] mode=indexing
          tunnel: [w809] -> w794
          tunnel: w786 -> [w808]
          tunnel: w785 -> [_]
          n380 = property class="WFChart"(reference=w807, error in=w806) -> (reference out=w812:refnum<vi>, error out=w813:errorcluster, "XScale.Maximum"=w805:dbl)
          n381 = Subtract(x=w805, y=w808) -> (x-y=w804:dbl)
          n382 = property class="WFChart"(reference=w812, error in=w813, "XScale.Minimum"=w804) -> (reference out=w810:refnum<vi>, error out=w811:errorcluster)
          n383 = Close Reference(reference=w810, error in (no error)=w811) -> (error out=w809:errorcluster)
        }
        n384 = feedback #2(0) -> (w790:i32)
        n385 = Increment(x=w790) -> (x+1=w788:i32)
        n386 = feedback-in #2(w788) -> ()
        n387 = call "emi_Defer Panel Updates OFF.vi"("error in (no error)"=w794) -> ("error out"=w792:errorcluster)  [unwired: 13 in, 1 out]
        n388 = call "Set pannel updating false.vi"("error in"=w792, "Index(0)"=w791) -> ("error out"=w801:errorcluster)  [unwired: 5 in]
      }
      frame "Graph Dialog Show" {
        w845 = Loop_ID."GUI-GrphW Mast" ("Loop ID")
        n389 = Variant To Data(error in=w842, type=0, Variant=w831) -> (data=w829:i32, error out=w826:errorcluster)
        n390 = case shown="1" w829 {
          tunnel: [w858 w863] -> w838
          tunnel: [w857 w862] -> w837
          tunnel: [w856 w861] -> w836
          tunnel: [w855 w860] -> w835
          tunnel: [w854 w859] -> w823
          frame 1 {
            n391 = control-ref of="Chart 2"() -> (w854:refnum<vi>)
            n392 = local read "Plot G2 L1"() -> (w858:T20)
            n393 = local read "Plot G2 L2"() -> (w857:T20)
            n394 = local read "Plot G2 R1"() -> (w856:T20)
            n395 = local read "Plot G2 R2"() -> (w855:T20)
          }
          frame 0, Default {
            n396 = control-ref of="Chart 1"() -> (w859:refnum<vi>)
            n397 = local read "Plot G1 L1"() -> (w863:T20)
            n398 = local read "Plot G1 L2"() -> (w862:T20)
            n399 = local read "Plot G1 R1"() -> (w861:T20)
            n400 = local read "Plot G1 R2"() -> (w860:T20)
          }
        }
        n401 = local read "Chart Visible Time selector"() -> (w832:T21)
        n402 = case shown="\"1 minute\"" w832 {
          tunnel: [10 ("Numb Sec Shown") 60 ("Numb Sec Shown") 300 ("Numb Sec Shown") 600 ("Numb Sec Shown") 1800 ("Numb Sec Shown") 3600 ("Numb Sec Shown")] -> w827
          frame "10 Seconds" {
          }
          frame "1 minute" {
          }
          frame "5 minutes" {
          }
          frame "10 minutes" {
          }
          frame "30 minutes" {
          }
          frame "1 Hour" {
          }
        }
        n403 = for {
          N: 2 -> [_]
          shift-right: [w852] -> w825
          shift-left: w826 -> [w853]
          tunnel: w823 -> [w851]
          tunnel: [w849] -> w822 mode=indexing
          i -> [w850]
          n404 = call "Graph Get Y scale Settings.vi"("error in (no error)"=w853, "Active Y Scale"=w850, "Chart Ref"=w851) -> ("error out"=w852:errorcluster, "Y scale"=w849:T50)  [unwired: 7 in]
        }
        n405 = Index Array(array=w822) -> (element #1=w821:T50, element #2=w820:T50)  [unwired: 2 in]
        n406 = Get Date/Time In Seconds() -> (seconds since 1Jan1904=w834:timestamp)
        n407 = Subtract(x=w834, y=w827) -> (x-y=w828:timestamp)
        n408 = Bundle By Name(cluster=T51 {"Start Time"=timestamp(0 s since 1904-01-01), "Numb Sec Shown"=0, "Plot  L1"={"Var Tag"=0, "Color"=0, "Line Width"=0}, "Plot  L2"={"Var Tag"=0, "Color"=0, "Line Width"=0}, "Plot  R1"={"Var Tag"=0, "Color"=0, "Line Width"=0}, "Plot  R2"={"Var Tag"=0, "Color"=0, "Line Width"=0}, "Left Y-scale"={"Maximum"=0.0, "Minimum"=0.0, "Autoscaling"=0}, "Right Y-scale"={"Maximum"=0.0, "Minimum"=0.0, "Autoscaling"=0}} ("Settigner fra MAin in"), "Start Time"=w828, "Numb Sec Shown"=w827, "Plot  L1"=w838, "Plot  L2"=w837, "Plot  R1"=w836, "Plot  R2"=w835, "Left Y-scale"=w821, "Right Y-scale"=w820) -> (w839:T51)
        n409 = call "Graph vindu settinger.vi"("Action(GET)"=enum16{"GET", "SET"}."SET", "Settigner fra MAin in"=w839, "error in (no error)"=w825) -> ("error out"=w841:errorcluster)  [unwired: 11 in, 1 out]
        n410 = call-poly "emi_SMLoop Get State.vi"("Loop ID in"=w845, "error in (no error)"=w841) -> ("Loop Running Out"=w844:bool, "error out"=w846:errorcluster)  [unwired: 7 in, 5 out]
        n411 = Not(x=w844) -> (.not. x?=w843:bool)
        n412 = call-poly "emi_SMLoop Control.vi"("Loop ID in"=w845, "Enable"=w843, "error in (no error)"=w846) -> ("error out"=w847:errorcluster)  [unwired: 11 in, 1 out]
      }
      frame "Annotation, New" {
        n413 = call "User GFV ini.vi"("Action(GET)"=enum16{"GET", "SET"}."GET", "error in (no error)"=w870) -> ("User ID out"=w874:T22, "error out"=w876:errorcluster)  [unwired: 12 in]
        n414 = Unbundle By Name(w874) -> ("User Name"=w873:string)
        n415 = Bundle By Name(cluster=T52 {"Annotation"="", "User"="", "time"=timestamp(0 s since 1904-01-01)} ("output cluster"), "User"=w873) -> (w871:T52)
        n416 = Bundle By Name(cluster=T46 {"ID"=enum."Annotation", "Details"=variant} ("element"), "Details"=w871) -> (w872:T46)
        n417 = call "Dialog Selector SIC.vi"("error in (no error)"=w876) -> ("Dialog Selector Q"=w880:refnum<queue>, "error out"=w881:errorcluster)  [unwired: 13 in]
        n418 = Enqueue Element At Opposite End(queue=w880, element=w872, error in (no error)=w881) -> (error out=w878:errorcluster)  [unwired: 1 in, 2 out]
      }
      frame "Annotation Created" {
        # "TODO Lag S&E beskjed"
        # "TODO, Legg i fil"
        # "Marks annotation in chart"
        # "TODO: Lagriong og visning av Annotasjoner..\n\nFremtidig:\nMulig linking av Anotasjoenr mot visse grafer.\nMulighet til å legge til annotajoner i Graph Viewen. Trenger da i utgangspungtet å logge båte Anotasjons tidspungtet, OG, tidspuungtet det gjelder for.\nVise Annotasjoner i detalj Graph"
        n419 = Variant To Data(error in=w894, type=T52 {"Annotation"="", "User"="", "time"=timestamp(0 s since 1904-01-01)} ("output cluster"), Variant=w893) -> (data=w887:T52, error out=w890:errorcluster)
        n420 = call "Annotation Holder.vi"("Action"=Actin_Annotatino_Holder."Add Single", "Annotation in"=w887, "error in (no error)"=w890) -> ("error out"=w889:errorcluster)  [unwired: 8 in, 4 out]
        n421 = Unbundle By Name(w887) -> ("Annotation"=w883:string, "User"=w884:string)
        n422 = call "Running Annotation Unmarked.vi"("Action(GET)"=enum16{"GET", "SET"}."SET", "Untisplayed Annotation in"=TRUE, "error in (no error)"=w889) -> ("error out"=w886:errorcluster)  [unwired: 11 in, 1 out]
        n423 = call "Send S&E Anotation message.vi"("Annotation"=w883, "error in (no error)"=w886, "User(logged on)"=w884) -> ("error out"=w885:errorcluster)  [unwired: 11 in, 1 out]
      }
      frame "PCP CMD" {
        (unwired) PCP_High_Level_Commands."HVPSU HV ON" ("PCP")
        n424 = disable-structure shown="Enabled" {
          disable-tunnel: w910 -> [w934 w935]
          disable-tunnel: [w933 w935] -> w909
          frame Disabled {
            n425 = call <vilib>:"Set Busy.vi"("error in (no error)"=w934) -> ("error out"=w933:errorcluster)  [unwired: 9 in, 1 out]
          }
          frame Enabled {
          }
        }
        n426 = Variant To Data(error in=w909, type=T54 {"PCP"=enum."HVPSU HV ON", "SP"=0.0} ("PCP beskjed"), Variant=w911) -> (data=w913:T54, error out=w907:errorcluster)
        n427 = Unbundle(w913) -> ("PCP"=w903:T40, "SP"=w912:dbl)
        n428 = call "PSU interface to use GFV.vi"() -> ("PSU type  out"=w897:T41)  [unwired: 14 in, 1 out]
        n429 = case shown="Default" w903 {
          tunnel: w907 -> [w931 w932]
          tunnel: [w930 w932] -> w906
          frame Default {
            n430 = call <vilib>:"Set Busy.vi"("error in (no error)"=w931) -> ("error out"=w930:errorcluster)  [unwired: 9 in, 1 out]
          }
          frame "Update Motor Voltage", "Update Cable Resistance" {
          }
        }
        n431 = call "Send PCP command.vi"("PSU type"=w897, "PCP"=w903, "SP"=w912, "error out 2"=w906) -> ("d(0.0)"=w901:dbl, "Final motor voltage update made"=w900:bool, "Updated motor voltage pending"=w899:bool, "error out"=w908:errorcluster)  [unwired: 8 in]
        n432 = call <vilib>:"Clear Errors.vi"("error in (no error)"=w908) -> ("error out"=w905:errorcluster)  [unwired: 6 in]
        n433 = case shown="False" w900 {
          tunnel: w898 -> [w916 w926]
          tunnel: [w915 w925] -> w902
          tunnel: w901 -> [w917 _]
          tunnel: w899 -> [w918 _]
          frame False {
            n434 = case shown="True" w918 {
              tunnel: w917 -> [_ w920]
              tunnel: w916 -> [w919 w923]
              tunnel: [w919 w922] -> w915
              frame False {
              }
              frame True {
                n435 = Bundle By Name(cluster=w923, "Do motor update"=TRUE ("Do moter update"), "Motor voltage"=w920) -> (w922:T59)
              }
            }
          }
          frame True {
            n436 = Bundle By Name(cluster=w926, "Do motor update"=FALSE ("Do moter update")) -> (w925:T59)
          }
        }
        n437 = case shown="Default" w903 {
          tunnel: w905 -> [w928 w929]
          tunnel: [w927 w929] -> w904
          frame Default {
            n438 = call <vilib>:"Unset Busy.vi"("error in (no error)"=w928) -> ("error out"=w927:errorcluster)  [unwired: 10 in]
          }
          frame "Update Motor Voltage", "Update Cable Resistance" {
          }
        }
      }
      frame "Show Welcome screen" {
        # "OBS: TODO\nNew session. All fil lagring bør avsluttes OSV."
        n439 = call "Dialog Selector SIC.vi"("error in (no error)"=w937) -> ("Dialog Selector Q"=w939:refnum<queue>, "error out"=w940:errorcluster)  [unwired: 13 in]
        n440 = Enqueue Element At Opposite End(queue=w939, element=T46 {"ID"=enum."Welcome screen", "Details"=variant}, error in (no error)=w940) -> (error out=w936:errorcluster)  [unwired: 1 in, 2 out]
      }
      frame "Dialog Tool analog" {
        n441 = call "Dialog Selector SIC.vi"("error in (no error)"=w946) -> ("Dialog Selector Q"=w944:refnum<queue>, "error out"=w945:errorcluster)  [unwired: 13 in]
        n442 = Enqueue Element At Opposite End(queue=w944, element=T46 {"ID"=enum."Variables Tool Analog", "Details"=variant}, error in (no error)=w945) -> (error out=w942:errorcluster)  [unwired: 1 in, 2 out]
      }
      frame "Update PCP resistance" {
      }
      frame "Tool CMD" {
        n443 = Variant To Data(error in=w961, type=Tool_specific_commands."controller relay 1 on" ("Tool command"), Variant=w960) -> (data=w951:T55, error out=w957:errorcluster)
        n444 = call <vilib>:"Set Busy.vi"("error in (no error)"=w957) -> ("error out"=w958:errorcluster)  [unwired: 9 in, 1 out]
        n445 = case shown="\"STROKER tool: Start Force Mon dir in\"" w951 {
          tunnel: ["Stroke setpoint" "Stroker force limit" w965] -> w954
          frame "controller relay 1 on", Default {
          }
          frame "STROKER tool: Start Force Mon dir in" {
          }
          frame "STROKER tool: Start Force Mon dir out" {
            n446 = local read "Stroker force limit"() -> (w965:dbl)
          }
        }
        n447 = call <vilib>:"Clear Errors.vi"("error in (no error)"=w958) -> ("error out"=w955:errorcluster)  [unwired: 6 in]
        n448 = Merge Errors(w957, w955) -> (w956:errorcluster)
        n449 = call "Send commands to tool.vi"("Tool command"=w951, "Input Data"=w954, "error in"=w956) -> ("OK"=w950:bool, "error out"=w953:errorcluster)  [unwired: 11 in]
        n450 = case shown="True" w950 {
          tunnel: w953 -> [w966 w969]
          tunnel: [w966 w968] -> w952
          tunnel: w951 -> [_ w970]
          frame False {
            n451 = One Button Dialog(message="Command not performed correctly") -> ()  [unwired: 1 in, 1 out]
          }
          frame True {
            n452 = case shown="\"Controller relay 1 & 2 on\", \"Controller relay 1 & 2 off\"" w970 {
              tunnel: w969 -> [w972 w975]
              tunnel: [w974 w975] -> w968
              frame "Controller relay 1 & 2 on", "Controller relay 1 & 2 off" {
                w971 = TRUE ("Relay 1 Initialized")
                # "Both relays initialized"
                n453 = call "Tool Relay State Initialized.vi"("Action(GET)"=enum16{"GET", "SET"}."SET", "Relay 1 Initialized"=w971, "Relay 2 Initialized"=w971, "error in (no error)"=w972) -> ("error out"=w974:errorcluster)  [unwired: 9 in, 2 out]
              }
              frame "Solonoid 1 (master) on", Default {
              }
            }
          }
        }
        n454 = call <vilib>:"Unset Busy.vi"("error in (no error)"=w952) -> ()  [unwired: 10 in, 1 out]
      }
      frame "Chart single autoscale" {
        w984 = u8 1 ("Y Scale.Scale Fit")
        n455 = Variant To Data(error in=w990, type=0, Variant=w989) -> (data=w981:i32, error out=w983:errorcluster)
        n456 = control-ref of="Chart 1"() -> (w988:refnum<vi>)
        n457 = control-ref of="Chart 2"() -> (w987:refnum<vi>)
        n458 = Build Array(w988, w987) -> (w977:refnum<vi>[])
        n459 = Index Array(array=w977, index=w981) -> (element=w980:refnum<vi>)
        n460 = property class="WFChart (strict)"(reference=w980, error in=w983, "ActYScl"=0 ("Active Y Scale"), "YScale.ScaleFit"=w984) -> (reference out=w978:refnum<vi>, error out=w982:errorcluster)
        n461 = property class="WFChart (strict)"(reference=w978, error in=w982, "ActYScl"=1 ("Active Y Scale"), "YScale.ScaleFit"=w984) -> (error out=w979:errorcluster)  [unwired: 1 out]
        n462 = Close Reference(reference=w977, error in (no error)=w979) -> (error out=w976:errorcluster)
      }
      frame "Tool connenction state" {
        # "1.0.12. \nThiw was false. No Idee why."
        n463 = Variant To Data(error in=w999, type=FALSE, Variant=w998) -> (error out=w996:errorcluster)  [unwired: 1 out]
        n464 = call-poly "emi_SMLoop Control.vi"("Loop ID in"=Loop_ID."Main display enable view" ("Loop ID"), "Enable"=TRUE, "error in (no error)"=w996) -> ("error out"=w994:errorcluster)  [unwired: 11 in, 1 out]
      }
      frame "Show detailed view" {
        n465 = call-poly "emi_SMLoop Control.vi"("Loop ID in"=Loop_ID."Detail View L1" ("Loop ID"), "Enable"=TRUE, "error in (no error)"=w1004) -> ("error out"=w1003:errorcluster)  [unwired: 11 in, 1 out]
      }
      frame "Sequences updated" {
        n466 = call "Sekvenser GFV.vi"("error in (no error)"=w1011) -> ("Sequences out"=w1009:T81[], "error out"=w1010:errorcluster)  [unwired: 13 in]
        n467 = for {
          tunnel: w1009 -> [w1017] mode=indexing
          tunnel: [w1016] -> w1008 mode=indexing
          n468 = Unbundle By Name(w1017) -> ("Sequence Name"=w1016:string)
        }
        n469 = property on="Sequence to run" class="Ring (strict)"(error in=w1010, "Strings []"=w1008) -> (error out=w1006:errorcluster)  [unwired: 1 in, 1 out]
        n470 = flat-sequence {
          tunnel: [w1015] -> w1007
          tunnel: w1006 -> [w1015]
          frame #0 {
            w1013 = "" ("Sequence progress")
            n471 = local write "Time spent on sequence step"(w1013) -> ()
            n472 = local write "Next step"(w1013) -> ()
            n473 = local write "Current step"(w1013) -> ()
            n474 = local write "Sequence progress"(w1013) -> ()
            n475 = local write "Sequence to run"(0) -> ()
          }
        }
      }
      frame "Show stroker wizard" {
        n476 = call-poly "emi_SMLoop Control.vi"("Loop ID in"=Loop_ID."Stroker Wizard L1" ("Loop ID"), "Enable"=TRUE, "error in (no error)"=w1021) -> ("error out"=w1020:errorcluster)  [unwired: 11 in, 1 out]
      }
      frame "Change tool" {
        # "This state is called when the active tool is changed.\n1. Change COM port of LEIN arbeiter (will restart the process)\n2. Change visible TABs"
        n477 = Variant To Data(error in=w1031, type=List_of_tools."Stroker" ("Tool in"), Variant=w1026) -> (data=w1029:T56, error out=w1028:errorcluster)
        n478 = call "Selected Tool holder.vi"("Action(GET)"=enum16{"GET", "SET"}."SET", "Tool in"=w1029, "error in (no error)"=w1028) -> ("Tool out"=w1027:T56, "error out"=w1023:errorcluster)  [unwired: 11 in]
        n479 = disable-structure shown="Disabled" {
          disable-tunnel: [w1037 w1046] -> w1025
          disable-tunnel: w1023 -> [w1036 w1046]
          frame Disabled {
            w1041 = u32 700  # Reply timeout
            # "NB!! I imagine this is no longer necessary"
            n480 = call "Options GFV.vi"("error in (no error)"=w1036, "Action(Get Settings)"=Action_GFV_Settings."Get Settings") -> ("Options"=w1040:T60, "error out"=w1038:errorcluster)  [unwired: 15 in, 1 out]
            n481 = Unbundle By Name(w1040) -> ("P 1 (App).Tractor/Stroker Interface"=w1039:string)
            n482 = Unbundle By Name(w1040) -> ("P 7 (Expert).Modem baud"=w1042:u16, "P 7 (Expert).Modem sim"=w1045:T73)
            n483 = call "LEIN m serial Interface settings.vi"("baud rate"=w1042, "Action(GET)"=enum16{"GET", "SET"}."SET", "Reply timeout"=w1041, "LEIN m serial VISA  name  in"=w1039, "Modem sim in"=w1045, "error in (no error)"=w1038) -> ("error out"=w1037:errorcluster)  [unwired: 4 in, 5 out]
          }
          frame Enabled {
          }
        }
        n484 = To Unsigned Word Integer(number=w1027) -> (unsigned 16bit integer=w1033:u16)
        n485 = local write "Type tab 1"(w1033) -> ()
        n486 = local write "Type tab 2"(w1033) -> ()
        n487 = local write "Type tab 3"(w1033) -> ()
        n488 = call "emi_Wait MS with err.vi"("milliseconds to wait(0)"=u32 1000, "error in (no error)"=w1025) -> ("error out"=w1024:errorcluster)  [unwired: 13 in]
      }
      frame "Reset Telemetry" {
        w1050 = 0.0
        w1047 = FALSE ("Blinking")
        w1053 = User_Event_List."Reset Telemetry" ("User Events")
        # "Stop blinking of control\nand reset Start Telemetry\nCommand button"
        n489 = control-ref of="Start Telemetry"() -> (w1051:refnum<vi>)
        n490 = property on="Property Node" class="Bool (strict)"(reference=w1051, error in=w1052, "Blinking"=w1047) -> (error out=w1048:errorcluster)  [unwired: 1 out]
        n491 = local write "Start Telemetry"(w1047) -> ()
        n492 = local write "Tool voltage setpoint(V)"(w1050) -> ()
        n493 = call "PCP Voltage Setpoint.vi"("Action(GET)"=enum16{"GET", "SET"}."SET", "PCP HV setpoint"=w1050, "error in (no error)"=w1048) -> ("error out"=w1059:errorcluster)  [unwired: 11 in, 1 out]
        n494 = Format Into String(format string="%s (%f)", error in=w1059, w1053, w1050) -> (resulting string=w1056:string, error out=w1055:errorcluster)  [unwired: 1 in]
        n495 = call "Send S&E EVENT message.vi"("Event Source(user)"=S&E_Event_source."User", "Event Description"=w1056, "error in (no error)"=w1055, "Loc Sub ID/Event ID(No ID)"=w1053) -> ("error out"=w1049:errorcluster)  [unwired: 10 in, 1 out]
      }
      frame "Stop Logging" {
        # "Stop logging loop"
        n496 = call-poly "emi_SMLoop Control.vi"("Loop ID in"=Loop_ID."Var Handling-File storage" ("Loop ID"), "Enable"=FALSE, "error in (no error)"=w1062) -> ("error out"=w1061:errorcluster)  [unwired: 11 in, 1 out]
      }
      frame "Start New Loggfile" {
        w1066 = Loop_ID."Var Handling-File storage" ("Loop ID")
        # "Check if loop has stopped"
        n497 = call "emi_Wait MS with err.vi"("milliseconds to wait(0)"=u32 50, "error in (no error)"=w1071) -> ("error out"=w1070:errorcluster)  [unwired: 13 in]
        n498 = call-poly "emi_SMLoop Get State.vi"("Loop ID in"=w1066, "error in (no error)"=w1070) -> ("Loop Running Out"=w1069:bool, "error out"=w1068:errorcluster)  [unwired: 7 in, 5 out]
        n499 = case shown="False" w1069 {
          tunnel: w1068 -> [w1076 w1079]
          tunnel: [w1075 w1078] -> w1067
          tunnel: w1066 -> [w1074 _]
          frame False {
            # "Logging loop has stopped - Start loop"
            n500 = call-poly "emi_SMLoop Control.vi"("Loop ID in"=w1074, "Enable"=TRUE, "error in (no error)"=w1076) -> ("error out"=w1075:errorcluster)  [unwired: 11 in, 1 out]
          }
          frame True {
            # "Logging loop has not yet stopped\ntry again"
            n501 = call "QSM enque.vi"("State"=QSM_State_List."Start New Loggfile", "error in"=w1079) -> ("error out"=w1078:errorcluster)  [unwired: 13 in]
          }
        }
      }
      frame "Update control units" {
        # "Initialize user inputs with unit captions and input range"
        n502 = call "Selected Tool holder.vi"("error in (no error)"=w1083) -> ("Tool out"=w1081:T56, "error out"=w1082:errorcluster)  [unwired: 13 in]
        n503 = case shown="\"Stroker\"" w1081 {
          tunnel: [w1086 w1090] -> w1084
          tunnel: w1082 -> [w1086 w1089]
          frame "Tractor", Default {
            # "2013-09-13 OOS:\nCurrently Tractor and Driller does not have\nany inputs with configurable units"
          }
          frame "Stroker" {
            w1087 = Variable_List_Tool_Analog."Stroke Extension" ("Variable ID")
            w1088 = Variable_List_Tool_Analog."Stroke Force" ("Variable ID")
            w1096 = 0.5  # length of extended stroker [m]
            n504 = call "GS Var TOOL Ana Fixed Settings.vi"("error in (no error)"=w1089) -> ("Tool Analog var Fixed out"=w1109:T85[], "error out"=w1104:errorcluster)  [unwired: 12 in, 1 out]
            n505 = Index Array(array=w1109, index #1=w1088, index #2=w1087) -> (element #1=w1107:T85, element #2=w1101:T85)
            n506 = call "GS Var Tool Common Ana User Settings.vi"("error in (no error)"=w1104) -> ("Tool Analog var User settigns out"=w1110:T91[], "error out"=w1097:errorcluster)  [unwired: 12 in, 1 out]
            n507 = Index Array(array=w1110, index #1=w1088, index #2=w1087) -> (element #1=w1108:T91, element #2=w1102:T91)
            n508 = Unbundle By Name(w1107) -> ("Quantity"=w1106:T86)
            n509 = Unbundle By Name(w1108) -> ("Unit"=w1105:u16)
            n510 = Unbundle By Name(w1101) -> ("Quantity"=w1100:T86)
            n511 = Unbundle By Name(w1102) -> ("Unit"=w1099:u16)
            n512 = call "Get Unit Scaling.vi"("Unit Index"=w1099, "Quantity"=w1100) -> ("Gain"=w1095:dbl, "Unit"=w1098:string)  [unwired: 7 in, 1 out]
            n513 = call "Get Unit Scaling.vi"("Unit Index"=w1105, "Quantity"=w1106) -> ("Unit"=w1103:string)  [unwired: 7 in, 2 out]
            n514 = property on="Stroker force limit" class="DigNum (strict)"(error in=w1097, "Caption.Text"=w1103) -> (error out=w1111:errorcluster)  [unwired: 1 in, 1 out]
            n515 = Multiply(x=w1095, y=w1096) -> (x*y=w1094:dbl)
            n516 = property on="Stroke setpoint" class="Slide (strict)"(error in=w1111, "Caption.Text"=w1098) -> (error out=w1093:errorcluster)  [unwired: 1 in, 1 out]
            n517 = property on="Stroker" class="Slide (strict)"(error in=w1093, "Scale.Maximum"=w1094) -> (error out=w1092:errorcluster)  [unwired: 1 in, 1 out]
            n518 = property on="Stroker  2" class="Slide (strict)"(error in=w1092, "Scale.Maximum"=w1094) -> (error out=w1091:errorcluster)  [unwired: 1 in, 1 out]
            n519 = property on="Stroke setpoint" class="Slide (strict)"(error in=w1091, "Scale.Maximum"=w1094) -> (error out=w1090:errorcluster)  [unwired: 1 in, 1 out]
          }
        }
      }
      frame "Log Init" {
        n520 = disable-structure shown="Enabled" {
          disable-tunnel: w1114 -> [w1121 w1194]
          disable-tunnel: [w1118 w1209] -> w1113
          frame Disabled {
            n521 = call "GFV project info.vi"("error in (no error)"=w1121) -> ("Project info out"=w1117:T96, "error out"=w1119:errorcluster)  [unwired: 13 in]
            n522 = Unbundle By Name(w1117) -> ("data.Run Information.Active Run"=w1120:bool)
            n523 = case shown="True" w1120 {
              tunnel: w1119 -> [w1124 w1139]
              tunnel: [w1123 w1138] -> w1118
              tunnel: w1117 -> [w1122 w1137]
              tunnel: [FALSE ("String Check Rec") w1136] -> w1116
              tunnel: [FALSE ("String Check Rec") w1135] -> w1115
              frame False {
                w1127 = FALSE ("Run Information.Active Run")
                n524 = Unbundle By Name(w1122) -> ("Project path"=w1129:path, "Comment"=w1126:string, "data"=w1128:T97)
                n525 = Bundle By Name(cluster=w1128, "Run Information.Active Run"=w1127, "Run Information.String Check Rec"=w1127) -> (w1125:T97)
                n526 = call "Create or update project ini file.vi"("Project file path"=w1129, "Comment"=w1126, "Project information"=w1125, "error in (no error)"=w1124) -> ("error out"=w1132:errorcluster)  [unwired: 11 in]
                n527 = Bundle By Name(cluster=w1122, "data"=w1125) -> (w1131:T96)
                n528 = call "GFV project info.vi"("Action(GET)"=enum16{"GET", "SET"}."SET", "Project info in"=w1131, "error in (no error)"=w1132) -> ("error out"=w1123:errorcluster)  [unwired: 11 in, 1 out]
              }
              frame True {
                n529 = Two Button Dialog(message="A run was active the last time Beagle shut down. Do you want to continue this run?", 1:"Stop run" ("F button name (\"Cancel\")"), 2:"Continue run" ("T button name (\"OK\")")) -> (T button?=w1140:bool)
                n530 = case shown="True" w1140 {
                  tunnel: w1139 -> [w1146 w1157]
                  tunnel: [w1147 w1161] -> w1138
                  tunnel: w1137 -> [w1153 w1158]
                  tunnel: [FALSE ("String Check Rec") w1160] -> w1136
                  tunnel: [FALSE ("String Check Rec") w1159] -> w1135
                  frame False {
                    w1150 = FALSE ("Run Information.Active Run")
                    n531 = Unbundle By Name(w1153) -> ("Project path"=w1152:path, "Comment"=w1149:string, "data"=w1151:T97)
                    n532 = Bundle By Name(cluster=w1151, "Run Information.Active Run"=w1150, "Run Information.String Check Rec"=w1150) -> (w1148:T97)
                    n533 = call "Create or update project ini file.vi"("Project file path"=w1152, "Comment"=w1149, "Project information"=w1148, "error in (no error)"=w1146) -> ("error out"=w1156:errorcluster)  [unwired: 11 in]
                    n534 = Bundle By Name(cluster=w1153, "data"=w1148) -> (w1155:T96)
                    n535 = call "GFV project info.vi"("Action(GET)"=enum16{"GET", "SET"}."SET", "Project info in"=w1155, "error in (no error)"=w1156) -> ("error out"=w1147:errorcluster)  [unwired: 11 in, 1 out]
                  }
                  frame True {
                    # "Continue active Run\nNew data will be appended to the existing logfile\nThe Analog Handler is initialized with data from file"
                    n536 = call "Initialize Graph from logfile.vi"("error in"=w1157) -> ("error out"=w1164:errorcluster, "Data out"=w1163:dbl[][], "Corrupt"=w1162:bool)  [unwired: 8 in]
                    n537 = case shown="False" w1162 {
                      tunnel: w1164 -> [w1172 w1180]
                      tunnel: [w1167 w1179] -> w1161
                      tunnel: w1163 -> [w1170 _]
                      tunnel: [FALSE ("String Check Rec") FALSE ("String Check Rec")] -> w1160
                      tunnel: [TRUE ("String Check Rec") FALSE ("String Check Rec")] -> w1159
                      tunnel: w1158 -> [_ w1178]
                      frame False {
                        n538 = for {
                          shift-right: [w1176] -> w1168
                          shift-left: w1172 -> [w1177]
                          tunnel: Action_Analog_Handler."Set initial waveform" ("Action") -> [w1175]
                          tunnel: w1170 -> [w1174] mode=indexing
                          i -> [w1173]
                          n539 = call "analog Handler.vi"("Variable Index"=w1173, "Action"=w1175, "error in (no error)"=w1177, "Initial Data"=w1174) -> ("error out"=w1176:errorcluster)  [unwired: 6 in, 5 out]
                        }
                        n540 = call "QSM enque.vi"("State"=QSM_State_List."Start New Loggfile", "error in"=w1168) -> ("error out"=w1167:errorcluster)  [unwired: 13 in]
                      }
                      frame True {
                        w1183 = FALSE ("Run Information.Active Run")
                        n541 = Unbundle By Name(w1178) -> ("Project path"=w1185:path, "Comment"=w1182:string, "data"=w1184:T97)
                        n542 = Bundle By Name(cluster=w1184, "Run Information.Active Run"=w1183, "Run Information.String Check Rec"=w1183) -> (w1181:T97)
                        n543 = One Button Dialog(message="An error occurred when loading the logfile from the last active run.\nA new run has to be started manually!") -> ()  [unwired: 1 in, 1 out]
                        n544 = call "Create or update project ini file.vi"("Project file path"=w1185, "Comment"=w1182, "Project information"=w1181, "error in (no error)"=w1180) -> ("error out"=w1188:errorcluster)  [unwired: 11 in]
                        n545 = Bundle By Name(cluster=w1178, "data"=w1181) -> (w1187:T96)
                        n546 = call "GFV project info.vi"("Action(GET)"=enum16{"GET", "SET"}."SET", "Project info in"=w1187, "error in (no error)"=w1188) -> ("error out"=w1179:errorcluster)  [unwired: 11 in, 1 out]
                      }
                    }
                  }
                }
              }
            }
            n547 = local write "String Check Rec"(w1116) -> ()
            n548 = local write "Start Run"(w1115) -> ()
          }
          frame Enabled {
            # "Reset Active Run cmd button"
            # "Write Project info FGV"
            # "v1.13.0 Logging functionality introduced in v1.11.0 has been disabled.\nThe command buttons for starting and stopping logging has been made invisible"
            n549 = call "GFV project info.vi"("error in (no error)"=w1194) -> ("Project info out"=w1200:T96, "error out"=w1206:errorcluster)  [unwired: 13 in]
            n550 = Get Date/Time In Seconds() -> (seconds since 1Jan1904=w1204:timestamp)
            n551 = Unbundle By Name(w1200) -> ("Project path"=w1195:path, "Comment"=w1196:string, "data"=w1197:T97)
            n552 = Format Into String(format string="%<%Y%m%d %H%M%S>T", error in=w1206, w1204) -> (resulting string=w1208:string, error out=w1207:errorcluster)  [unwired: 1 in]
            n553 = Bundle By Name(cluster=w1197, "Run Information.Time of File Start"=w1208, "Run Information.String Check Rec"=TRUE, "Run Information.Active Run"=FALSE) -> (w1201:T97)
            n554 = call "Create or update project ini file.vi"("Project file path"=w1195, "Comment"=w1196, "Project information"=w1201, "error in (no error)"=w1207) -> ("error out"=w1199:errorcluster)  [unwired: 11 in]
            n555 = Bundle By Name(cluster=w1200, "data"=w1201) -> (w1202:T96)
            n556 = call "GFV project info.vi"("Action(GET)"=enum16{"GET", "SET"}."SET", "Project info in"=w1202, "error in (no error)"=w1199) -> ("error out"=w1193:errorcluster)  [unwired: 11 in, 1 out]
            n557 = call "QSM enque.vi"("State"=QSM_State_List."Start New Loggfile", "error in"=w1193) -> ("error out"=w1209:errorcluster)  [unwired: 13 in]
          }
        }
      }
      frame "Copy INI files" {
        # "This Case copies all settings that were used during the job to the project folder\nThis makes it possible to view what settings were used during the project"
        n558 = call "GFV project info.vi"("error in (no error)"=w1213) -> ("Project info out"=w1218:T96, "error out"=w1214:errorcluster)  [unwired: 13 in]
        n559 = Unbundle By Name(w1218) -> ("Project path"=w1217:path)
        n560 = Build Array("Config.ini", "Variables.ini" ("name or relative path"), "Tool Variables.ini" ("name or relative path"), "Modem Status Variables.ini" ("element")) -> (w1219:string[])
        n561 = for {
          tunnel: w1219 -> [w1227] mode=indexing
          tunnel: w1217 -> [w1228]
          tunnel: [w1225] -> w1216 mode=indexing
          tunnel: w1214 -> [w1224]
          n562 = call "emi_Default Ini File Name.vi"("Name"=w1227, "error in (no error)"=w1224) -> ("Path"=w1231:path, "error out"=w1229:errorcluster)  [unwired: 12 in]
          n563 = Build Path(base path=w1228, name or relative path=w1227) -> (appended path=w1226:path)
          n564 = Copy(8:w1229, 9:TRUE ("overwrite (F)"), 10:w1226, 11:w1231) -> (0:w1225:errorcluster)  [unwired: 1 in, 2 out]
        }
        n565 = Merge Errors(w1216) -> (w1215:errorcluster)
        n566 = call <vilib>:"Clear Errors.vi"("error in (no error)"=w1215) -> ("error out"=w1212:errorcluster)  [unwired: 6 in]
      }
    }
    n567 = call "QSM End of Loop.vi"("error in"=w64, "QSM state"=w62) -> ("error out"=w63:errorcluster)  [unwired: 13 in]
  }
  n568 = while "Sequence" {
    shift-right: [w1243] -> _
    shift-left: _ -> [w1239]
    shift-right: [w1241] -> _
    shift-left: w2 -> [w1237]
    tunnel: [w1240] -> _
    shift-right: [w1238] -> _
    shift-left: _ -> [w1233]
    tunnel: Loop_ID."Sequence runner" ("Loop ID") -> [w1234]
    i -> [w1240]
    stop <- w1242 stop-if-true
    n569 = call "emi_SMLoop Start.vi"("Loop ID"=w1234, "error in (no error)"=w1237, "Force Stop(F)"=w1233) -> ("Loop command"=w1235:T102, "error out"=w1236:errorcluster, "Loop ID out"=w1232:i32)  [unwired: 10 in]
    n570 = case shown="\"Normal Operation\"" w1235 {
      tunnel: [w1253 w1254 w1281 w1325 w1429 w1431 w1432 w1435] -> w1243
      tunnel: [_ _ _ _ _ _ _ TRUE] -> w1242
      tunnel: w1236 -> [w1245 w1256 w1275 w1324 w1428 w1430 w1433 w1436]
      tunnel: [w1244 w1255 w1277 w1310 w1419 w1430 w1433 w1436] -> w1241
      tunnel: w1239 -> [_ w1254 w1283 w1326 w1429 w1431 w1432 w1435]
      tunnel: [w1251 _ _ w1302 _ _ _ _] -> w1238
      tunnel: w1232 -> [_ _ _ _ w1425 _ _ _]
      frame "Init" {
        w1247 = T81 {"Sequence Name"="", "User input 1"={"Input name"="", "Minimum value "=0.0, "Maximum value"=0.0, "Default value"=0.0, "User inp enabled"=FALSE}, "Steps"=[]}  # Sequences
        w1248 = timestamp(0 s since 1904-01-01)  # Action time
        w1249 = 0  # Step index
        w1250 = TRUE  # Perform action
        w1251 = FALSE  # Force end
        w1252 = TRUE  # Op button disabled
        # "First case that is executed, executes regardless of loop beeing enabled.\nOnly executes once. Init loop data and other variables."
        n571 = property on="Start sequence" class="Bool (strict)"(error in=w1245, "DisabledEnum"=T45."Enabled" ("Disabled")) -> (error out=w1244:errorcluster)  [unwired: 1 in, 1 out]
        n572 = Bundle("Op button disabled"=w1252, "Perform action"=w1250, "Step index"=w1249, "Action time"=w1248, "Sequences"=w1247) -> (w1253:T103)  [unwired: 1 in]
      }
      frame "Standby", Default {
        # "Case that is executed when the loop is not enabled. Should not be edited."
        n573 = call "emi_Wait MS with err.vi"("milliseconds to wait(0)"=u32 50, "error in (no error)"=w1256) -> ("error out"=w1255:errorcluster)  [unwired: 13 in]
      }
      frame "Start" {
        w1269 = "" ("Sequence progress")
        w1278 = 0  # Step index
        w1279 = TRUE  # Perform action
        w1280 = TRUE  # Op button disabled
        # "Start or restart the loop. Should perform any init code. \nOpen channel and so on. Will perform each time the system is restarted."
        n574 = local read "Sequence to run"() -> (w1273:u16)
        n575 = call "Sekvenser GFV.vi"("error in (no error)"=w1275) -> ("Sequences out"=w1272:T81[], "error out"=w1274:errorcluster)  [unwired: 13 in]
        n576 = Index Array(array=w1272, index=w1273) -> (element=w1267:T81)
        n577 = property on="Approve step" class="Bool (strict)"(error in=w1274, "DisabledEnum"=T45."Disabled and Grayed Out" ("Disabled")) -> (error out=w1271:errorcluster)  [unwired: 1 in, 1 out]
        n578 = property on="Stopp sequence" class="Bool (strict)"(error in=w1271, "DisabledEnum"=T45."Enabled" ("Disabled")) -> (error out=w1258:errorcluster)  [unwired: 1 in, 1 out]
        n579 = Unbundle By Name(w1267) -> ("User input 1.User inp enabled"=w1265:bool, "User input 1.Input name"=w1264:string, "User input 1.Maximum value"=w1263:dbl, "User input 1.Minimum value"=w1262:dbl, "User input 1.Default value"=w1261:dbl)
        n580 = property on="Start sequence" class="Bool (strict)"(error in=w1258, "DisabledEnum"=T45."Disabled and Grayed Out" ("Disabled")) -> (error out=w1259:errorcluster)  [unwired: 1 in, 1 out]
        n581 = case shown="True" w1265 {
          tunnel: w1259 -> [w1291 w1294]
          tunnel: [w1286 w1293] -> w1266
          tunnel: w1264 -> [w1289 _]
          tunnel: w1263 -> [w1285 _]
          tunnel: w1262 -> [w1284 _]
          tunnel: w1261 -> [w1288 _]
          frame True {
            n582 = property on="Sequence user input" class="DigNum (strict)"(error in=w1291, "Visible"=TRUE) -> (error out=w1287:errorcluster)  [unwired: 1 in, 1 out]
            n583 = local write "Sequence user input name"(w1289) -> ()
            n584 = local write "Sequence user input"(w1288) -> ()
            n585 = property on="Sequence user input" class="DigNum (strict)"(error in=w1287, "Maximum"=w1285, "Minimum"=w1284) -> (error out=w1286:errorcluster)  [unwired: 1 in, 1 out]
          }
          frame False {
            n586 = property on="Sequence user input" class="DigNum (strict)"(error in=w1294, "Visible"=FALSE) -> (error out=w1293:errorcluster)  [unwired: 1 in, 1 out]
          }
        }
        n587 = call "emi_Get DateTime In Seconds err & offs.vi"("error in (no error)"=w1266) -> ("Time"=w1276:timestamp, "error out"=w1277:errorcluster)  [unwired: 13 in]
        n588 = local write "Current step"(w1269) -> ()
        n589 = local write "Sequence progress"(w1269) -> ()
        n590 = local write "Time spent on sequence step"(w1269) -> ()
        n591 = local write "Next step"(w1269) -> ()
        n592 = local write "Approve step"(FALSE ("Approve step")) -> ()
        n593 = Bundle By Name(cluster=w1283, "Op button disabled"=w1280, "Perform action"=w1279, "Step index"=w1278, "Action time"=w1276, "Sequences"=w1267) -> (w1281:T103)
      }
      frame "Normal Operation" {
        # "Bloddy hell:"
        # "Normal Throughput"
        # "All normal tasks belong here. This will be repeated, until error, disable, restart or\nforsed to restart. OBS, reduce overhead with internal loop(will execute unevenly)."
        n594 = local read "Approve step"() -> (w1315:bool)
        n595 = Unbundle By Name(w1326) -> ("Op button disabled"=w1314:bool, "Perform action"=w1320:bool, "Step index"=w1316:i32, "Sequences"=w1322:T81, "Action time"=w1321:timestamp)
        n596 = Unbundle By Name(w1322) -> ("Steps"=w1312:T25[])
        n597 = Array Size(array=w1312) -> (size(s)=w1311:i32)
        n598 = Index Array(array=w1312, index #1=w1316) -> (element #1=w1317:T25, element #2=w1301:T25)  [unwired: 1 in]
        n599 = case shown="True" w1320 {
          selector: w1320 -> [_ w1402]
          tunnel: w1316 -> [w1342 w1379]
          tunnel: w1321 -> [w1344 _]
          tunnel: w1317 -> [w1345 w1395]
          tunnel: w1324 -> [w1334 w1372]
          tunnel: [w1344 w1403] -> w1308
          tunnel: [w1341 w1370] -> w1323
          tunnel: [w1343 w1401] -> w1319
          tunnel: [w1337 w1400] -> w1318
          tunnel: [w1336 w1397] -> w1302
          tunnel: w1315 -> [w1335 _]
          tunnel: w1314 -> [_ w1396]
          tunnel: [w1338 w1396] -> w1313
          tunnel: w1311 -> [w1332 w1393]
          tunnel: w1301 -> [_ w1382]
          tunnel: [_ w1365] -> w1299
          tunnel: [_ w1369] -> w1300
          tunnel: "Sequence user input" -> [w1330 w1368]
          tunnel: [_ w1367] -> w1297
          tunnel: [_ w1366] -> w1296
          tunnel: [_ w1365] -> w1295
          frame False {
            n600 = Increment(x=w1342) -> (x+1=w1331:i32)
            n601 = case shown="True" w1335 {
              tunnel: w1334 -> [w1346 w1353]
              tunnel: [w1346 w1352] -> w1333
              tunnel: w1331 -> [_ w1348]
              frame False {
              }
              frame True {
                w1354 = User_Event_List."Sequence step approved" ("User Events")
                n602 = Number To Decimal String(number=w1348) -> (decimal integer string=w1347:string)  [unwired: 1 in]
                n603 = Format Into String(error in=w1353, w1354) -> (resulting string=w1350:string, error out=w1355:errorcluster)  [unwired: 2 in]
                n604 = Concatenate Strings(w1350, "  Step:" ("string"), w1347) -> (w1351:string)
                n605 = call "Send S&E EVENT message.vi"("Event Source(user)"=S&E_Event_source."User", "Event Description"=w1351, "error in (no error)"=w1355, "Loc Sub ID/Event ID(No ID)"=w1354) -> ("error out"=w1352:errorcluster)  [unwired: 10 in, 1 out]
              }
            }
            n606 = call "Check if ready for next step.vi"("data step cluster"=w1345, "Time since action"=w1344, "Operator input"=w1335, "error in (no error)"=w1333, "User input 1"=w1330) -> ("Next step"=w1343:bool, "Show operator button"=w1338:bool, "error out"=w1340:errorcluster)  [unwired: 8 in]
            n607 = Not Equal?(x=w1338, y=w1335) -> (x != y?=w1339:bool)
            n608 = case shown="True" w1339 {
              tunnel: [w1357 w1364] -> w1341
              tunnel: w1340 -> [w1357 w1363]
              tunnel: w1338 -> [_ w1359]
              frame False {
              }
              frame True {
                n609 = local write "Approve step"(FALSE ("Approve step")) -> ()
                n610 = Select(t=T45."Enabled", s=w1359, f=T45."Disabled and Grayed Out" ("Disabled")) -> (s? t:f=w1361:T45)
                n611 = property on="Approve step" class="Bool (strict)"(error in=w1363, "DisabledEnum"=w1361) -> (error out=w1364:errorcluster)  [unwired: 1 in, 1 out]
              }
            }
            n612 = Select(t=w1331, s=w1343, f=w1342) -> (s? t:f=w1337:i32)
            n613 = Equal?(x=w1337, y=w1332) -> (x = y?=w1336:bool)
          }
          frame True {
            w1388 = User_Event_List."Sequence action" ("User Events")
            # "Perform action"
            n614 = call <vilib>:"Set Busy.vi"("error in (no error)"=w1372) -> ("error out"=w1374:errorcluster)  [unwired: 9 in, 1 out]
            n615 = call "criteria string.vi"("Sequence step config"=w1395, "User input"=w1368) -> ("Full criteria string"=w1394:string)  [unwired: 12 in, 1 out]
            n616 = call <vilib>:"Clear Errors.vi"("error in (no error)"=w1374) -> ("error out"=w1373:errorcluster)  [unwired: 6 in]
            n617 = Number To Decimal String(number=w1379) -> (decimal integer string=w1384:string)  [unwired: 1 in]
            n618 = Merge Errors(w1372, w1373) -> (w1371:errorcluster)
            n619 = Increment(x=w1379) -> (x+1=w1381:i32)
            n620 = Increment(x=w1381) -> (x+1=w1380:i32)
            n621 = Format Into String(format string="Step %d of %d", w1381, w1393) -> (resulting string=w1391:string)  [unwired: 2 in, 1 out]
            n622 = Format Into String(error in=w1371, w1388) -> (resulting string=w1386:string, error out=w1389:errorcluster)  [unwired: 2 in]
            n623 = Equal?(x=w1380, y=w1379) -> (x = y?=w1378:bool)
            n624 = local write "Sequence progress"(w1391) -> ()
            n625 = local write "Current step"(w1394) -> ()
            n626 = Concatenate Strings(w1386, "  Step:" ("string"), w1384) -> (w1387:string)
            n627 = call "criteria string.vi"("Sequence step config"=w1382, "Finnished(F)"=w1378, "User input"=w1368) -> ("Actino string"=w1377:string)  [unwired: 11 in, 1 out]
            n628 = call "Send S&E EVENT message.vi"("Event Source(user)"=S&E_Event_source."User", "Event Description"=w1387, "error in (no error)"=w1389, "Loc Sub ID/Event ID(No ID)"=w1388) -> ("error out"=w1383:errorcluster)  [unwired: 10 in, 1 out]
            n629 = call "Perform actrion and wait for responce.vi"("data step cluster"=w1395, "error in (no error)"=w1383) -> ("Rdesistance go to"=w1367:bool, "Voltage go to"=w1366:bool, "Continue"=w1398:bool, "Retry"=w1399:bool, "Stroke  go to"=w1369:bool, "Action value tool"=w1365:dbl, "error out"=w1404:errorcluster)  [unwired: 7 in]
            n630 = call "emi_Get DateTime In Seconds err & offs.vi"("error in (no error)"=w1404) -> ("Time"=w1403:timestamp, "error out"=w1370:errorcluster)  [unwired: 13 in]
            n631 = case shown="True" w1398 {
              tunnel: w1402 -> [_ _]
              tunnel: w1379 -> [w1408 w1410]
              tunnel: w1399 -> [w1406 _]
              tunnel: [TRUE FALSE] -> w1401
              tunnel: [w1408 w1410] -> w1400
              tunnel: [w1405 FALSE] -> w1397
              frame False {
                n632 = Not(x=w1406) -> (.not. x?=w1405:bool)
              }
              frame True {
              }
            }
            n633 = Concatenate Strings("Next action: " ("string"), w1377) -> (→"Next step":string)
            n634 = call <vilib>:"Unset Busy.vi"("error in (no error)"=w1370) -> ()  [unwired: 10 in, 1 out]
          }
        }
        n635 = case shown="True" w1296 {
          tunnel: w1295 -> [_ w1328]
          frame False {
          }
          frame True {
            n636 = local write "Tool voltage setpoint(V)"(w1328) -> ()
          }
        }
        n637 = case shown="True" w1297 {
          tunnel: w1295 -> [_ w1327]
          frame False {
          }
          frame True {
            n638 = local write "Resistance(Ohm)"(w1327) -> ()
          }
        }
        n639 = call "emi_Get DateTime In Seconds err & offs.vi"("error in (no error)"=w1323) -> ("Time"=w1309:timestamp, "error out"=w1310:errorcluster)  [unwired: 13 in]
        n640 = Subtract(x=w1309, y=w1308) -> (x-y=w1307:dbl)
        n641 = case shown="True" w1300 {
          tunnel: w1299 -> [_ w1329]
          frame False {
          }
          frame True {
            n642 = local write "Stroke setpoint"(w1329) -> ()
          }
        }
        n643 = Number To Fractional String(number=w1307, precision (6)=i16 0) -> (F-format string=w1305:string)  [unwired: 2 in]
        n644 = Bundle By Name(cluster=w1326, "Op button disabled"=w1313, "Perform action"=w1319, "Step index"=w1318, "Action time"=w1308) -> (w1325:T103)
        n645 = Concatenate Strings(w1305, " s") -> (w1303:string)
        n646 = local write "Time spent on sequence step"(w1303) -> ()
      }
      frame "Stop" {
        w1421 = User_Event_List."Sequence stopped" ("User Events")
        w1426 = T45."Disabled and Grayed Out" ("Disabled")
        w1418 = "" ("Sequence progress")
        # "Stop the loop. May be restarted later. Close interfaces and the like"
        n647 = call-poly "emi_SMLoop Control.vi"("Loop ID in"=w1425, "Enable"=FALSE, "error in (no error)"=w1428) -> ("error out"=w1417:errorcluster)  [unwired: 11 in, 1 out]
        n648 = property on="Sequence user input" class="DigNum (strict)"(error in=w1417, "Visible"=FALSE) -> (error out=w1416:errorcluster)  [unwired: 1 in, 1 out]
        n649 = local write "Next step"(w1418) -> ()
        n650 = local write "Current step"(w1418) -> ()
        n651 = local write "Sequence progress"(w1418) -> ()
        n652 = local write "Time spent on sequence step"(w1418) -> ()
        n653 = local write "Sequence user input name"(w1418) -> ()
        n654 = property on="Stopp sequence" class="Bool (strict)"(error in=w1416, "DisabledEnum"=w1426) -> (error out=w1427:errorcluster)  [unwired: 1 in, 1 out]
        n655 = property on="Approve step" class="Bool (strict)"(error in=w1427, "DisabledEnum"=w1426) -> (error out=w1413:errorcluster)  [unwired: 1 in, 1 out]
        n656 = property on="Start sequence" class="Bool (strict)"(error in=w1413, "DisabledEnum"=T45."Enabled" ("Disabled")) -> (error out=w1412:errorcluster)  [unwired: 1 in, 1 out]
        n657 = Format Into String(error in=w1412, w1421) -> (resulting string=w1420:string, error out=w1422:errorcluster)  [unwired: 2 in]
        n658 = call "Send S&E EVENT message.vi"("Event Source(user)"=S&E_Event_source."Application", "Event Description"=w1420, "error in (no error)"=w1422, "Loc Sub ID/Event ID(No ID)"=w1421) -> ("error out"=w1419:errorcluster)  [unwired: 10 in, 1 out]
      }
      frame "Error Handling" {
        # "Loop automaticaly returns here after error is found. If error is cleared, \nLoop wil continue as normal(if was operative when error."
      }
      frame "End" {
        # "Only executes at application end has. Should performa any action the loop \nneeds to finnish. Executes only once."
      }
      frame "Post" {
        # "Only exists to pas true to loop conditional without extra VI. DO Not edit"
      }
    }
  }
  n659 = while "Alarm Handling" {
    shift-right: [w1448] -> _
    shift-left: _ -> [w1445]
    shift-right: [w1446] -> _
    shift-left: w2 -> [w1443]
    tunnel: [w1437] -> _
    shift-right: [w1444] -> _
    shift-left: _ -> [w1439]
    tunnel: Loop_ID."Alarm Handling" ("Loop ID") -> [w1440]
    i -> [w1437]
    stop <- w1447 stop-if-true
    # "Alarm Handling"
    n660 = call "emi_SMLoop Start.vi"("Loop ID"=w1440, "error in (no error)"=w1443, "Force Stop(F)"=w1439) -> ("Loop command"=w1441:T102, "error out"=w1442:errorcluster, "Loop ID out"=w1438:i32)  [unwired: 10 in]
    n661 = case shown="\"Normal Operation\"" w1441 {
      tunnel: [w1451 w1453 w1457 w1503 w1683 w1686 w1687 w1690] -> w1448
      tunnel: [_ _ _ _ _ _ _ TRUE] -> w1447
      tunnel: w1442 -> [w1452 w1455 w1458 w1557 w1684 w1685 w1688 w1691]
      tunnel: [w1452 w1454 w1458 w1505 w1684 w1685 w1688 w1691] -> w1446
      tunnel: w1445 -> [_ w1453 w1457 w1503 w1683 w1686 w1687 w1690]
      tunnel: [w1449 _ _ _ _ _ _ _] -> w1444
      tunnel: w1438 -> [_ _ _ _ _ _ _ _]
      frame "Init" {
        w1449 = FALSE  # Force end
        w1450 = FALSE  # Placeholder
        # "First case that is executed, executes regardless of loop beeing enabled.\nOnly executes once. Init loop data and other variables."
        n662 = Bundle("Placeholder"=w1450) -> (w1451:cluster{"Placeholder":bool})  [unwired: 1 in]
      }
      frame "Standby", Default {
        # "Case that is executed when the loop is not enabled. Should not be edited."
        n663 = call "emi_Wait MS with err.vi"("milliseconds to wait(0)"=u32 50, "error in (no error)"=w1455) -> ("error out"=w1454:errorcluster)  [unwired: 13 in]
      }
      frame "Start" {
        # "Start or restart the loop. Should perform any init code. \nOpen channel and so on. Will perform each time the system is restarted."
      }
      frame "Normal Operation" {
        n664 = call "emi_Wait until MS multipl with Err.vi"("millisecond multiple(0)"=u32 1000, "error in (no error)"=w1557) -> ("error out"=w1470:errorcluster)  [unwired: 13 in]
        n665 = call "Options GFV.vi"("error in (no error)"=w1470) -> ("Options"=w1468:T60, "error out"=w1469:errorcluster)  [unwired: 16 in, 1 out]
        n666 = control-ref of="Voltage Down Hole"() -> (w1529:refnum<vi>)
        n667 = control-ref of="Voltage Topside"() -> (w1528:refnum<vi>)
        n668 = control-ref of="Current"() -> (w1527:refnum<vi>)
        n669 = control-ref of="Resistance"() -> (w1526:refnum<vi>)
        n670 = control-ref of="Depth"() -> (w1525:refnum<vi>)
        n671 = control-ref of="Speed"() -> (w1524:refnum<vi>)
        n672 = control-ref of="Tension"() -> (w1523:refnum<vi>)
        n673 = call "Get Analog Vars.vi"("Common alarm handling(F)"=TRUE, "Tool"=FALSE, "error in (no error)"=w1469) -> ("Catagorised  Stsaus"=w1538:T106[], "Any Alarm"=w1477:bool, "Primary Action"=w1463:T94, "Alarms"=w1499:bool[], "error out"=w1521:errorcluster)  [unwired: 6 in, 2 out]
        n674 = call "Selected Tool holder.vi"("error in (no error)"=w1521) -> ("Tool out"=w1548:T56, "error out"=w1520:errorcluster)  [unwired: 13 in]
        n675 = Build Array(w1529, w1528, w1527, w1526, w1525, w1524, w1523) -> (w1522:refnum<vi>[])
        n676 = Index Array(array=w1499) -> (element #1=w1498:bool, element #2=w1497:bool, element #3=w1496:bool, element #4=w1495:bool, element #5=w1494:bool, element #6=w1493:bool, element #7=w1492:bool)  [unwired: 7 in]
        n677 = Build Array(w1498, w1497, w1496, w1495, w1494, w1493, w1492) -> (w1491:bool[])
        n678 = call "Get Analog Vars.vi"("Common alarm handling(F)"=TRUE, "Tool"=TRUE, "error in (no error)"=w1520) -> ("Catagorised  Stsaus"=w1539:T106[], "Any Alarm"=w1476:bool, "Primary Action"=w1464:T94, "Alarms"=w1490:bool[], "error out"=w1519:errorcluster)  [unwired: 6 in, 2 out]
        n679 = case shown="\"Stroker\", Default" w1548 {
          selector: w1548 -> [w1644 w1667 w1682]
          tunnel: [w1644 w1667 w1682] -> w1542
          tunnel: w1519 -> [w1645 w1666 w1681]
          tunnel: [w1645 w1666 w1681] -> w1518
          tunnel: [w1642 w1662 w1679] -> w1502
          tunnel: w1522 -> [w1641 w1661 w1680]
          tunnel: w1491 -> [w1631 w1655 w1673]
          tunnel: w1490 -> [w1632 w1656 w1672]
          tunnel: [w1630 w1654 w1674] -> w1482
          tunnel: w1468 -> [w1629 _ _]
          frame "Stroker", Default {
            n680 = Unbundle By Name(w1629) -> ("P 4.Force det."=w1628:T66)
            n681 = control-ref of="Stroke force"() -> (w1643:refnum<vi>)
            n682 = control-ref of="\"Stroke out\" Pressure"() -> (w1627:refnum<vi>)
            n683 = control-ref of="\"Stroke in\" Pressure"() -> (w1626:refnum<vi>)
            n684 = control-ref of="Upper Tension Sub"() -> (w1640:refnum<vi>)
            n685 = control-ref of="Stroke Extension"() -> (w1639:refnum<vi>)
            n686 = case shown="\"Stroke in = node 1\", Default" w1628 {
              tunnel: w1627 -> [w1647 w1648]
              tunnel: w1626 -> [w1646 w1649]
              tunnel: [w1647 w1649] -> w1625
              tunnel: [w1646 w1648] -> w1624
              frame "Stroke in = node 1", Default {
              }
              frame "Strok out = node 1" {
              }
            }
            n687 = Index Array(array=w1632, index #1=Variable_List_Tool_Analog."Stroke Force" ("Variable ID"), index #2=Variable_List_Tool_Analog."Stroker Pressure 1" ("Variable ID"), index #3=Variable_List_Tool_Analog."Stroker Pressure 2" ("Variable ID"), index #4=Variable_List_Tool_Analog."Stroker Upper Tension Sub" ("Variable ID"), index #5=Variable_List_Tool_Analog."Stroke Extension" ("Variable ID"), index #6=Variable_List_Tool_Analog."Tool (Controller) Temperature" ("Variable ID")) -> (element #1=w1633:bool, element #2=w1634:bool, element #3=w1635:bool, element #4=w1636:bool, element #5=w1637:bool, element #6=w1638:bool)
            n688 = Build Array (concatenate)(w1631, w1633, w1634, w1635, w1636, w1637, w1638) -> (w1630:bool[])
            n689 = Build Array (concatenate)(w1641, w1643, w1625, w1624, w1640, w1639) -> (w1642:refnum<vi>[])
          }
          frame "Driller" {
            n690 = control-ref of="Weight on bit"() -> (w1663:refnum<vi>)
            n691 = control-ref of="Driller RPM"() -> (w1664:refnum<vi>)
            n692 = control-ref of="Torque"() -> (w1665:refnum<vi>)
            n693 = Index Array(array=w1656, index #1=Variable_List_Tool_Analog."Tool weight on bit" ("Variable ID"), index #2=Variable_List_Tool_Analog."Tool Motor RPM" ("Variable ID"), index #3=Variable_List_Tool_Analog."Tool Motor Torque" ("Variable ID"), index #4=Variable_List_Tool_Analog."Tool Max Temperature" ("Variable ID")) -> (element #1=w1657:bool, element #2=w1658:bool, element #3=w1659:bool, element #4=w1660:bool)
            n694 = Build Array (concatenate)(w1661, w1663, w1664, w1665) -> (w1662:refnum<vi>[])
            n695 = Build Array (concatenate)(w1655, w1657, w1658, w1659, w1660) -> (w1654:bool[])
          }
          frame "Tractor" {
            n696 = control-ref of="Trac - Upper Tension Sub"() -> (w1678:refnum<vi>)
            n697 = control-ref of="Trac - Lower Tension Sub"() -> (w1677:refnum<vi>)
            n698 = Index Array(array=w1672, index #1=Variable_List_Tool_Analog."Tractor Upper Tension Sub" ("Variable ID"), index #2=Variable_List_Tool_Analog."Tractor Lower Tension Sub" ("Variable ID"), index #3=Variable_List_Tool_Analog."Tool Max Temperature" ("Variable ID")) -> (element #1=w1675:bool, element #2=w1676:bool, element #3=w1671:bool)
            n699 = Build Array (concatenate)(w1680, w1678, w1677) -> (w1679:refnum<vi>[])
            n700 = Build Array (concatenate)(w1673, w1675, w1676, w1671) -> (w1674:bool[])
          }
        }
        n701 = Or(x=w1477, y=w1476) -> (x .or. y?=w1475:bool)
        n702 = Max & Min(x=w1464, y=w1463) -> (max(x,y)=w1466:u16)  [unwired: 1 out]
        n703 = call "Get Digital Vars.vi"("Common alarm handling(F)"=TRUE, "Tool"=FALSE, "error in (no error)"=w1518) -> ("Catagorised  Stsaus"=w1541:T106[], "Any Alarm"=w1474:bool, "Primary Action"=w1461:T94, "Alarms"=w1484:bool[], "error out"=w1530:errorcluster)  [unwired: 6 in, 2 out]
        n704 = Or(x=w1475, y=w1474) -> (x .or. y?=w1473:bool)
        n705 = control-ref of="Controller Temp."() -> (w1501:refnum<vi>)
        n706 = control-ref of="PCP"() -> (w1513:refnum<vi>)
        n707 = control-ref of="PCP Control"() -> (w1514:refnum<vi>)
        n708 = control-ref of="PSU"() -> (w1515:refnum<vi>)
        n709 = control-ref of="HV out"() -> (w1516:refnum<vi>)
        n710 = control-ref of="Tool"() -> (w1512:refnum<vi>)
        n711 = Index Array(array=w1484, index #5=Variable_List_Common_Digital."Tool Connected" ("Action")) -> (element #1=w1485:bool, element #2=w1486:bool, element #3=w1487:bool, element #4=w1488:bool, element #5=w1489:bool)  [unwired: 4 in]
        n712 = Build Array (concatenate)(w1502, w1501, w1513, w1514, w1515, w1516, w1512) -> (w1511:refnum<vi>[])
        n713 = Build Array (concatenate)(w1482, w1485, w1486, w1487, w1488, w1489) -> (w1481:bool[])
        n714 = call "Get Digital Vars.vi"("Common alarm handling(F)"=TRUE, "Tool"=TRUE, "error in (no error)"=w1530) -> ("Catagorised  Stsaus"=w1540:T106[], "Any Alarm"=w1472:bool, "Primary Action"=w1462:T94, "Alarms"=w1480:bool[], "error out"=w1517:errorcluster)  [unwired: 6 in, 2 out]
        n715 = Max & Min(x=w1462, y=w1461) -> (max(x,y)=w1467:u16)  [unwired: 1 out]
        n716 = case shown="\"Stroker\", Default" w1542 {
          tunnel: [w1590 w1605 w1617] -> w1478
          tunnel: w1517 -> [w1590 w1605 w1617]
          tunnel: w1511 -> [w1582 w1599 w1616]
          tunnel: [w1581 w1598 w1615] -> w1500
          tunnel: w1481 -> [w1573 w1601 w1608]
          tunnel: w1480 -> [w1572 w1602 w1609]
          tunnel: [w1571 w1600 w1610] -> w1479
          frame "Stroker", Default {
            n717 = control-ref of="Pressure 1"() -> (w1589:refnum<vi>)
            n718 = control-ref of="Pressure 2"() -> (w1587:refnum<vi>)
            n719 = control-ref of="Solenoid"() -> (w1588:refnum<vi>)
            n720 = control-ref of="Strok Tension Sub 1"() -> (w1586:refnum<vi>)
            n721 = control-ref of="Str Error P1"() -> (w1585:refnum<vi>)
            n722 = control-ref of="Str Error P2"() -> (w1584:refnum<vi>)
            n723 = control-ref of="Str Error Sol"() -> (w1583:refnum<vi>)
            n724 = Build Array (concatenate)(w1582, w1589, w1587, w1588, w1586, w1585, w1584, w1583) -> (w1581:refnum<vi>[])
            n725 = Index Array(array=w1572, index #1=Variable_List_Tool_Digital."Tool node Pressure 1", index #2=Variable_List_Tool_Digital."Tool node Pressure 2", index #3=Variable_List_Tool_Digital."Tool node Solenoid", index #4=Variable_List_Tool_Digital."Upper Tension Sub", index #5=Variable_List_Tool_Digital."Tool node Pressure 1", index #6=Variable_List_Tool_Digital."Tool node Pressure 2", index #7=Variable_List_Tool_Digital."Tool node Solenoid") -> (element #1=w1579:bool, element #2=w1578:bool, element #3=w1577:bool, element #4=w1576:bool, element #5=w1575:bool, element #6=w1574:bool, element #7=w1580:bool)
            n726 = Build Array (concatenate)(w1573, w1579, w1578, w1577, w1576, w1575, w1574, w1580) -> (w1571:bool[])
          }
          frame "Driller" {
            n727 = control-ref of="Dr Pressure 1"() -> (w1597:refnum<vi>)
            n728 = control-ref of="Dr Pressure 2"() -> (w1596:refnum<vi>)
            n729 = control-ref of="Dr Solenoid"() -> (w1595:refnum<vi>)
            n730 = Build Array (concatenate)(w1599, w1597, w1596, w1595) -> (w1598:refnum<vi>[])
            n731 = Index Array(array=w1602, index #1=Variable_List_Tool_Digital."Tool node Pressure 1", index #2=Variable_List_Tool_Digital."Tool node Pressure 2", index #3=Variable_List_Tool_Digital."Tool node Solenoid") -> (element #1=w1604:bool, element #2=w1603:bool, element #3=w1594:bool)
            n732 = Build Array (concatenate)(w1601, w1604, w1603, w1594) -> (w1600:bool[])
          }
          frame "Tractor" {
            n733 = control-ref of="Trac Tension Sub 1"() -> (w1614:refnum<vi>)
            n734 = control-ref of="Trac Tension Sub 2"() -> (w1613:refnum<vi>)
            n735 = Build Array (concatenate)(w1616, w1614, w1613) -> (w1615:refnum<vi>[])
            n736 = Index Array(array=w1609, index #1=Variable_List_Tool_Digital."Upper Tension Sub", index #2=Variable_List_Tool_Digital."Lower Tension Sub") -> (element #1=w1612:bool, element #2=w1611:bool)
            n737 = Build Array (concatenate)(w1608, w1612, w1611) -> (w1610:bool[])
          }
        }
        n738 = Or(x=w1473, y=w1472) -> (x .or. y?=w1471:bool)
        "Alarm" <- w1471
        n739 = control-ref of="General level"() -> (w1536:refnum<vi>)
        n740 = control-ref of="Power Level"() -> (w1535:refnum<vi>)
        n741 = control-ref of="Temp level"() -> (w1534:refnum<vi>)
        n742 = control-ref of="Press level"() -> (w1533:refnum<vi>)
        n743 = Build Array (concatenate)(w1536, w1535, w1534, w1533, w1500) -> (w1532:refnum<vi>[])
        n744 = Max & Min(x=w1467, y=w1466) -> (max(x,y)=w1465:u16)  [unwired: 1 out]
        n745 = call "Catagoried alarms combine.vi"("Catagorised  Stsaus 1"=w1538, "Catagorised  Stsaus 2"=w1539, "Catagorised  Stsaus 3"=w1541, "Catagorised  Stsaus 4"=w1540) -> ("catagorised Status out"=w1545:T106[], "Catagoried alarms out"=w1537:bool[])  [unwired: 10 in]
        n746 = call "Action executor.vi"("Action"=w1465) -> ("Stop Motor"=w1460:bool, "P 3.Stop Motor Voltage"=w1459:dbl)  [unwired: 12 in, 1 out]
        n747 = Build Array (concatenate)(w1537, w1479) -> (w1531:bool[])
        n748 = case shown="True" w1460 {
          tunnel: w1459 -> [_ w1560]
          frame False {
          }
          frame True {
            n749 = local write "Tool voltage setpoint(V)"(w1560) -> ()
            n750 = local write "Start Motor"(FALSE ("Start Motor")) -> ()
          }
        }
        n751 = call "Array of bluinking controllers.vi"("Controls"=w1532, "Blinking"=w1531, "error in"=w1478) -> ("error out"=w1504:errorcluster)  [unwired: 12 in]
        n752 = Index Array(array=w1545) -> (element #1=→"General level":T106, element #2=→"Power Level":T106, element #3=→"Temp level":T106, element #4=→"Press level":T106)  [unwired: 4 in]
        n753 = call "Get Alarm State.vi"("error in (no error)"=w1504) -> ("Alarm state"=w1507:string[][], "updated"=w1509:bool, "error out"=w1508:errorcluster)  [unwired: 12 in]
        n754 = case shown="True" w1509 {
          tunnel: [w1561 w1563] -> w1506
          tunnel: w1508 -> [w1561 w1563]
          tunnel: w1507 -> [_ w1562]
          frame False {
          }
          frame True {
            "Alarms" <- w1562
          }
        }
        n755 = call "Alarma.vi"("Action(GET)"=enum16{"GET", "SET"}."SET", "error in (no error)"=w1506, "Alarma in"=w1471) -> ("error out"=w1505:errorcluster)  [unwired: 7 in, 1 out]
      }
      frame "Stop" {
        # "Stop the loop. May be restarted later. Close interfaces and the like"
      }
      frame "Error Handling" {
        # "Loop automaticaly returns here after error is found. If error is cleared, \nLoop wil continue as normal(if was operative when error."
      }
      frame "End" {
        # "Only executes at application end has. Should performa any action the loop \nneeds to finnish. Executes only once."
      }
      frame "Post" {
        # "Only exists to pas true to loop conditional without extra VI. DO Not edit"
      }
    }
  }
  n756 = while "Periodically update control properties" {
    shift-right: [w1703] -> _
    shift-left: _ -> [w1699]
    shift-right: [w1701] -> _
    shift-left: w2 -> [w1697]
    tunnel: [w1700] -> _
    shift-right: [w1698] -> _
    shift-left: _ -> [w1693]
    tunnel: Loop_ID."Main-Ind Upd" ("Loop ID") -> [w1694]
    i -> [w1700]
    stop <- w1702 stop-if-true
    n757 = call "emi_SMLoop Start.vi"("Loop ID"=w1694, "error in (no error)"=w1697, "Force Stop(F)"=w1693) -> ("Loop command"=w1695:T102, "error out"=w1696:errorcluster, "Loop ID out"=w1692:i32)  [unwired: 10 in]
    n758 = case shown="\"Normal Operation\"" w1695 {
      tunnel: [w1707 w1709 w1713 w1724 w1888 w1890 w1891 w1894] -> w1703
      tunnel: [_ _ _ _ _ _ _ TRUE] -> w1702
      tunnel: w1696 -> [w1708 w1711 w1714 w1725 w1887 w1889 w1892 w1895]
      tunnel: [w1708 w1710 w1714 w1718 w1887 w1889 w1892 w1895] -> w1701
      tunnel: w1699 -> [_ w1709 w1713 w1724 w1888 w1890 w1891 w1894]
      tunnel: [w1705 _ _ FALSE ("Force End") _ _ _ _] -> w1698
      tunnel: w1692 -> [_ _ _ _ _ _ _ _]
      frame "Init" {
        w1705 = FALSE  # Force end
        w1706 = FALSE  # Placeholder
        # "First case that is executed, executes regardless of loop beeing enabled.\nOnly executes once. Init loop data and other variables."
        n759 = Wait (ms)(milliseconds to wait=u32 200) -> ()  [unwired: 1 out]
        n760 = Bundle("Placeholder"=w1706) -> (w1707:cluster{"Placeholder":bool})  [unwired: 1 in]
      }
      frame "Standby", Default {
        # "Case that is executed when the loop is not enabled. Should not be edited."
        n761 = call "emi_Wait MS with err.vi"("milliseconds to wait(0)"=u32 50, "error in (no error)"=w1711) -> ("error out"=w1710:errorcluster)  [unwired: 13 in]
      }
      frame "Start" {
        # "Start or restart the loop. Should perform any init code. \nOpen channel and so on. Will perform each time the system is restarted."
      }
      frame "Normal Operation" {
        w1717 = 4 ("Index(0)")
        # "All normal tasks belong here. This will be repeated, until error, disable, restart or\nforsed to restart. OBS, reduce overhead with internal loop(will execute unevenly)."
        n762 = call "emi_Wait until MS multipl with Err.vi"("millisecond multiple(0)"=u32 500 ("milliseconds to wait(0)"), "error in (no error)"=w1725) -> ("error out"=w1721:errorcluster)  [unwired: 13 in]
        n763 = control-ref of="This VI"() -> (w1716:refnum<vi>)
        n764 = disable-structure shown="Disabled" {
          disable-tunnel: w1721 -> [w1731 w1732]
          disable-tunnel: [w1730 w1732] -> w1720
          disable-tunnel: w1717 -> [w1729 _]
          disable-tunnel: w1716 -> [w1727 _]
          disable-tunnel: [w1726 _] -> w1715
          frame Disabled {
            n765 = call "Set pannel updating true.vi"("error in"=w1731, "Index(0)"=w1729) -> ("error out"=w1728:errorcluster)  [unwired: 5 in]
            n766 = call "emi_Defer Panel Updates ON.vi"("VI Refnum(This VI)"=w1727, "error in (no error)"=w1728) -> ("VI Refnum Out"=w1726:refnum<vi>, "error out"=w1730:errorcluster)  [unwired: 12 in]
          }
          frame Enabled {
          }
        }
        n767 = flat-sequence {
          tunnel: [w1823] -> w1719
          tunnel: w1720 -> [w1782]
          frame #0 {
            w1755 = Variable_List_Common_Digital."Tool Connected" ("Digital Signal")
            w1802 = Status_Digitalish."True" ("y")
            n768 = call "Get Analog Vars.vi"("Common alarm handling(F)"=FALSE, "Tool"=TRUE, "error in (no error)"=w1782) -> ("Values"=w1781:dbl[])  [unwired: 6 in, 6 out]
            n769 = call "Get Analog Vars.vi"("Common alarm handling(F)"=FALSE, "Tool"=FALSE, "error in (no error)"=w1782) -> ("Values"=w1810:dbl[], "error out"=w1770:errorcluster)  [unwired: 6 in, 5 out]
            n770 = call "Get Digital Vars.vi"("Common alarm handling(F)"=FALSE, "Tool"=TRUE, "error in (no error)"=w1782) -> ("Values"=w1745:T108[], "error out"=w1796:errorcluster)  [unwired: 6 in, 5 out]
            n771 = call "Get Digital Vars.vi"("Common alarm handling(F)"=FALSE, "Tool"=FALSE, "error in (no error)"=w1782) -> ("Values"=w1756:T108[], "error out"=w1780:errorcluster)  [unwired: 6 in, 5 out]
            n772 = Index Array(array=w1745, index=Variable_List_Tool_Digital."Tool Both Relays") -> (element=w1742:T108)
            n773 = Index Array(array=w1756, index #1=Variable_List_Common_Digital."PCP PC Control" ("Action"), index #2=Variable_List_Common_Digital."PCP Connected" ("Action"), index #3=Variable_List_Common_Digital."Tool Connected" ("Action"), index #4=Variable_List_Common_Digital."HV PSU HV Active" ("Action")) -> (element #1=w1816:T108, element #2=w1801:T108, element #3=w1791:T108, element #4=w1787:T108)
            n774 = Equal?(x=w1742, y=Status_Digitalish."NA") -> (x = y?=w1741:bool)
            n775 = call "Selected Tool holder.vi"("error in (no error)"=w1796) -> ("Tool out"=w1795:T56)  [unwired: 13 in, 1 out]
            n776 = Index Array(array=w1810, index #1=Variable_List_Common_Analog."HVPSU Head Voltage" ("First part list"), index #2=Variable_List_Common_Analog."PCP Cable Resistance" ("First part list")) -> (element #1=w1746:dbl, element #2=w1797:dbl)
            n777 = Equal?(x=w1816, y=Status_Digitalish."False") -> (x = y?=w1818:bool)
            n778 = Equal?(x=w1816, y=w1802) -> (x = y?=w1803:bool)
            n779 = Equal?(x=w1801, y=w1802) -> (x = y?=w1800:bool)
            n780 = Equal?(x=w1791, y=Status_Digitalish."True") -> (x = y?=w1739:bool)
            n781 = And(x=w1739, y=w1741) -> (x .and. y?=w1740:bool)
            n782 = property on="Relay Status" class="Clust (strict)"("Blinking"=w1740) -> ()  [unwired: 2 in, 2 out]
            n783 = Equal?(x=w1787, y=Status_Digitalish."True") -> (x = y?=w1786:bool)
            n784 = local read "Tool voltage setpoint(V)"() -> (w1808:dbl)
            n785 = case shown="\"Stroker\"" w1795 {
              tunnel: w1745 -> [_ w1837]
              frame "Driller", Default {
              }
              frame "Stroker" {
                n786 = control-ref of="Stroker Stroke Go To"() -> (w1839:refnum<vi>)
                n787 = control-ref of="Stroker Stroke Out"() -> (w1840:refnum<vi>)
                n788 = control-ref of="Stroker Stroke In"() -> (w1841:refnum<vi>)
                n789 = call "Set command buttons blinking.vi"("Go To Ref"=w1839, "Values"=w1837, "In Ref"=w1841, "Out Ref"=w1840) -> ()  [unwired: 7 in, 1 out]
                n790 = Index Array(array=w1837, index=Variable_List_Tool_Digital."Stroke Target seeking") -> (element=w1843:T108)
                n791 = Equal?(x=w1843, y=Status_Digitalish."True") -> (x = y?=w1842:bool)
                n792 = property on="Distance from target:" class="DigNum (strict)"("Visible"=w1842) -> ()  [unwired: 2 in, 2 out]
                n793 = control-ref of="Slips total"() -> (w1838:refnum<vi>)
                n794 = call "Set font color of buttons.vi"("index"=Variable_List_Tool_Digital."Stroke SLIPS established", "Values"=w1837, "Ctrl Ref"=w1838) -> ()  [unwired: 8 in, 1 out]
              }
            }
            n795 = call "Options GFV.vi"() -> ("Options"=w1748:T60)  [unwired: 17 in, 2 out]
            n796 = Unbundle By Name(w1748) -> ("P 3.Relay Status Loss Voltage"=w1747:dbl)
            n797 = Less?(x=w1746, y=10.0) -> (x < y?=w1807:bool)
            n798 = call "PCP connected and PC controlled.vi"("Action(GET)"=enum16{"GET", "SET"}."SET", "PCP connected  in"=w1800, "PCP PC controlled in"=w1803) -> ()  [unwired: 10 in, 3 out]
            n799 = call "PCP Voltage AND resistance value read.vi"("Action(GET)"=enum16{"GET", "SET"}."SET", "PCP resistance"=w1797, "PCP voltage"=w1746) -> ()  [unwired: 10 in, 3 out]
            n800 = Equal To 0?(x=w1808) -> (x = 0?=w1806:bool)
            n801 = And(x=w1807, y=w1806) -> (x .and. y?=w1804:bool)
            n802 = call "PCP HV on OK.vi"("Action(GET)"=enum16{"GET", "SET"}."SET", "PCP HV on OK"=w1804, "Telemetry Started"=w1739, "HV Active"=w1786) -> ()  [unwired: 8 in, 4 out]
            n803 = Not A Number/Path/Refnum?(number/path/refnum=w1746) -> (NaN/Path/Refnum?=w1751:bool)
            n804 = Less?(x=w1746, y=w1747) -> (x < y?=w1752:bool)
            n805 = Not(x=w1751) -> (.not. x?=w1750:bool)
            n806 = control-ref of="Start Telemetry"() -> (w1764:refnum<vi>)
            n807 = control-ref of="HV ON"() -> (w1793:refnum<vi>)
            n808 = And(x=w1750, y=w1752) -> (x .and. y?=w1749:bool)
            n809 = case shown="True" w1749 {
              frame False {
              }
              frame True {
                w1824 = FALSE ("Relay 1 Initialized")
                # "2015-06-23 v1.16 OOS\nIf TS voltage is less than a set limit\nthe relay initialized state is cleared"
                n810 = call "Tool Relay State Initialized.vi"("Action(GET)"=enum16{"GET", "SET"}."SET", "Relay 1 Initialized"=w1824, "Relay 2 Initialized"=w1824) -> ()  [unwired: 10 in, 3 out]
              }
            }
            n811 = call "Set color of CMD buttons.vi"("Color OFF"=u32 32832, "Color ON"=u32 7204608, "Var Index"=Variable_List_Common_Digital."HV PSU HV Active" ("Action"), "Values"=w1756, "Ctrl ref"=w1793) -> ("error out"=w1765:errorcluster)  [unwired: 6 in]
            n812 = call "Set color of CMD buttons.vi"("Color OFF"=u32 12369084, "Color ON"=u32 7204608, "error in (no error)"=w1765, "Var Index"=Variable_List_Common_Digital."Tool Connected" ("Action"), "Values"=w1756, "Ctrl ref"=w1764) -> ("error out"=w1757:errorcluster)  [unwired: 5 in]
            n813 = case shown="False" w1818 {
              tunnel: w1810 -> [w1856 w1886]
              tunnel: w1781 -> [w1855 _]
              tunnel: w1780 -> [w1857 w1880]
              tunnel: [w1854 w1879] -> w1779
              tunnel: "Calculate resistance" -> [w1848 _]
              frame False {
                w1850 = 2 ("Samples to average")
                n814 = Index Array(array=w1855, index=Variable_List_Tool_Analog."Head Voltage" ("Variable ID")) -> (element=w1851:dbl)
                n815 = Index Array(array=w1856, index #1=Variable_List_Common_Analog."HVPSU TS Voltage" ("First part list"), index #2=Variable_List_Common_Analog."HVPSU Current" ("First part list")) -> (element #1=w1852:dbl, element #2=w1853:dbl)
                n816 = call "Average DBL.vi"("Samples to average"=w1850, "Data in"=w1851) -> ("Averaged data out"=w1847:dbl)  [unwired: 9 in]
                n817 = call "Average DBL.vi"("Samples to average"=w1850, "Data in"=w1852) -> ("Averaged data out"=w1845:dbl)  [unwired: 9 in]
                n818 = call "Average DBL.vi"("Samples to average"=w1850, "Data in"=w1853) -> ("Averaged data out"=w1846:dbl)  [unwired: 9 in]
                n819 = case shown="True" w1848 {
                  tunnel: w1857 -> [w1860 w1870]
                  tunnel: [w1860 w1867] -> w1854
                  tunnel: w1847 -> [_ w1876]
                  tunnel: w1846 -> [_ w1875]
                  tunnel: w1845 -> [_ w1874]
                  frame False {
                  }
                  frame True {
                    # "Remote (PC Control)\nCalculate resistance when button pressed"
                    n820 = Subtract(x=w1874, y=w1876) -> (x-y=w1877:dbl)
                    n821 = call "Options GFV.vi"("error in (no error)"=w1870) -> ("Options"=w1873:T60, "error out"=w1868:errorcluster)  [unwired: 16 in, 1 out]
                    n822 = Divide(x=w1877, y=w1875) -> (x/y=w1869:dbl)
                    n823 = Unbundle By Name(w1873) -> ("P 3.Max resistance"=w1872:dbl, "P 3.Min resistance"=w1871:dbl)
                    n824 = In Range and Coerce(upper limit=w1872, x=w1869, lower limit=w1871) -> (coerced(x)=w1862:dbl, In Range?=w1866:bool)
                    n825 = Not A Number/Path/Refnum?(number/path/refnum=w1862) -> (NaN/Path/Refnum?=w1861:bool)
                    n826 = case shown="False" w1861 {
                      tunnel: w1862 -> [w1878 _]
                      frame False {
                        n827 = local write "Resistance(Ohm)"(w1878) -> ()
                      }
                      frame True {
                      }
                    }
                    n828 = Select(t=u32 16776960, s=w1866, f=u32 16722474) -> (s? t:f=w1863:u32)
                    n829 = property on="Resistance(Ohm)" class="DigNum (strict)"(error in=w1868, "NumText.BG Color"=w1863) -> (error out=w1867:errorcluster)  [unwired: 1 in, 1 out]
                  }
                }
              }
              frame True {
                # "Local"
                n830 = Index Array(array=w1886, index #1=Variable_List_Common_Analog."HVPSU Head Voltage" ("First part list"), index #2=Variable_List_Common_Analog."PCP Cable Resistance" ("First part list")) -> (element #1=w1881:dbl, element #2=w1882:dbl)
                n831 = local write "Tool voltage setpoint(V)"(w1881) -> ()
                n832 = local write "Resistance(Ohm)"(w1882) -> ()
                n833 = call "PC send voltage and resistance when in local mode.vi"("Resistance"=w1882, "Voltage"=w1881, "error in (no error)"=w1880) -> ("error out"=w1883:errorcluster)  [unwired: 12 in]
                n834 = call <vilib>:"Clear Errors.vi"("error in (no error)"=w1883) -> ("error out"=w1879:errorcluster)  [unwired: 6 in]
              }
            }
            n835 = call "Reset flashing button.vi"("error in (no error)"=w1757, "Digital Values"=w1756, "Digital Signal Index"=w1755, "Controll collection"=Controll_refrence_groups."PCP Start Telemetry") -> ()  [unwired: 7 in, 1 out]
            n836 = call "Modem Status Interpret Data.vi"() -> ("Subsea Bar Graph"=→"Subsea Bar Graph":T1, "Topside Bar Graph"=→"Topside Bar Graph":T1)  [unwired: 10 in]
            n837 = call "Check if boolean value changed.vi"("Var Index"=w1755, "Values"=w1756) -> ("Value"=w1753:bool, "Value Changed"=w1754:bool)  [unwired: 8 in]
            n838 = call "Set contrls enabled disabled.vi"("error in (no error)"=w1770) -> ("error out"=w1771:errorcluster)  [unwired: 14 in]
            n839 = case shown="True" w1754 {
              tunnel: w1753 -> [_ w1826]
              frame False {
              }
              frame True {
                n840 = local write "Start Telemetry"(w1826) -> ()
              }
            }
            n841 = call "GFV project info.vi"() -> ("Project info out"=w1775:T96)  [unwired: 14 in, 1 out]
            n842 = Unbundle By Name(w1775) -> ("data.Run Information.Active Run"=w1774:bool, "data.Run Information.String Check Rec"=w1773:bool, "data.Run Information.Run Number"=w1772:i32)
            n843 = call "Enable or Disable PCP controls.vi"("error in (no error)"=w1771) -> ("error out"=w1767:errorcluster)  [unwired: 14 in]
            n844 = case shown="True" w1774 {
              tunnel: w1772 -> [_ w1834]
              tunnel: [w1827 w1831] -> w1777
              tunnel: w1773 -> [w1830 _]
              frame False {
                n845 = Select(t="Recording String Check", s=w1830, f="Idle") -> (s? t:f=w1827:string)
              }
              frame True {
                n846 = Number To Decimal String(number=w1834) -> (decimal integer string=w1832:string)  [unwired: 1 in]
                n847 = Concatenate Strings("Recording Run " ("string"), w1832) -> (w1831:string)
              }
            }
            "Recording Status" <- w1777
            n848 = Or(x=w1774, y=w1773) -> (x .or. y?=→"Recording":bool)
            n849 = call "Enable or Disable Modem Status Controls.vi"("error in (no error)"=w1767) -> ("error out"=w1766:errorcluster)  [unwired: 14 in]
            n850 = Merge Errors(w1766, w1779) -> (w1823:errorcluster)
          }
        }
        n851 = disable-structure shown="Disabled" {
          disable-tunnel: w1719 -> [w1736 w1738]
          disable-tunnel: [w1735 w1738] -> w1718
          disable-tunnel: w1717 -> [w1734 _]
          disable-tunnel: w1715 -> [w1733 _]
          frame Disabled {
            n852 = call "emi_Defer Panel Updates OFF.vi"("VI Refnum(This VI)"=w1733, "error in (no error)"=w1736) -> ("error out"=w1737:errorcluster)  [unwired: 12 in, 1 out]
            n853 = call "Set pannel updating false.vi"("error in"=w1737, "Index(0)"=w1734) -> ("error out"=w1735:errorcluster)  [unwired: 5 in]
          }
          frame Enabled {
          }
        }
      }
      frame "Stop" {
        # "Stop the loop. May be restarted later. Close interfaces and the like"
      }
      frame "Error Handling" {
        # "Loop automaticaly returns here after error is found. If error is cleared, \nLoop wil continue as normal(if was operative when error."
      }
      frame "End" {
        # "Only executes at application end has. Should performa any action the loop \nneeds to finnish. Executes only once."
      }
      frame "Post" {
        # "Only exists to pas true to loop conditional without extra VI. DO Not edit"
      }
    }
  }
  n854 = while "Indicator value update" {
    shift-right: [w1907] -> _
    shift-left: _ -> [w1903]
    shift-right: [w1905] -> _
    shift-left: w2 -> [w1901]
    tunnel: [w1904] -> _
    shift-right: [w1902] -> _
    shift-left: _ -> [w1897]
    tunnel: Loop_ID."Indicator Value Update" ("Loop ID") -> [w1898]
    i -> [w1904]
    stop <- w1906 stop-if-true
    # "Indicator value update"
    n855 = call "emi_SMLoop Start.vi"("Loop ID"=w1898, "error in (no error)"=w1901, "Force Stop(F)"=w1897) -> ("Loop command"=w1899:T102, "error out"=w1900:errorcluster, "Loop ID out"=w1896:i32)  [unwired: 10 in]
    n856 = case shown="\"Normal Operation\"" w1899 {
      tunnel: [w1910 w1912 w1916 w1969 w2120 w2123 w2124 w2127] -> w1907
      tunnel: [_ _ _ _ _ _ _ TRUE] -> w1906
      tunnel: w1900 -> [w1911 w1914 w1917 w1970 w2121 w2122 w2125 w2128]
      tunnel: [w1911 w1913 w1917 w1930 w2121 w2122 w2125 w2128] -> w1905
      tunnel: w1903 -> [_ w1912 w1916 w1969 w2120 w2123 w2124 w2127]
      tunnel: [w1908 _ _ FALSE ("Force End") _ _ _ _] -> w1902
      tunnel: w1896 -> [_ _ _ _ _ _ _ _]
      frame "Init" {
        w1908 = FALSE  # Force end
        w1909 = FALSE  # Placeholder
        # "First case that is executed, executes regardless of loop beeing enabled.\nOnly executes once. Init loop data and other variables."
        n857 = Bundle("Placeholder"=w1909) -> (w1910:cluster{"Placeholder":bool})  [unwired: 1 in]
      }
      frame "Standby", Default {
        # "Case that is executed when the loop is not enabled. Should not be edited."
        n858 = call "emi_Wait MS with err.vi"("milliseconds to wait(0)"=u32 50, "error in (no error)"=w1914) -> ("error out"=w1913:errorcluster)  [unwired: 13 in]
      }
      frame "Start" {
        # "Start or restart the loop. Should perform any init code. \nOpen channel and so on. Will perform each time the system is restarted."
      }
      frame "Normal Operation" {
        # "Digital Data"
        # "Analog Data"
        # "All normal tasks belong here. This will be repeated, until error, disable, restart or\nforsed to restart. OBS, reduce overhead with internal loop(will execute unevenly)."
        n859 = call "emi_Wait until MS multipl with Err.vi"("millisecond multiple(0)"=u32 100, "error in (no error)"=w1970) -> ("error out"=w1933:errorcluster)  [unwired: 13 in]
        n860 = call "Options GFV.vi"("error in (no error)"=w1933) -> ("Options"=w1921:T60, "error out"=w1932:errorcluster)  [unwired: 16 in, 1 out]
        n861 = Unbundle By Name(w1921) -> ("P 3.Samples to average"=w1920:i32)
        n862 = call "Get Analog Vars.vi"("Common alarm handling(F)"=FALSE, "Tool"=FALSE, "error in (no error)"=w1932) -> ("Analog Vars"=w1964:T10[], "error out"=w1958:errorcluster)  [unwired: 6 in, 5 out]
        n863 = call "Selected Tool holder.vi"("error in (no error)"=w1958) -> ("Tool out"=w1957:T56, "error out"=w1956:errorcluster)  [unwired: 13 in]
        n864 = Index Array(array=w1964) -> (element #1=w1924:T10, element #2=w1923:T10, element #3=w1922:T10, element #4=→"Resistance":T10, element #5=→"Depth":T10, element #6=→"Speed":T10, element #7=w1929:T10)  [unwired: 7 in]
        n865 = call "Average.vi"("Samples to average"=w1920, "Data inn"=w1924) -> ("Averaged data out"=→"Voltage Down Hole":T10)  [unwired: 9 in]
        n866 = call "Average.vi"("Samples to average"=w1920, "Data inn"=w1923) -> ("Averaged data out"=→"Voltage Topside":T10)  [unwired: 9 in]
        n867 = call "Average.vi"("Samples to average"=w1920, "Data inn"=w1922) -> ("Averaged data out"=→"Current":T10)  [unwired: 9 in]
        n868 = call "Average.vi"("Samples to average"=w1920, "Data inn"=w1929) -> ("Averaged data out"=→"Tension":T10)  [unwired: 9 in]
        n869 = call "Get Analog Vars.vi"("Common alarm handling(F)"=FALSE, "Tool"=TRUE, "error in (no error)"=w1956) -> ("Values"=w1953:dbl[], "Analog Vars"=w1954:T10[], "error out"=w1955:errorcluster)  [unwired: 6 in, 4 out]
        n870 = case shown="\"Stroker\", Default" w1957 {
          selector: w1957 -> [w2071 w2095 w2118]
          tunnel: w1955 -> [w2074 w2100 w2117]
          tunnel: w1954 -> [w2080 w2104 w2116]
          tunnel: w1953 -> [w2078 w2099 w2112]
          tunnel: [w2074 w2100 w2117] -> w1949
          tunnel: [w2073 w2098 w2111] -> w1952
          tunnel: [w2072 w2097 w2110] -> w1951
          tunnel: [w2048 w2096 w2113] -> w1950
          tunnel: [w2071 w2095 w2118] -> w1945
          tunnel: w1921 -> [w2069 w2094 w2119]
          tunnel: [w2069 w2094 w2119] -> w1931
          frame "Stroker", Default {
            # "v1.13.0 only stroke force indicator is absolute\ngraph still shows pos and neg values"
            n871 = Unbundle By Name(w2069) -> ("P 4.Force det."=w2070:T66)
            n872 = local read "Stroke setpoint"() -> (w2083:dbl)
            n873 = Index Array(array=w2080, index #1=Variable_List_Tool_Analog."Stroke Force" ("Variable ID"), index #2=Variable_List_Tool_Analog."Stroker Pressure 1" ("Variable ID"), index #3=Variable_List_Tool_Analog."Stroker Pressure 2" ("Variable ID"), index #4=Variable_List_Tool_Analog."Stroker Upper Tension Sub" ("Variable ID"), index #5=Variable_List_Tool_Analog."Stroke Extension" ("Variable ID"), index #6=Variable_List_Tool_Analog."Tool Max Temperature" ("Variable ID")) -> (element #1=w2054:T10, element #2=w2068:T10, element #3=w2067:T10, element #4=→"Upper Tension Sub":T10, element #5=→"Stroke extenstion":T10, element #6=w2048:T10)
            n874 = Index Array(array=w2078, index #1=Variable_List_Tool_Analog."Stroke Extension" ("Variable ID"), index #2=Variable_List_Tool_Analog."Stroke Extension" ("Variable ID"), index #3=Variable_List_Tool_Analog."Stroke Extension" ("Variable ID"), index #4=Variable_List_Tool_Analog."Tool Inclination" ("Variable ID"), index #5=Variable_List_Tool_Analog."Tool Rotation" ("Variable ID")) -> (element #1=w2077:dbl, element #2=→"Stroker":dbl, element #3=→"Stroker  2":dbl, element #4=w2073:dbl, element #5=w2072:dbl)
            n875 = Subtract(x=w2083, y=w2077) -> (x-y=w2081:dbl)
            n876 = Unbundle By Name(w2054) -> ("Value"=w2055:dbl)
            n877 = case shown="\"Stroke in = node 1\", Default" w2070 {
              tunnel: w2068 -> [w2085 w2086]
              tunnel: w2067 -> [w2084 w2087]
              tunnel: [w2085 w2087] -> w2065
              tunnel: [w2084 w2086] -> w2066
              frame "Stroke in = node 1", Default {
              }
              frame "Strok out = node 1" {
              }
            }
            "\"Stroke in\" Pressure" <- w2066
            "\"Stroke out\" Pressure" <- w2065
            n878 = Absolute Value(x=w2081) -> (abs(x)=→"Distance from target:":dbl)
            n879 = Absolute Value(x=w2055) -> (abs(x)=w2053:dbl)
            n880 = Bundle By Name(cluster=w2054, "Value"=w2053) -> (→"Stroke force":T10)
          }
          frame "Driller" {
            n881 = Index Array(array=w2104, index #1=Variable_List_Tool_Analog."Tool weight on bit" ("Variable ID"), index #2=Variable_List_Tool_Analog."Tool Motor RPM" ("Variable ID"), index #3=Variable_List_Tool_Analog."Tool Motor Torque" ("Variable ID"), index #4=Variable_List_Tool_Analog."Tool Max Temperature" ("Variable ID")) -> (element #1=→"Weight on bit":T10, element #2=→"Driller RPM":T10, element #3=→"Torque":T10, element #4=w2096:T10)
            n882 = Index Array(array=w2099, index #1=Variable_List_Tool_Analog."Tool Inclination" ("Variable ID"), index #2=Variable_List_Tool_Analog."Tool Rotation" ("Variable ID")) -> (element #1=w2098:dbl, element #2=w2097:dbl)
          }
          frame "Tractor" {
            n883 = Index Array(array=w2116, index #1=Variable_List_Tool_Analog."Tractor Upper Tension Sub" ("Variable ID"), index #2=Variable_List_Tool_Analog."Tractor Lower Tension Sub" ("Variable ID"), index #3=Variable_List_Tool_Analog."Tool Max Temperature" ("Variable ID")) -> (element #1=→"Trac - Upper Tension Sub":T10, element #2=→"Trac - Lower Tension Sub":T10, element #3=w2113:T10)
            n884 = Index Array(array=w2112, index #1=Variable_List_Tool_Analog."Tool Inclination" ("Variable ID"), index #2=Variable_List_Tool_Analog."Tool Rotation" ("Variable ID")) -> (element #1=w2111:dbl, element #2=w2110:dbl)
          }
        }
        "Tool Angle" <- w1952
        "Controller Temp." <- w1950
        "Tool Rotation" <- w1951
        n885 = call "Get Digital Vars.vi"("Common alarm handling(F)"=FALSE, "Tool"=FALSE, "error in (no error)"=w1949) -> ("Analog Vars"=w1941:T2[], "error out"=w1946:errorcluster)  [unwired: 6 in, 5 out]
        n886 = Index Array(array=w1941) -> (element #1=→"PCP":T2, element #2=→"PCP Control":T2, element #3=→"PSU":T2, element #4=→"HV out":T2, element #5=→"Beagle Panel":T2, element #6=→"Tool":T2)  [unwired: 6 in]
        n887 = call "Get Digital Vars.vi"("Common alarm handling(F)"=FALSE, "Tool"=TRUE, "error in (no error)"=w1946) -> ("Values"=w1935:T108[], "Analog Vars"=w1936:T2[], "error out"=w1942:errorcluster)  [unwired: 6 in, 4 out]
        n888 = case shown="\"Stroker\", Default" w1945 {
          tunnel: w1942 -> [w2001 w2025 w2047]
          tunnel: w1936 -> [w2009 w2034 w2046]
          tunnel: w1935 -> [w2000 w2030 w2045]
          tunnel: [w1975 w2026 w2040] -> w1934
          tunnel: [w2001 w2025 w2047] -> w1930
          tunnel: w1931 -> [w1994 _ _]
          frame "Stroker", Default {
            w1995 = Status_Digitalish."True" ("y")
            n889 = Index Array(array=w2009, index #1=Variable_List_Tool_Digital."Tool node Pressure 1", index #2=Variable_List_Tool_Digital."Tool node Pressure 2", index #3=Variable_List_Tool_Digital."Tool node Solenoid", index #4=Variable_List_Tool_Digital."Upper Tension Sub", index #5=Variable_List_Tool_Digital."Tool Both Relays") -> (element #1=→"Strok Pressure 1":T2, element #2=→"Strok Pressure 2":T2, element #3=→"Strok Solenoid":T2, element #4=→"Strok Tension Sub 1":T2, element #5=w1975:T2)
            n890 = Index Array(array=w2000, index #1=Variable_List_Tool_Digital."Tool Error Pressure 1", index #2=Variable_List_Tool_Digital."Tool Error Pressure 2", index #3=Variable_List_Tool_Digital."Tool Error Solenoid", index #4=Variable_List_Tool_Digital."Tool Error Upper Tension Sub", index #5=Variable_List_Tool_Digital."Stroke Out (force)", index #6=Variable_List_Tool_Digital."Stroke In (force)") -> (element #1=→"Str Error P1":T108, element #2=→"Str Error P2":T108, element #3=→"Str Error Sol":T108, element #4=→"Str Error Tens1":T108, element #5=→"Moving right":T108, element #6=→"Moving left":T108)
            n891 = Unbundle By Name(w1994) -> ("P 4.Force det."=w1993:T66)
            n892 = Index Array(array=w2000, index #1=Variable_List_Tool_Digital."Stroke Force change not correct") -> (element #1=w1999:T108, element #2=w1998:T108, element #3=w1997:T108, element #4=w1996:T108)  [unwired: 3 in]
            n893 = Equal?(x=w1999, y=w1995) -> (x = y?=→"pressure falling":bool)
            n894 = Equal?(x=w1998, y=w1995) -> (x = y?=w1992:bool)
            n895 = Equal?(x=w1997, y=w1995) -> (x = y?=w1991:bool)
            n896 = Equal?(x=w1996, y=w1995) -> (x = y?=→"Slips total":bool)
            n897 = case shown="\"Strok out = node 1\"" w1993 {
              tunnel: w1992 -> [w2011 w2012]
              tunnel: w1991 -> [w2010 w2013]
              tunnel: [w2011 w2013] -> w1990
              tunnel: [w2010 w2012] -> w1989
              frame "Stroke in = node 1", Default {
              }
              frame "Strok out = node 1" {
              }
            }
            "Slips Venstre" <- w1990
            "Slips Høyre" <- w1989
          }
          frame "Driller" {
            n898 = Index Array(array=w2034, index #1=Variable_List_Tool_Digital."Tool node Pressure 1", index #2=Variable_List_Tool_Digital."Tool node Pressure 2", index #3=Variable_List_Tool_Digital."Tool node Solenoid", index #4=Variable_List_Tool_Digital."Mill Bit Direction", index #5=Variable_List_Tool_Digital."Oil filling mode", index #6=Variable_List_Tool_Digital."Tool Both Relays") -> (element #1=→"Dr Pressure 1":T2, element #2=→"Dr Pressure 2":T2, element #3=→"Dr Solenoid":T2, element #4=→"Drill bit direaction":T2, element #5=→"Dr Oil filling mode":T2, element #6=w2026:T2)
            n899 = Index Array(array=w2030, index #1=Variable_List_Tool_Digital."Tool Error Pressure 1", index #2=Variable_List_Tool_Digital."Tool Error Pressure 2", index #3=Variable_List_Tool_Digital."Tool Error Solenoid") -> (element #1=→"Error Dr P1":T108, element #2=→"Error Dr P2":T108, element #3=→"Error Dr Sol":T108)
          }
          frame "Tractor" {
            n900 = Index Array(array=w2046, index #1=Variable_List_Tool_Digital."Upper Tension Sub", index #2=Variable_List_Tool_Digital."Lower Tension Sub", index #3=Variable_List_Tool_Digital."Tool Both Relays") -> (element #1=→"Trac Tension Sub 1":T2, element #2=→"Trac Tension Sub 2":T2, element #3=w2040:T2)
            n901 = Index Array(array=w2045, index #1=Variable_List_Tool_Digital."Tool Error Upper Tension Sub", index #2=Variable_List_Tool_Digital."Tool Error Lower Tension Sub") -> (element #1=→"Error Tr Tension Sub 1":T108, element #2=→"Error Tr Tension Sub 2":T108)
          }
        }
        "Relay Status" <- w1934
      }
      frame "Stop" {
        # "Stop the loop. May be restarted later. Close interfaces and the like"
      }
      frame "Error Handling" {
        # "Loop automaticaly returns here after error is found. If error is cleared, \nLoop wil continue as normal(if was operative when error."
      }
      frame "End" {
        # "Only executes at application end has. Should performa any action the loop \nneeds to finnish. Executes only once."
      }
      frame "Post" {
        # "Only exists to pas true to loop conditional without extra VI. DO Not edit"
      }
    }
  }
  n902 = timed-loop "Periodicaly puts data in the application graphs" {
    shift-right: [w2140] -> _
    shift-left: _ -> [w2137]
    shift-right: [w2138] -> _
    shift-left: w2 -> [w2135]
    tunnel: [w2129] -> _
    shift-right: [w2136] -> _
    shift-left: _ -> [w2131]
    tunnel: Loop_ID."Main-Graph Upd" ("Loop ID") -> [w2132]
    timing: w12 -> [_]
    timing-out: [_] -> w11
    i -> [w2129]
    stop <- w2139 stop-if-true
    # "Update Charts"
    n903 = node-c288() -> ()  [unwired: 1 in, 1 out]
    n904 = call "emi_SMLoop Start.vi"("Loop ID"=w2132, "error in (no error)"=w2135, "Force Stop(F)"=w2131) -> ("Loop command"=w2133:T102, "error out"=w2134:errorcluster, "Loop ID out"=w2130:i32)  [unwired: 10 in]
    n905 = case shown="\"Normal Operation\"" w2133 {
      tunnel: [w2146 w2149 w2151 w2158 w2164 w2167 w2168 w2171] -> w2140
      tunnel: [_ _ _ _ _ _ _ TRUE] -> w2139
      tunnel: w2134 -> [w2147 w2148 w2150 w2159 w2165 w2166 w2169 w2172]
      tunnel: [w2147 w2148 w2150 w2152 w2165 w2166 w2169 w2172] -> w2138
      tunnel: w2137 -> [_ w2149 w2151 w2158 w2164 w2167 w2168 w2171]
      tunnel: [w2144 _ _ _ _ _ _ _] -> w2136
      tunnel: w2130 -> [_ _ _ _ _ _ _ _]
      tunnel: w2129 -> [_ _ _ _ _ _ _ _]
      frame "Init" {
        w2143 = 5  # Itt between upd
        w2144 = FALSE  # Force end
        w2145 = FALSE  # Delayed update
        # "1.7.13\n20 -> 5"
        # "First case that is executed, executes regardless of loop beeing enabled.\nOnly executes once. Init loop data and other variables."
        n906 = Bundle("Delayed update"=w2145, "Itt between upd"=w2143) -> (w2146:T110)  [unwired: 1 in]
      }
      frame "Standby", Default {
        # "Case that is executed when the loop is not enabled. Should not be edited."
      }
      frame "Start" {
        # "Start or restart the loop. Should perform any init code. \nOpen channel and so on. Will perform each time the system is restarted."
      }
      frame "Normal Operation" {
        # "Normal Throughput"
        # "All normal tasks belong here. This will be repeated, until error, disable, restart or\nforsed to restart. OBS, reduce overhead with internal loop(will execute unevenly)."
        n907 = call "Running Annotation Unmarked.vi"("error in (no error)"=w2159) -> ("Undisplayed Annotation out"=w2155:bool, "error out"=w2156:errorcluster)  [unwired: 13 in]
        n908 = call "All analog data for display.vi"("error inn"=w2156) -> ("All analog data for graph"=w2154:dbl[], "error out"=w2152:errorcluster)  [unwired: 13 in]
        n909 = case shown="True" w2155 {
          tunnel: [nan 0.0] -> w2157
          frame False {
          }
          frame True {
            n910 = call "Running Annotation Unmarked.vi"("Action(GET)"=enum16{"GET", "SET"}."SET", "Untisplayed Annotation in"=FALSE) -> ()  [unwired: 12 in, 2 out]
          }
        }
        "Annotation Chart" <- w2157
        n911 = Build Array(w2154) -> (→"Chart 1" →"Chart 2":dbl[][])
      }
      frame "Stop" {
        # "Stop the loop. May be restarted later. Close interfaces and the like"
      }
      frame "Error Handling" {
        # "Loop automaticaly returns here after error is found. If error is cleared, \nLoop wil continue as normal(if was operative when error."
      }
      frame "End" {
        # "Only executes at application end has. Should performa any action the loop \nneeds to finnish. Executes only once."
      }
      frame "Post" {
        # "Only exists to pas true to loop conditional without extra VI. DO Not edit"
      }
    }
    n912 = node-c288() -> ()  [unwired: 1 in, 1 out]
  }
  n913 = call "Graph Vindu.vi"("Loop ID Master"=Loop_ID."GUI-GrphW Mast", "Loop ID Slave"=Loop_ID."GUI-GrphW Slav", "error in (no error)"=w2) -> ()  [unwired: 13 in]
  n914 = call "Debugl Loop Dialog.vi"("Debug W1"=Loop_ID."Main-DebugW1" ("Loop ID Slave"), "Debug W2"=Loop_ID."Main-DebugW2" ("Loop ID Slave"), "error in (no error)"=w2) -> ()  [unwired: 13 in]
  n915 = call "LEIN Arbeiter.vi"("LEIN m Serial Transmitt Loop ID"=Loop_ID."LEIN-motor" ("Loop ID Slave"), "error Inn"=w2) -> ()  [unwired: 14 in]
  n916 = call "Simulator Tool Loop Dialog.vi"("Tool Sim W1"=Loop_ID."SIM-Tool W1" ("Loop ID Slave"), "Tool Sim  W2"=Loop_ID."SIM-Tool W2" ("Loop ID Slave"), "error in (no error)"=w2) -> ()  [unwired: 13 in]
  n917 = call "Alarm Loop.vi"("Loop ID"=Loop_ID."Alm-Sound", "error out"=w2) -> ()  [unwired: 14 in]
  n918 = call "File handling.vi"("Loop ID"=Loop_ID."Var Handling-File storage", "error out"=w2) -> ()  [unwired: 14 in]
  n919 = call "Tool data SIMULTERT gatheringloop.vi"("Loop ID"=Loop_ID."Var Handling-From Simulator", "error out"=w2) -> ()  [unwired: 14 in]
  n920 = call "PCP data gathering Loop.vi"("Loop ID"=Loop_ID."Var Handling-From PCP", "error in"=w2) -> ()  [unwired: 14 in]
  n921 = call "Modem Status data gathering Loop.vi"("Loop ID"=Loop_ID."Var Handling - Modem Status", "error in"=w2) -> ()  [unwired: 14 in]
  n922 = call "Puls Loop.vi"("Loop ID"=Loop_ID."Var Handling-Beat", "error out"=w2) -> ()  [unwired: 14 in]
  n923 = call "Tool measurment data collection.vi"("Quer loop"=Loop_ID."Tool data gatherer Qer" ("Loop ID"), "Stat 2 reader ID"=Loop_ID."Tool STAT2 dedicated reader" ("Loop ID"), "error out"=w2) -> ()  [unwired: 13 in]
  n924 = call "Tool detail GUI and STAT 2 collector.vi"("Detail W1"=Loop_ID."Detail View L2" ("Loop ID"), "Detail W2"=Loop_ID."Detail View L1" ("Loop ID"), "LEIN contoller STAT2 data dekoder"=Loop_ID."Tool Data LEIN STAT2 dekoder" ("Loop ID Slave"), "error in (no error)"=w2) -> ()  [unwired: 12 in]
  n925 = call "Voltage and resistance setpoint loop.vi"("Resistance setpoint Loop ID"=Loop_ID."Resistance setpoint" ("Loop ID"), "Voltage setpoint loop ID"=Loop_ID."Voltage setpoint" ("Loop ID"), "error in (no error)"=w2) -> ()  [unwired: 13 in]
  n926 = call "Nod eID handler.vi"("Loop ID"=Loop_ID."Tool ID handler", "error in (no error)"=w2) -> ()  [unwired: 14 in]
  n927 = call "SandE main loop.vi"("Loop ID"=Loop_ID."Main-SE Handler", "error in (no error)"=w2) -> ()  [unwired: 14 in]
  n928 = call "Dialog window display loop.vi"("Loop ID"=Loop_ID."Main-Dialog", "error in (no error)"=w2) -> ()  [unwired: 14 in]
  n929 = call "Stroker Wizard.vi"("Stroker Wizard L1"=Loop_ID."Stroker Wizard L1" ("Loop ID"), "Stroker Wizard L2"=Loop_ID."Stroker Wizard L2" ("Loop ID"), "error in (no error)"=w2) -> ()  [unwired: 13 in]
  n930 = call "Annotations Tip Strip.vi"("Annotations Tip Strip loop ID"=Loop_ID."Annotations Tip Strip" ("Loop ID"), "error in (no error)"=w2) -> ()  [unwired: 14 in]
  n931 = call "Magna Interface Loop.vi"("Magna IO Loop ID"=Loop_ID."Magna Interface" ("Loop ID"), "error in (no error)"=w2) -> ()  [unwired: 14 in]
  n932 = node-c288(w11) -> ()  [unwired: 1 out]
  n933 = call "Modem Status Loop.vi"("PCP IO Loop ID"=Loop_ID."Modem Status" ("Loop ID"), "error in (no error)"=w2) -> ()  [unwired: 14 in]
  n934 = call "Power Interface Detector.vi"("Power interface finder Loop ID"=Loop_ID."Power interface detector" ("Loop ID"), "error in (no error)"=w2) -> ()  [unwired: 14 in]
  n935 = while {
    tunnel: [w2178] -> _
    tunnel: w2 -> [w2176]
    tunnel: [w2174] -> _
    i -> [w2178]
    stop <- w2173 stop-if-true
    # "Moved out as test in 1.0.10. Previously in idle case"
    n936 = event shown="[20] \"HV ON\": Value Change" {
      selector: _ -> [_ _ _ _ _ _ _ _ _ _ _ _ _ _ _ _ _ _ _ _ _ _ _ _ _ _ _ _ _ _ _ _ _ _ _ _ _ _ _ _]
      dyn-events: _ -> [_ _ _ _ _ _ _ _ _ _ _ _ _ _ _ _ _ _ _ _ _ _ _ _ _ _ _ _ _ _ _ _ _ _ _ _ _ _ _ _]
      timeout: 100 -> [_ _ _ _ _ _ _ _ _ _ _ _ _ _ _ _ _ _ _ _ _ _ _ _ _ _ _ _ _ _ _ _ _ _ _ _ _ _ _ _]
      tunnel: [w2179 w2180 w2182 w2322 w2329 w2340 w2344 w2351 w2357 w2360 w2365 w2377 w2387 w2399 w2409 w2420 w2433 w2490 w2493 w2534 w2552 w2576 w2592 w2625 w2652 w2670 w2687 w2703 w2716 w2730 w2760 w2783 w2806 w2836 w2856 w2875 w2895 w2926 w2943 w2988] -> w2175
      tunnel: w2176 -> [w2179 w2180 w2183 w2323 w2330 w2337 w2345 w2352 w2358 w2361 w2366 w2378 w2388 w2400 w2410 w2421 w2428 w2489 w2491 w2538 w2547 w2577 w2591 w2624 w2654 w2669 w2686 w2702 w2715 w2729 w2759 w2782 w2805 w2837 w2857 w2876 w2896 w2927 w2944 w2989]
      event Timeout {
        n937 = event-data() -> ()  [unwired: 1 in, 2 out]
      }
      event Panel Resize {
        n938 = event-data() -> ()  [unwired: 1 in, 1 out]
      }
      event Menu Selection (User) {
        n939 = event-data() -> ("ItemTag"=w2181:string)  [unwired: 1 in]
        n940 = case shown="\"File_User\"" w2181 {
          tunnel: w2183 -> [w2184 w2186 w2191 w2196 w2203 w2206 w2210 w2214 w2218 w2222 w2229 w2235 w2238 w2247 w2265 w2286 w2299 w2309 w2312 w2315]
          tunnel: [w2184 w2188 w2190 w2201 w2204 w2207 w2211 w2215 w2219 w2221 w2228 w2236 w2239 w2251 w2270 w2289 w2298 w2310 w2313 w2316] -> w2182
          frame Default {
          }
          frame "File_User" {
            # "Memorize graph \nconfiguration for\ntool before changing \nuser"
            n941 = call "QSM enque.vi"("State"=QSM_State_List."Mem Graphs", "error in"=w2186) -> ("error out"=w2185:errorcluster)  [unwired: 13 in]
            n942 = call "QSM enque.vi"("State"=QSM_State_List."Show User Dialog", "error in"=w2185) -> ("error out"=w2188:errorcluster)  [unwired: 13 in]
          }
          frame "File_Welcome" {
            n943 = call "QSM enque.vi"("State"=QSM_State_List."Show Welcome screen", "error in"=w2191) -> ("error out"=w2190:errorcluster)  [unwired: 13 in]
          }
          frame "File_Exit" {
            w2197 = enum16{"Program Started", "Program Ended"}."Program Ended" ("App Events")
            n944 = Format Into String(error in=w2196, w2197) -> (resulting string=w2198:string, error out=w2199:errorcluster)  [unwired: 2 in]
            n945 = Concatenate Strings(w2198, " by User" ("Note(\"\")")) -> (w2195:string)
            n946 = call "Send S&E EVENT message.vi"("Event Source(user)"=S&E_Event_source."Application", "Event Description"=w2195, "error in (no error)"=w2199, "Loc Sub ID/Event ID(No ID)"=w2197) -> ("error out"=w2193:errorcluster)  [unwired: 10 in, 1 out]
            n947 = call "QSM enque.vi"("State"=QSM_State_List."End Application", "error in"=w2193) -> ("error out"=w2201:errorcluster)  [unwired: 13 in]
          }
          frame "Edit_Clear" {
            n948 = call "QSM enque.vi"("State"=QSM_State_List."Chart Clear", "error in"=w2203) -> ("error out"=w2204:errorcluster)  [unwired: 13 in]
          }
          frame "Edit_Anotate" {
            n949 = call "QSM enque.vi"("State"=QSM_State_List."Annotation, New", "error in"=w2206) -> ("error out"=w2207:errorcluster)  [unwired: 13 in]
          }
          frame "View_Upper_Graph" {
            n950 = call "QSM enque.vi"("State"=QSM_State_List."Graph Dialog Show", "Value"=0, "error in"=w2210) -> ("error out"=w2211:errorcluster)  [unwired: 12 in]
          }
          frame "View_Lower_Graph" {
            n951 = call "QSM enque.vi"("State"=QSM_State_List."Graph Dialog Show", "Value"=1, "error in"=w2214) -> ("error out"=w2215:errorcluster)  [unwired: 12 in]
          }
          frame "Detail _view" {
            n952 = call "QSM enque.vi"("State"=QSM_State_List."Show detailed view", "Value"=0, "error in"=w2218) -> ("error out"=w2219:errorcluster)  [unwired: 12 in]
          }
          frame "Sequence setup" {
            n953 = Bundle By Name(cluster=T46 {"ID"=enum."Sequence setup", "Details"=variant} ("element"), "Details"=FALSE) -> (w2224:T46)
            n954 = call "Dialog Selector SIC.vi"("error in (no error)"=w2222) -> ("Dialog Selector Q"=w2226:refnum<queue>, "error out"=w2227:errorcluster)  [unwired: 13 in]
            n955 = Enqueue Element At Opposite End(queue=w2226, element=w2224, error in (no error)=w2227) -> (error out=w2221:errorcluster)  [unwired: 1 in, 2 out]
          }
          frame "High_g_graph" {
            n956 = Bundle By Name(cluster=T46 {"ID"=enum."High G graph display", "Details"=variant} ("element"), "Details"=FALSE) -> (w2231:T46)
            n957 = call "Dialog Selector SIC.vi"("error in (no error)"=w2229) -> ("Dialog Selector Q"=w2233:refnum<queue>, "error out"=w2234:errorcluster)  [unwired: 13 in]
            n958 = Enqueue Element At Opposite End(queue=w2233, element=w2231, error in (no error)=w2234) -> (error out=w2228:errorcluster)  [unwired: 1 in, 2 out]
          }
          frame "Setup_Options" {
            n959 = call "QSM enque.vi"("State"=QSM_State_List."Show options", "error in"=w2235) -> ("error out"=w2236:errorcluster)  [unwired: 13 in]
          }
          frame "Setup_Analog" {
            n960 = call "QSM enque.vi"("State"=QSM_State_List."Dialog Tool analog", "error in"=w2238) -> ("error out"=w2239:errorcluster)  [unwired: 13 in]
          }
          frame "Tool_Stroker" {
            w2252 = User_Event_List."Stroker Activated" ("User Events")
            # "Memorize graph \nconfiguration for\ntool before changing"
            n961 = call "QSM enque.vi"("State"=QSM_State_List."Mem Graphs", "error in"=w2247) -> ("error out"=w2248:errorcluster)  [unwired: 13 in]
            n962 = call "QSM enque.vi"("State"=QSM_State_List."Change tool", "Value"=List_of_tools."Stroker" ("Tool in"), "error in"=w2248) -> ("error out"=w2243:errorcluster)  [unwired: 12 in]
            n963 = Build Array(QSM_State_List."Chart Read Settings from INI" ("State"), QSM_State_List."Chart Selection Changed" ("State"), QSM_State_List."Chart Time Changed" ("State")) -> (w2244:T30[])
            n964 = for {
              tunnel: w2244 -> [w2257] mode=indexing
              shift-right: [w2259] -> w2242
              shift-left: w2243 -> [w2258]
              n965 = call "QSM enque.vi"("State"=w2257, "error in"=w2258) -> ("error out"=w2259:errorcluster)  [unwired: 13 in]
            }
            n966 = Format Into String(error in=w2242, w2252) -> (resulting string=w2253:string, error out=w2254:errorcluster)  [unwired: 2 in]
            n967 = call "Send S&E EVENT message.vi"("Event Source(user)"=S&E_Event_source."User", "Event Description"=w2253, "error in (no error)"=w2254, "Loc Sub ID/Event ID(No ID)"=w2252) -> ("error out"=w2251:errorcluster)  [unwired: 10 in, 1 out]
          }
          frame "Tool_Driller" {
            w2271 = User_Event_List."Driller Activated" ("User Events")
            # "Memorize graph \nconfiguration for\ntool before changing"
            n968 = call "QSM enque.vi"("State"=QSM_State_List."Mem Graphs", "error in"=w2265) -> ("error out"=w2264:errorcluster)  [unwired: 13 in]
            n969 = call "QSM enque.vi"("State"=QSM_State_List."Change tool", "Value"=List_of_tools."Driller" ("Tool in"), "error in"=w2264) -> ("error out"=w2267:errorcluster)  [unwired: 12 in]
            n970 = Build Array(QSM_State_List."Chart Read Settings from INI" ("State"), QSM_State_List."Chart Selection Changed" ("State"), QSM_State_List."Chart Time Changed" ("State")) -> (w2261:T30[])
            n971 = for {
              tunnel: w2261 -> [w2276] mode=indexing
              shift-right: [w2278] -> w2269
              shift-left: w2267 -> [w2277]
              n972 = call "QSM enque.vi"("State"=w2276, "error in"=w2277) -> ("error out"=w2278:errorcluster)  [unwired: 13 in]
            }
            n973 = Format Into String(error in=w2269, w2271) -> (resulting string=w2272:string, error out=w2273:errorcluster)  [unwired: 2 in]
            n974 = call "Send S&E EVENT message.vi"("Event Source(user)"=S&E_Event_source."User", "Event Description"=w2272, "error in (no error)"=w2273, "Loc Sub ID/Event ID(No ID)"=w2271) -> ("error out"=w2270:errorcluster)  [unwired: 10 in, 1 out]
          }
          frame "Tool_Tractor" {
            w2290 = User_Event_List."Tractor Activated" ("User Events")
            # "Memorize graph \nconfiguration for\ntool before changing"
            n975 = call "QSM enque.vi"("State"=QSM_State_List."Mem Graphs", "error in"=w2286) -> ("error out"=w2285:errorcluster)  [unwired: 13 in]
            n976 = call "QSM enque.vi"("State"=QSM_State_List."Change tool", "Value"=List_of_tools."Tractor" ("Tool in"), "error in"=w2285) -> ("error out"=w2281:errorcluster)  [unwired: 12 in]
            n977 = Build Array(QSM_State_List."Chart Read Settings from INI" ("State"), QSM_State_List."Chart Selection Changed" ("State"), QSM_State_List."Chart Time Changed" ("State")) -> (w2282:T30[])
            n978 = for {
              tunnel: w2282 -> [w2295] mode=indexing
              shift-right: [w2297] -> w2280
              shift-left: w2281 -> [w2296]
              n979 = call "QSM enque.vi"("State"=w2295, "error in"=w2296) -> ("error out"=w2297:errorcluster)  [unwired: 13 in]
            }
            n980 = Format Into String(error in=w2280, w2290) -> (resulting string=w2291:string, error out=w2292:errorcluster)  [unwired: 2 in]
            n981 = call "Send S&E EVENT message.vi"("Event Source(user)"=S&E_Event_source."User", "Event Description"=w2291, "error in (no error)"=w2292, "Loc Sub ID/Event ID(No ID)"=w2290) -> ("error out"=w2289:errorcluster)  [unwired: 10 in, 1 out]
          }
          frame "Tool_STOPP" {
            w2301 = User_Event_List."Stop Tool Operation" ("User Events")
            n982 = Bundle(cluster=T54 {"PCP"=enum."HVPSU HV ON", "SP"=0.0} ("PCP beskjed"), "PCP"=PCP_High_Level_Commands."HVPSU HV OFF") -> (w2307:T54)  [unwired: 1 in]
            n983 = call "QSM enque.vi"("State"=QSM_State_List."PCP CMD", "Value"=w2307, "error in"=w2299) -> ("error out"=w2300:errorcluster)  [unwired: 12 in]
            n984 = Format Into String(error in=w2300, w2301) -> (resulting string=w2302:string, error out=w2303:errorcluster)  [unwired: 2 in]
            n985 = call "Send S&E EVENT message.vi"("Event Source(user)"=S&E_Event_source."User", "Event Description"=w2302, "error in (no error)"=w2303, "Loc Sub ID/Event ID(No ID)"=w2301) -> ("error out"=w2298:errorcluster)  [unwired: 10 in, 1 out]
          }
          frame "Tool_Analog" {
            n986 = call "QSM enque.vi"("State"=QSM_State_List."Dialog Tool analog", "error in"=w2309) -> ("error out"=w2310:errorcluster)  [unwired: 13 in]
          }
          frame "Help_About" {
            n987 = call "QSM enque.vi"("State"=QSM_State_List."Show About", "error in"=w2312) -> ("error out"=w2313:errorcluster)  [unwired: 13 in]
          }
          frame "Help_Help" {
            n988 = call "QSM enque.vi"("State"=QSM_State_List."Show Help", "error in"=w2315) -> ("error out"=w2316:errorcluster)  [unwired: 13 in]
          }
        }
      }
      event "Annotation Chart": Mouse Move {
        n989 = event-data() -> ("Coords"=w2318:T112)  [unwired: 1 in]
        n990 = Bundle By Name(cluster=T111 {"Enabled"=FALSE, "Point32"={"Horizontal"=0, "Vertical"=0}} ("Annotations Tip Strip Data in"), "Enabled"=TRUE, "Point32"=w2318) -> (w2320:T111)
        n991 = call "Annotations Tip Strip Data FGV.vi"("Action(GET)"=T29."SET", "Annotations Tip Strip Data in"=w2320, "error in (no error)"=w2323) -> ("error out"=w2322:errorcluster)  [unwired: 11 in, 1 out]
      }
      event "Annotation Chart": Mouse Leave {
        n992 = event-data() -> ()  [unwired: 1 in, 1 out]
        n993 = Bundle By Name(cluster=T111 {"Enabled"=FALSE, "Point32"={"Horizontal"=0, "Vertical"=0}} ("Annotations Tip Strip Data in"), "Enabled"=FALSE, "Point32"=T112 {"Horizontal"=0, "Vertical"=0}) -> (w2327:T111)
        n994 = call "Annotations Tip Strip Data FGV.vi"("Action(GET)"=T29."SET", "Annotations Tip Strip Data in"=w2327, "error in (no error)"=w2330) -> ("error out"=w2329:errorcluster)  [unwired: 11 in, 1 out]
      }
      event Panel Close? {
        w2335 = enum16{"Program Started", "Program Ended"}."Program Ended" ("App Events")
        # "Here, to enable logging to file befor actual closing"
        n995 = event-data() -> ()  [unwired: 1 in, 1 out]
        n996 = Format Into String(error in=w2337, w2335) -> (resulting string=w2333:string, error out=w2338:errorcluster)  [unwired: 2 in]
        n997 = Concatenate Strings(w2333, " by User" ("Note(\"\")")) -> (w2332:string)
        n998 = call "Send S&E EVENT message.vi"("Event Source(user)"=S&E_Event_source."Application", "Event Description"=w2332, "error in (no error)"=w2338, "Loc Sub ID/Event ID(No ID)"=w2335) -> ("error out"=w2336:errorcluster)  [unwired: 10 in, 1 out]
        n999 = call "QSM enque.vi"("State"=QSM_State_List."End Application", "error in"=w2336) -> ("error out"=w2340:errorcluster)  [unwired: 13 in]
        n1000 = event-data("Discard?"=TRUE) -> ()  [unwired: 1 in, 1 out]
      }
      event "About": Value Change {
        n1001 = event-data() -> ("NewVal"=w2343:bool)  [unwired: 1 in]
        n1002 = case shown="False" w2343 {
          tunnel: w2345 -> [w2348 w2349]
          tunnel: [w2347 w2349] -> w2344
          frame False {
            n1003 = call "QSM enque.vi"("State"=QSM_State_List."Show About", "error in"=w2348) -> ("error out"=w2347:errorcluster)  [unwired: 13 in]
          }
          frame True {
          }
        }
      }
      event "Options": Value Change {
        n1004 = event-data() -> ("NewVal"=w2350:bool)  [unwired: 1 in]
        n1005 = case shown="False" w2350 {
          tunnel: w2352 -> [w2355 w2356]
          tunnel: [w2354 w2356] -> w2351
          frame False {
            n1006 = call "QSM enque.vi"("State"=QSM_State_List."Show options", "error in"=w2355) -> ("error out"=w2354:errorcluster)  [unwired: 13 in]
          }
          frame True {
          }
        }
      }
      event Value Change {
        n1007 = event-data() -> ()  [unwired: 1 in, 1 out]
        n1008 = call "QSM enque.vi"("State"=QSM_State_List."Chart Selection Changed", "error in"=w2358) -> ("error out"=w2357:errorcluster)  [unwired: 13 in]
      }
      event Value Change {
        n1009 = event-data() -> ()  [unwired: 1 in, 1 out]
        n1010 = call "QSM enque.vi"("State"=QSM_State_List."Chart Time Changed", "error in"=w2361) -> ("error out"=w2360:errorcluster)  [unwired: 13 in]
      }
      event "Inspect Lower Chart", "Inspect Upper Chart": Value Change {
        n1011 = event-data() -> ("NewVal"=w2364:bool)  [unwired: 1 in]
        n1012 = case shown="True" w2364 {
          tunnel: w2366 -> [w2367 w2373]
          tunnel: [w2367 w2372] -> w2365
          tunnel: "Inspect Upper Chart" -> [_ w2371]
          frame False {
          }
          frame True {
            n1013 = Select(t=0, s=w2371, f=1) -> (s? t:f=w2368:i32)
            n1014 = call "QSM enque.vi"("State"=QSM_State_List."Graph Dialog Show", "Value"=w2368, "error in"=w2373) -> ("error out"=w2372:errorcluster)  [unwired: 12 in]
          }
        }
      }
      event "Chart 1": Mouse Down {
        n1015 = event-data() -> ("Mods"=w2376:cluster{"Double Click":bool, "Menu Key":bool})  [unwired: 1 in]
        n1016 = Unbundle By Name(w2376) -> ("Double Click"=w2375:bool)
        n1017 = case shown="True" w2375 {
          tunnel: w2378 -> [w2379 w2381]
          tunnel: [w2379 w2380] -> w2377
          frame False {
          }
          frame True {
            n1018 = disable-structure shown="Disabled" {
              disable-tunnel: w2381 -> [w2384 _]
              disable-tunnel: [w2383 _] -> w2380
              frame Disabled {
                n1019 = call "QSM enque.vi"("State"=QSM_State_List."Chart single autoscale", "Value"=0, "error in"=w2384) -> ("error out"=w2383:errorcluster)  [unwired: 12 in]
              }
              frame Enabled {
              }
            }
          }
        }
      }
      event "Chart 1": Shortcut Menu Selection (User) {
        n1020 = event-data() -> ("ItemTag"=w2386:string)  [unwired: 1 in]
        n1021 = case shown="\"Clear_Charts\"" w2386 {
          tunnel: w2388 -> [w2389 w2392 w2395]
          tunnel: [w2389 w2391 w2394] -> w2387
          frame "0", Default {
          }
          frame "Inspect" {
            n1022 = call "QSM enque.vi"("State"=QSM_State_List."Graph Dialog Show", "Value"=0, "error in"=w2392) -> ("error out"=w2391:errorcluster)  [unwired: 12 in]
          }
          frame "Clear_Charts" {
            n1023 = call "QSM enque.vi"("State"=QSM_State_List."Chart Read Settings from INI", "error in"=w2395) -> ("error out"=w2394:errorcluster)  [unwired: 13 in]
          }
        }
      }
      event "Chart 2": Mouse Down {
        n1024 = event-data() -> ("Mods"=w2398:cluster{"Double Click":bool, "Menu Key":bool})  [unwired: 1 in]
        n1025 = Unbundle By Name(w2398) -> ("Double Click"=w2397:bool)
        n1026 = case shown="True" w2397 {
          tunnel: w2400 -> [w2401 w2403]
          tunnel: [w2401 w2402] -> w2399
          frame False {
          }
          frame True {
            n1027 = disable-structure shown="Disabled" {
              disable-tunnel: w2403 -> [w2406 _]
              disable-tunnel: [w2405 _] -> w2402
              frame Disabled {
                n1028 = call "QSM enque.vi"("State"=QSM_State_List."Chart single autoscale", "Value"=1, "error in"=w2406) -> ("error out"=w2405:errorcluster)  [unwired: 12 in]
              }
              frame Enabled {
              }
            }
          }
        }
      }
      event "Chart 2": Shortcut Menu Selection (User) {
        n1029 = event-data() -> ("ItemTag"=w2408:string)  [unwired: 1 in]
        n1030 = case shown="\"Clear_Charts\"" w2408 {
          tunnel: w2410 -> [w2411 w2414 w2417]
          tunnel: [w2411 w2413 w2416] -> w2409
          frame "0", Default {
          }
          frame "Inspect" {
            n1031 = call "QSM enque.vi"("State"=QSM_State_List."Graph Dialog Show", "Value"=1, "error in"=w2414) -> ("error out"=w2413:errorcluster)  [unwired: 12 in]
          }
          frame "Clear_Charts" {
            n1032 = call "QSM enque.vi"("State"=QSM_State_List."Chart Read Settings from INI", "error in"=w2417) -> ("error out"=w2416:errorcluster)  [unwired: 13 in]
          }
        }
      }
      event "Create Anotation": Value Change {
        n1033 = event-data() -> ("NewVal"=w2419:bool)  [unwired: 1 in]
        n1034 = case shown="True" w2419 {
          tunnel: w2421 -> [w2422 w2425]
          tunnel: [w2422 w2424] -> w2420
          frame False {
          }
          frame True {
            n1035 = call "QSM enque.vi"("State"=QSM_State_List."Annotation, New", "error in"=w2425) -> ("error out"=w2424:errorcluster)  [unwired: 13 in]
          }
        }
      }
      event "Tool voltage setpoint(V)": Value Change {
        n1036 = event-data() -> ("NewVal"=w2426:dbl, "OldVal"=w2429:dbl)  [unwired: 1 in]
        n1037 = call "Get Digital Vars.vi"("Common alarm handling(F)"=FALSE, "Tool"=TRUE, "error in (no error)"=w2428) -> ("Values"=w2437:T108[], "error out"=w2435:errorcluster)  [unwired: 6 in, 5 out]
        n1038 = Index Array(array=w2437, index=Variable_List_Tool_Digital."Tool Both Relays") -> (element=w2436:T108)
        n1039 = feedback #3() -> (w2430:bool)  [unwired: 1 in]
        n1040 = case shown="\"True\"" w2436 {
          tunnel: w2426 -> [_ w2451 w2468]
          tunnel: w2435 -> [w2448 w2459 w2476]
          tunnel: [w2448 w2458 w2475] -> w2434
          tunnel: [TRUE ("T button?") w2457 w2474] -> w2432
          tunnel: [FALSE ("T button?") w2455 w2472] -> w2431
          tunnel: w2430 -> [_ w2453 w2470]
          tunnel: w2429 -> [_ w2450 w2467]
          frame "False" {
            # "Apply new settings"
            # "Tool is in motor mode. No voltage restrictions apply in this mode.\nThe warning dialog will be reset each time the software enters motor mode"
          }
          frame "True" {
            # "new value is greater than old"
            # "Tool in Passenger mode\nThe new voltage has to be confirmed is it exceeds a safe limit"
            n1041 = call "Options GFV.vi"("error in (no error)"=w2459, "Action(Get Settings)"=Action_GFV_Settings."Get Settings") -> ("Options"=w2460:T60, "error out"=w2458:errorcluster)  [unwired: 15 in, 1 out]
            n1042 = Unbundle By Name(w2460) -> ("P 3.Pass Mode Warning Voltage"=w2456:dbl)
            n1043 = Greater?(x=w2451, y=w2456) -> (0:w2454:bool)
            n1044 = Greater?(x=w2451, y=w2450) -> (0:w2449:bool)
            n1045 = Compound Arithmetic op=AND(invert w2453, w2454, w2449) -> (w2452:bool)
            n1046 = case shown="True" w2452 {
              tunnel: [TRUE ("T button?") w2464] -> w2457
              tunnel: [w2462 w2464] -> w2455
              tunnel: w2453 -> [w2462 _]
              frame False {
              }
              frame True {
                n1047 = Two Button Dialog(message="Tool is in passenger mode. Are you sure that you want to increase the voltage?") -> (T button?=w2464:bool)  [unwired: 2 in]
              }
            }
          }
          frame "NA", Default {
            # "new value is greater than old"
            # "Tool in Unknown mode\nThe new voltage has to be confirmed is it exceeds a safe limit"
            n1048 = call "Options GFV.vi"("error in (no error)"=w2476, "Action(Get Settings)"=Action_GFV_Settings."Get Settings") -> ("Options"=w2477:T60, "error out"=w2475:errorcluster)  [unwired: 15 in, 1 out]
            n1049 = Unbundle By Name(w2477) -> ("P 3.Pass Mode Warning Voltage"=w2473:dbl)
            n1050 = Greater?(x=w2468, y=w2473) -> (0:w2471:bool)
            n1051 = Greater?(x=w2468, y=w2467) -> (0:w2466:bool)
            n1052 = Compound Arithmetic op=AND(invert w2470, w2471, w2466) -> (w2469:bool)
            n1053 = case shown="True" w2469 {
              tunnel: [TRUE ("T button?") w2481] -> w2474
              tunnel: [w2479 w2481] -> w2472
              tunnel: w2470 -> [w2479 _]
              frame False {
              }
              frame True {
                n1054 = Two Button Dialog(message="Tool is in an unknown mode. Are you sure that you want to increase the voltage?") -> (T button?=w2481:bool)  [unwired: 2 in]
              }
            }
          }
        }
        n1055 = feedback-in #3(w2431) -> ()
        n1056 = case shown="False" w2432 {
          tunnel: w2426 -> [_ w2444]
          tunnel: w2434 -> [w2441 w2443]
          tunnel: [w2441 w2442] -> w2433
          tunnel: w2429 -> [w2440 _]
          frame False {
            # "discard new value"
            n1057 = local write "Tool voltage setpoint(V)"(w2440) -> ()
          }
          frame True {
            # "Apply new voltage\nlevel"
            n1058 = call "PCP Voltage Setpoint.vi"("Action(GET)"=enum16{"GET", "SET"}."SET", "PCP HV setpoint"=w2444, "error in (no error)"=w2443) -> ("error out"=w2442:errorcluster)  [unwired: 11 in, 1 out]
          }
        }
      }
      event "Tool voltage setpoint(V)": Mouse Up {
        w2485 = User_Event_List."HV SP Adjusted" ("User Events")
        # "This case is used to write to the event log that the Tool Voltage has been adjusted.\nThe value change event creates too many events when sliding so the event file would have been spammed\nIf the Tool voltage setpoint is changed in the digital display this event will not capture it."
        n1059 = event-data() -> ()  [unwired: 1 in, 1 out]
        n1060 = local read "Tool voltage setpoint(V)"() -> (w2483:dbl)
        n1061 = Format Into String(format string="%s (%#.1f)", error in=w2489, w2485, w2483) -> (resulting string=w2486:string, error out=w2487:errorcluster)  [unwired: 1 in]
        n1062 = call "Send S&E EVENT message.vi"("Event Source(user)"=S&E_Event_source."User", "Event Description"=w2486, "error in (no error)"=w2487, "Loc Sub ID/Event ID(No ID)"=w2485) -> ("error out"=w2490:errorcluster)  [unwired: 10 in, 1 out]
      }
      event "Upd Default resistance": Value Change {
        # "Updates default resistance\nby writing it to PCP or Magna"
        n1063 = event-data() -> ("NewVal"=w2492:bool)  [unwired: 1 in]
        n1064 = case shown="True" w2492 {
          tunnel: [w2494 w2500] -> w2493
          tunnel: w2491 -> [w2494 w2502]
          frame False {
          }
          frame True {
            n1065 = call "Options GFV.vi"("error in (no error)"=w2502) -> ("Options"=w2503:T60, "error out"=w2501:errorcluster)  [unwired: 16 in, 1 out]
            n1066 = Unbundle By Name(w2503) -> ("P 3.Max resistance"=w2496:dbl, "P 3.Min resistance"=w2497:dbl)
            n1067 = local read "Resistance(Ohm)"() -> (w2495:dbl)
            n1068 = In Range and Coerce(upper limit=w2496, x=w2495, lower limit=w2497) -> (coerced(x)=w2499:dbl, In Range?=w2498:bool)
            n1069 = case shown="True" w2498 {
              tunnel: w2501 -> [w2505 w2521]
              tunnel: [w2508 w2524] -> w2500
              tunnel: w2499 -> [w2507 _]
              tunnel: w2497 -> [_ w2518]
              tunnel: w2496 -> [_ w2517]
              tunnel: w2495 -> [_ w2516]
              frame True {
                w2511 = User_Event_List."Cable Resistance Updated" ("User Events")
                n1070 = property on="Resistance(Ohm)" class="DigNum (strict)"(error in=w2505, "NumText.BG Color"=u32 16777216) -> (error out=w2504:errorcluster)  [unwired: 1 in, 1 out]
                n1071 = call "PCP Resistance Setpoint.vi"("Action(GET)"=enum16{"GET", "SET"}."SET", "PCP Res setpoint"=w2507, "error in (no error)"=w2504) -> ("error out"=w2509:errorcluster)  [unwired: 11 in, 1 out]
                n1072 = Format Into String(format string="%s (%#.1f)", error in=w2509, w2511, w2507) -> (resulting string=w2512:string, error out=w2513:errorcluster)  [unwired: 1 in]
                n1073 = call "Send S&E EVENT message.vi"("Event Source(user)"=S&E_Event_source."User", "Event Description"=w2512, "error in (no error)"=w2513, "Loc Sub ID/Event ID(No ID)"=w2511) -> ("error out"=w2508:errorcluster)  [unwired: 10 in, 1 out]
              }
              frame False {
                w2526 = User_Event_List."Cable Resistance Update Failed" ("User Events")
                n1074 = Format Into String(format string="(%#.1f Ohm) is not within the allowed range (%#.1f-%#.1f Ohm)", initial string="The Cable Resistance was not updated because the setpoint ", error in=w2521, w2516, w2518, w2517) -> (resulting string=w2519:string, error out=w2520:errorcluster)
                n1075 = One Button Dialog(message=w2519) -> ()  [unwired: 1 in, 1 out]
                n1076 = Format Into String(format string="%s (%#.1f)", error in=w2520, w2526, w2516) -> (resulting string=w2527:string, error out=w2528:errorcluster)  [unwired: 1 in]
                n1077 = call "Send S&E EVENT message.vi"("Event Source(user)"=S&E_Event_source."User", "Event Description"=w2527, "error in (no error)"=w2528, "Loc Sub ID/Event ID(No ID)"=w2526) -> ("error out"=w2524:errorcluster)  [unwired: 10 in, 1 out]
              }
            }
          }
        }
      }
      event "Resistance(Ohm)": Value Change {
        n1078 = event-data() -> ()  [unwired: 1 in, 1 out]
        n1079 = call "Options GFV.vi"("error in (no error)"=w2538) -> ("Options"=w2539:T60, "error out"=w2535:errorcluster)  [unwired: 16 in, 1 out]
        n1080 = Unbundle By Name(w2539) -> ("P 3.Max resistance"=w2540:dbl, "P 3.Min resistance"=w2541:dbl)
        n1081 = In Range and Coerce(upper limit=w2540, x="Resistance(Ohm)", lower limit=w2541) -> (coerced(x)=w2537:dbl, In Range?=w2533:bool)
        n1082 = local write "Resistance(Ohm)"(w2537) -> ()
        n1083 = Select(t=u32 16776960, s=w2533, f=u32 16722474) -> (s? t:f=w2530:u32)
        n1084 = property on="Resistance(Ohm)" class="DigNum (strict)"(error in=w2535, "NumText.BG Color"=w2530) -> (error out=w2534:errorcluster)  [unwired: 1 in, 1 out]
      }
      event "HV ON": Value Change {
        n1085 = event-data() -> ("NewVal"=w2542:bool)  [unwired: 1 in]
        n1086 = call "Options GFV.vi"("error in (no error)"=w2547) -> ("Options"=w2551:T60, "error out"=w2543:errorcluster)  [unwired: 16 in, 1 out]
        n1087 = Unbundle By Name(w2551) -> ("P 3.Max resistance"=w2550:dbl, "P 3.Min resistance"=w2549:dbl)
        n1088 = local read "Resistance(Ohm)"() -> (w2548:dbl)
        n1089 = call "PCP HV on OK.vi"() -> ("PCP cHV on OKout"=w2544:bool)  [unwired: 12 in, 3 out]
        n1090 = And(x=w2544, y=w2542) -> (x .and. y?=w2545:bool)
        n1091 = In Range and Coerce(upper limit=w2550, x=w2548, lower limit=w2549) -> (coerced(x)=w2546:dbl)  [unwired: 1 out]
        n1092 = case shown="True" w2545 {
          tunnel: w2543 -> [w2554 w2556]
          tunnel: [w2554 w2563] -> w2552
          tunnel: w2546 -> [_ w2559]
          tunnel: w2542 -> [w2553 _]
          frame False {
            n1093 = case shown="True" w2553 {
              frame False {
              }
              frame True {
                n1094 = One Button Dialog(message="HV ON failed!\nMake sure that the tool voltage setpoint is set to 0 & that the HVPSU Head Voltage is below 10V!") -> ()  [unwired: 1 in, 1 out]
              }
            }
          }
          frame True {
            w2558 = T54 {"PCP"=enum."HVPSU HV ON", "SP"=0.0} ("PCP beskjed")
            w2557 = QSM_State_List."PCP CMD" ("State")
            w2565 = User_Event_List."HV ON" ("User Events")
            n1095 = local read "Tool voltage setpoint(V)"() -> (w2572:dbl)
            n1096 = Bundle(cluster=w2558, "PCP"=PCP_High_Level_Commands."Final Resistance", "SP"=w2559) -> (w2560:T54)
            n1097 = call "QSM enque.vi"("State"=w2557, "Value"=w2560, "error in"=w2556) -> ("error out"=w2561:errorcluster)  [unwired: 12 in]
            n1098 = Bundle(cluster=w2558, "PCP"=PCP_High_Level_Commands."Final Motor Voltage", "SP"=w2572) -> (w2574:T54)
            n1099 = call "QSM enque.vi"("State"=w2557, "Value"=w2574, "error in"=w2561) -> ("error out"=w2569:errorcluster)  [unwired: 12 in]
            n1100 = Bundle(cluster=w2558, "PCP"=PCP_High_Level_Commands."HVPSU HV ON") -> (w2570:T54)  [unwired: 1 in]
            n1101 = call "QSM enque.vi"("State"=w2557, "Value"=w2570, "error in"=w2569) -> ("error out"=w2564:errorcluster)  [unwired: 12 in]
            n1102 = Format Into String(error in=w2564, w2565) -> (resulting string=w2566:string, error out=w2567:errorcluster)  [unwired: 2 in]
            n1103 = call "Send S&E EVENT message.vi"("Event Source(user)"=S&E_Event_source."User", "Event Description"=w2566, "error in (no error)"=w2567, "Loc Sub ID/Event ID(No ID)"=w2565) -> ("error out"=w2563:errorcluster)  [unwired: 10 in, 1 out]
          }
        }
      }
      event "HV AV": Value Change {
        n1104 = event-data() -> ("NewVal"=w2575:bool)  [unwired: 1 in]
        n1105 = case shown="True" w2575 {
          tunnel: w2577 -> [w2578 w2589]
          tunnel: [w2578 w2579] -> w2576
          frame False {
          }
          frame True {
            w2581 = User_Event_List."HV OFF" ("User Events")
            n1106 = Bundle(cluster=T54 {"PCP"=enum."HVPSU HV ON", "SP"=0.0} ("PCP beskjed"), "PCP"=PCP_High_Level_Commands."HVPSU HV OFF") -> (w2587:T54)  [unwired: 1 in]
            n1107 = call "QSM enque.vi"("State"=QSM_State_List."PCP CMD", "Value"=w2587, "error in"=w2589) -> ("error out"=w2580:errorcluster)  [unwired: 12 in]
            n1108 = Format Into String(error in=w2580, w2581) -> (resulting string=w2582:string, error out=w2583:errorcluster)  [unwired: 2 in]
            n1109 = call "Send S&E EVENT message.vi"("Event Source(user)"=S&E_Event_source."User", "Event Description"=w2582, "error in (no error)"=w2583, "Loc Sub ID/Event ID(No ID)"=w2581) -> ("error out"=w2579:errorcluster)  [unwired: 10 in, 1 out]
          }
        }
      }
      event "Start Telemetry": Value Change {
        n1110 = event-data() -> ("NewVal"=w2593:bool, "CtlRef"=w2590:refnum<vi>)  [unwired: 1 in]
        n1111 = case shown="True" w2593 {
          tunnel: [w2600 w2612] -> w2592
          tunnel: w2591 -> [w2598 w2615]
          tunnel: w2590 -> [w2599 w2616]
          frame True {
            w2610 = User_Event_List."Start Telemetry Operation" ("User Events")
            n1112 = property class="Bool (strict)"(reference=w2599, error in=w2598, "Blinking"=TRUE) -> (error out=w2594:errorcluster)  [unwired: 1 out]
            n1113 = call "Options GFV.vi"("error in (no error)"=w2594) -> ("Options"=w2605:T60, "error out"=w2603:errorcluster)  [unwired: 16 in, 1 out]
            n1114 = Unbundle By Name(w2605) -> ("P 3.Start Telemetry Voltage"=w2601:dbl)
            n1115 = local write "Tool voltage setpoint(V)"(w2601) -> ()
            n1116 = call "PCP Voltage Setpoint.vi"("Action(GET)"=enum16{"GET", "SET"}."SET", "PCP HV setpoint"=w2601, "error in (no error)"=w2603) -> ("error out"=w2602:errorcluster)  [unwired: 11 in, 1 out]
            n1117 = Format Into String(format string="%s (%#.1f)", error in=w2602, w2610, w2601) -> (resulting string=w2607:string, error out=w2608:errorcluster)  [unwired: 1 in]
            n1118 = call "Send S&E EVENT message.vi"("Event Source(user)"=S&E_Event_source."User", "Event Description"=w2607, "error in (no error)"=w2608, "Loc Sub ID/Event ID(No ID)"=w2610) -> ("error out"=w2595:errorcluster)  [unwired: 10 in, 1 out]
            n1119 = call "QSM enque.vi"("State"=QSM_State_List."Show stroker wizard", "error in"=w2595) -> ("error out"=w2600:errorcluster)  [unwired: 13 in]
          }
          frame False {
            w2613 = 0.0 ("P 3.Start Telemetry Voltage")
            w2623 = User_Event_List."Stop Telemetry" ("User Events")
            n1120 = property class="Bool (strict)"(reference=w2616, error in=w2615, "Blinking"=FALSE) -> (error out=w2611:errorcluster)  [unwired: 1 out]
            n1121 = local write "Tool voltage setpoint(V)"(w2613) -> ()
            n1122 = call "PCP Voltage Setpoint.vi"("Action(GET)"=enum16{"GET", "SET"}."SET", "PCP HV setpoint"=w2613, "error in (no error)"=w2611) -> ("error out"=w2617:errorcluster)  [unwired: 11 in, 1 out]
            n1123 = Format Into String(format string="%s (%#.1f)", error in=w2617, w2623, w2613) -> (resulting string=w2620:string, error out=w2621:errorcluster)  [unwired: 1 in]
            n1124 = call "Send S&E EVENT message.vi"("Event Source(user)"=S&E_Event_source."User", "Event Description"=w2620, "error in (no error)"=w2621, "Loc Sub ID/Event ID(No ID)"=w2623) -> ("error out"=w2612:errorcluster)  [unwired: 10 in, 1 out]
          }
        }
      }
      event "Start Motor": Value Change {
        n1125 = event-data() -> ("NewVal"=w2626:bool)  [unwired: 1 in]
        n1126 = case shown="True" w2626 {
          tunnel: [w2631 w2643] -> w2625
          tunnel: w2624 -> [w2632 w2644]
          frame True {
            w2638 = User_Event_List."Start Motor Operation" ("User Events")
            n1127 = call "Options GFV.vi"("error in (no error)"=w2632) -> ("Options"=w2633:T60, "error out"=w2629:errorcluster)  [unwired: 16 in, 1 out]
            n1128 = Unbundle By Name(w2633) -> ("P 3.Start Motor Voltage"=w2627:dbl)
            n1129 = call "PCP Voltage Setpoint.vi"("Action(GET)"=enum16{"GET", "SET"}."SET", "PCP HV setpoint"=w2627, "error in (no error)"=w2629) -> ("error out"=w2628:errorcluster)  [unwired: 11 in, 1 out]
            n1130 = local write "Tool voltage setpoint(V)"(w2627) -> ()
            n1131 = Format Into String(format string="%s (%f)", error in=w2628, w2638, w2627) -> (resulting string=w2635:string, error out=w2636:errorcluster)  [unwired: 1 in]
            n1132 = call "Send S&E EVENT message.vi"("Event Source(user)"=S&E_Event_source."User", "Event Description"=w2635, "error in (no error)"=w2636, "Loc Sub ID/Event ID(No ID)"=w2638) -> ("error out"=w2631:errorcluster)  [unwired: 10 in, 1 out]
          }
          frame False {
            w2650 = User_Event_List."Stop Motor Operation" ("User Events")
            n1133 = call "Options GFV.vi"("error in (no error)"=w2644) -> ("Options"=w2645:T60, "error out"=w2641:errorcluster)  [unwired: 16 in, 1 out]
            n1134 = Unbundle By Name(w2645) -> ("P 3.Stop Motor Voltage"=w2639:dbl)
            n1135 = call "PCP Voltage Setpoint.vi"("Action(GET)"=enum16{"GET", "SET"}."SET", "PCP HV setpoint"=w2639, "error in (no error)"=w2641) -> ("error out"=w2640:errorcluster)  [unwired: 11 in, 1 out]
            n1136 = local write "Tool voltage setpoint(V)"(w2639) -> ()
            n1137 = Format Into String(format string="%s (%#.1f)", error in=w2640, w2650, w2639) -> (resulting string=w2647:string, error out=w2648:errorcluster)  [unwired: 1 in]
            n1138 = call "Send S&E EVENT message.vi"("Event Source(user)"=S&E_Event_source."User", "Event Description"=w2647, "error in (no error)"=w2648, "Loc Sub ID/Event ID(No ID)"=w2650) -> ("error out"=w2643:errorcluster)  [unwired: 10 in, 1 out]
          }
        }
      }
      event Key Down {
        n1139 = event-data() -> ("VKey"=w2651:T113)  [unwired: 1 in]
        n1140 = Equal?(x=eventvkey."Escape" ("VKey"), y=w2651) -> (x = y?=w2653:bool)
        n1141 = case shown="True" w2653 {
          tunnel: w2654 -> [w2656 w2659]
          tunnel: [w2656 w2657] -> w2652
          frame False {
          }
          frame True {
            w2664 = User_Event_List."ESCAPE" ("User Events")
            n1142 = Bundle(cluster=T54 {"PCP"=enum."HVPSU HV ON", "SP"=0.0} ("PCP beskjed"), "PCP"=PCP_High_Level_Commands."HVPSU HV OFF") -> (w2662:T54)  [unwired: 1 in]
            n1143 = call "QSM enque.vi"("State"=QSM_State_List."PCP CMD", "Value"=w2662, "error in"=w2659) -> ("error out"=w2658:errorcluster)  [unwired: 12 in]
            n1144 = Format Into String(error in=w2658, w2664) -> (resulting string=w2665:string, error out=w2666:errorcluster)  [unwired: 2 in]
            n1145 = call "Send S&E EVENT message.vi"("Event Source(user)"=S&E_Event_source."User", "Event Description"=w2665, "error in (no error)"=w2666, "Loc Sub ID/Event ID(No ID)"=w2664) -> ("error out"=w2657:errorcluster)  [unwired: 10 in, 1 out]
          }
        }
      }
      event "Stroker Anchor out": Value Change {
        n1146 = event-data() -> ("NewVal"=w2671:bool, "CtlRef"=w2668:refnum<vi>)  [unwired: 1 in]
        n1147 = case shown="True" w2671 {
          tunnel: [w2672 w2678] -> w2670
          tunnel: w2669 -> [w2672 w2676]
          tunnel: w2668 -> [_ w2674]
          frame False {
          }
          frame True {
            w2681 = User_Event_List."STROKER tool: Anchor Solenoid ON" ("User Events")
            n1148 = call "Set pressed button green.vi"("error in (no error)"=w2676, "Controll collection"=Controll_refrence_groups."Stroker Anchor Cmd Buttons", "Selected control"=w2674) -> ("error out"=w2675:errorcluster)  [unwired: 8 in]
            n1149 = Format Into String(error in=w2675, w2681) -> (resulting string=w2682:string, error out=w2683:errorcluster)  [unwired: 2 in]
            n1150 = call "Send S&E EVENT message.vi"("Event Source(user)"=S&E_Event_source."User", "Event Description"=w2682, "error in (no error)"=w2683, "Loc Sub ID/Event ID(No ID)"=w2681) -> ("error out"=w2677:errorcluster)  [unwired: 10 in, 1 out]
            n1151 = call "QSM enque.vi"("State"=QSM_State_List."Tool CMD", "Value"=Tool_specific_commands."Solonoid 3 (Anchor) on" ("Tool command"), "error in"=w2677) -> ("error out"=w2678:errorcluster)  [unwired: 12 in]
          }
        }
      }
      event "Stroker Anchor in": Value Change {
        n1152 = event-data() -> ("NewVal"=w2688:bool, "CtlRef"=w2685:refnum<vi>)  [unwired: 1 in]
        n1153 = case shown="True" w2688 {
          tunnel: [w2689 w2694] -> w2687
          tunnel: w2686 -> [w2689 w2693]
          tunnel: w2685 -> [_ w2692]
          frame False {
          }
          frame True {
            w2698 = User_Event_List."STROKER tool: Anchor Solenoid OFF" ("User Events")
            n1154 = call "Set pressed button green.vi"("error in (no error)"=w2693, "Controll collection"=Controll_refrence_groups."Stroker Anchor Cmd Buttons", "Selected control"=w2692) -> ("error out"=w2690:errorcluster)  [unwired: 8 in]
            n1155 = Format Into String(error in=w2690, w2698) -> (resulting string=w2699:string, error out=w2700:errorcluster)  [unwired: 2 in]
            n1156 = call "Send S&E EVENT message.vi"("Event Source(user)"=S&E_Event_source."User", "Event Description"=w2699, "error in (no error)"=w2700, "Loc Sub ID/Event ID(No ID)"=w2698) -> ("error out"=w2695:errorcluster)  [unwired: 10 in, 1 out]
            n1157 = call "QSM enque.vi"("State"=QSM_State_List."Tool CMD", "Value"=Tool_specific_commands."Solonoid 3 (Anchor) off" ("Tool command"), "error in"=w2695) -> ("error out"=w2694:errorcluster)  [unwired: 12 in]
          }
        }
      }
      event "Relays on": Value Change {
        n1158 = event-data() -> ("NewVal"=w2704:bool)  [unwired: 1 in]
        n1159 = case shown="True" w2704 {
          tunnel: [w2705 w2706] -> w2703
          tunnel: w2702 -> [w2705 w2710]
          frame False {
          }
          frame True {
            w2711 = User_Event_List."Relays set to passenger mode" ("User Events")
            n1160 = Format Into String(error in=w2710, w2711) -> (resulting string=w2712:string, error out=w2713:errorcluster)  [unwired: 2 in]
            n1161 = call "Send S&E EVENT message.vi"("Event Source(user)"=S&E_Event_source."User", "Event Description"=w2712, "error in (no error)"=w2713, "Loc Sub ID/Event ID(No ID)"=w2711) -> ("error out"=w2707:errorcluster)  [unwired: 10 in, 1 out]
            n1162 = call "QSM enque.vi"("State"=QSM_State_List."Tool CMD", "Value"=Tool_specific_commands."Controller relay 1 & 2 on" ("Tool command"), "error in"=w2707) -> ("error out"=w2706:errorcluster)  [unwired: 12 in]
          }
        }
      }
      event "Relays off": Value Change {
        n1163 = event-data() -> ("NewVal"=w2717:bool)  [unwired: 1 in]
        n1164 = case shown="True" w2717 {
          tunnel: [w2718 w2719] -> w2716
          tunnel: w2715 -> [w2718 w2723]
          frame False {
          }
          frame True {
            w2724 = User_Event_List."Relays set to motor mode" ("User Events")
            n1165 = Format Into String(error in=w2723, w2724) -> (resulting string=w2725:string, error out=w2726:errorcluster)  [unwired: 2 in]
            n1166 = call "Send S&E EVENT message.vi"("Event Source(user)"=S&E_Event_source."User", "Event Description"=w2725, "error in (no error)"=w2726, "Loc Sub ID/Event ID(No ID)"=w2724) -> ("error out"=w2720:errorcluster)  [unwired: 10 in, 1 out]
            n1167 = call "QSM enque.vi"("State"=QSM_State_List."Tool CMD", "Value"=Tool_specific_commands."Controller relay 1 & 2 off" ("Tool command"), "error in"=w2720) -> ("error out"=w2719:errorcluster)  [unwired: 12 in]
          }
        }
      }
      event "Stroker Stroke Stop": Value Change {
        n1168 = event-data() -> ("NewVal"=w2731:bool, "CtlRef"=w2728:refnum<vi>)  [unwired: 1 in]
        n1169 = case shown="True" w2731 {
          tunnel: [w2732 w2739] -> w2730
          tunnel: w2729 -> [w2732 w2738]
          tunnel: w2728 -> [_ w2737]
          frame False {
          }
          frame True {
            n1170 = call "Set pressed button green.vi"("error in (no error)"=w2738, "Controll collection"=Controll_refrence_groups."Stroker Cmd Buttons", "Selected control"=w2737) -> ("error out"=w2735:errorcluster)  [unwired: 8 in]
            n1171 = property on="Distance from target:" class="DigNum (strict)"(error in=w2735) -> (error out=w2734:errorcluster, "Visible"=w2733:bool)  [unwired: 1 in, 1 out]
            n1172 = case shown="True" w2733 {
              tunnel: [w2741 w2750] -> w2739
              tunnel: w2734 -> [w2740 w2749]
              frame True {
                w2745 = User_Event_List."STROKER tool: Stroke stop homing" ("User Events")
                # "If distance from target indicator is visible a Stop homing command is sent"
                n1173 = Format Into String(error in=w2740, w2745) -> (resulting string=w2746:string, error out=w2747:errorcluster)  [unwired: 2 in]
                n1174 = call "Send S&E EVENT message.vi"("Event Source(user)"=S&E_Event_source."User", "Event Description"=w2746, "error in (no error)"=w2747, "Loc Sub ID/Event ID(No ID)"=w2745) -> ("error out"=w2742:errorcluster)  [unwired: 10 in, 1 out]
                n1175 = call "QSM enque.vi"("State"=QSM_State_List."Tool CMD", "Value"=Tool_specific_commands."STROKER tool: Stop Homing" ("Tool command"), "error in"=w2742) -> ("error out"=w2741:errorcluster)  [unwired: 12 in]
              }
              frame False {
                w2754 = User_Event_List."Stroker Stop" ("User Events")
                n1176 = Format Into String(error in=w2749, w2754) -> (resulting string=w2755:string, error out=w2756:errorcluster)  [unwired: 2 in]
                n1177 = call "Send S&E EVENT message.vi"("Event Source(user)"=S&E_Event_source."User", "Event Description"=w2755, "error in (no error)"=w2756, "Loc Sub ID/Event ID(No ID)"=w2754) -> ("error out"=w2751:errorcluster)  [unwired: 10 in, 1 out]
                n1178 = call "QSM enque.vi"("State"=QSM_State_List."Tool CMD", "Value"=Tool_specific_commands."STROKER tool: Stroke stop" ("Tool command"), "error in"=w2751) -> ("error out"=w2750:errorcluster)  [unwired: 12 in]
              }
            }
          }
        }
      }
      event "Stroker Stroke Out": Value Change {
        n1179 = event-data() -> ("NewVal"=w2761:bool, "CtlRef"=w2758:refnum<vi>)  [unwired: 1 in]
        n1180 = case shown="True" w2761 {
          tunnel: [w2762 w2763] -> w2760
          tunnel: w2759 -> [w2762 w2776]
          tunnel: w2758 -> [_ w2775]
          frame False {
          }
          frame True {
            w2765 = User_Event_List."Stroker Extend" ("User Events")
            # "the following command\nis stop force monitoring"
            n1181 = call "Set pressed button green.vi"("error in (no error)"=w2776, "Controll collection"=Controll_refrence_groups."Stroker Cmd Buttons", "Selected control"=w2775) -> ("error out"=w2771:errorcluster)  [unwired: 8 in]
            n1182 = call "QSM enque.vi"("State"=QSM_State_List."Tool CMD", "Value"=Tool_specific_commands."STROKER tool: Stop Force Mon" ("Tool command"), "error in"=w2771) -> ("error out"=w2770:errorcluster)  [unwired: 12 in]
            n1183 = call "QSM enque.vi"("State"=QSM_State_List."Tool CMD", "Value"=Tool_specific_commands."STROKER tool: Start Force Mon dir out" ("Tool command"), "error in"=w2770) -> ("error out"=w2769:errorcluster)  [unwired: 12 in]
            n1184 = call "QSM enque.vi"("State"=QSM_State_List."Tool CMD", "Value"=Tool_specific_commands."STROKER tool: Stroke out" ("Tool command"), "error in"=w2769) -> ("error out"=w2764:errorcluster)  [unwired: 12 in]
            n1185 = Format Into String(error in=w2764, w2765) -> (resulting string=w2766:string, error out=w2767:errorcluster)  [unwired: 2 in]
            n1186 = call "Send S&E EVENT message.vi"("Event Source(user)"=S&E_Event_source."User", "Event Description"=w2766, "error in (no error)"=w2767, "Loc Sub ID/Event ID(No ID)"=w2765) -> ("error out"=w2763:errorcluster)  [unwired: 10 in, 1 out]
          }
        }
      }
      event "Stroker Stroke In": Value Change {
        n1187 = event-data() -> ("NewVal"=w2784:bool, "CtlRef"=w2781:refnum<vi>)  [unwired: 1 in]
        n1188 = case shown="True" w2784 {
          tunnel: [w2785 w2786] -> w2783
          tunnel: w2782 -> [w2785 w2795]
          tunnel: w2781 -> [_ w2794]
          frame False {
          }
          frame True {
            w2800 = User_Event_List."Stroker Retract" ("User Events")
            # "Start monitoring and run stroker in\nShould be combined into one function"
            n1189 = call "Set pressed button green.vi"("error in (no error)"=w2795, "Controll collection"=Controll_refrence_groups."Stroker Cmd Buttons", "Selected control"=w2794) -> ("error out"=w2792:errorcluster)  [unwired: 8 in]
            n1190 = call "QSM enque.vi"("State"=QSM_State_List."Tool CMD", "Value"=Tool_specific_commands."STROKER tool: Stop Force Mon" ("Tool command"), "error in"=w2792) -> ("error out"=w2791:errorcluster)  [unwired: 12 in]
            n1191 = call "QSM enque.vi"("State"=QSM_State_List."Tool CMD", "Value"=Tool_specific_commands."STROKER tool: Start Force Mon dir in" ("Tool command"), "error in"=w2791) -> ("error out"=w2788:errorcluster)  [unwired: 12 in]
            n1192 = call "QSM enque.vi"("State"=QSM_State_List."Tool CMD", "Value"=Tool_specific_commands."STROKER tool: Stroke in" ("Tool command"), "error in"=w2788) -> ("error out"=w2787:errorcluster)  [unwired: 12 in]
            n1193 = Format Into String(error in=w2787, w2800) -> (resulting string=w2801:string, error out=w2802:errorcluster)  [unwired: 2 in]
            n1194 = call "Send S&E EVENT message.vi"("Event Source(user)"=S&E_Event_source."User", "Event Description"=w2801, "error in (no error)"=w2802, "Loc Sub ID/Event ID(No ID)"=w2800) -> ("error out"=w2786:errorcluster)  [unwired: 10 in, 1 out]
          }
        }
      }
      event "Stroker Stroke Go To": Value Change {
        n1195 = event-data() -> ("NewVal"=w2807:bool, "CtlRef"=w2804:refnum<vi>)  [unwired: 1 in]
        n1196 = case shown="True" w2807 {
          tunnel: [w2808 w2817] -> w2806
          tunnel: w2805 -> [w2808 w2832]
          tunnel: w2804 -> [_ w2831]
          frame False {
          }
          frame True {
            w2809 = User_Event_List."Stroker go to Position" ("User Events")
            # "Find direction for force monitoring"
            n1197 = local read "Stroke setpoint"() -> (w2812:dbl)
            n1198 = local read "Stroker"() -> (w2829:dbl)
            n1199 = call "Set pressed button green.vi"("error in (no error)"=w2832, "Controll collection"=Controll_refrence_groups."Stroker Cmd Buttons", "Selected control"=w2831) -> ("error out"=w2821:errorcluster)  [unwired: 8 in]
            n1200 = Subtract(x=w2812, y=w2829) -> (x-y=w2828:dbl)
            n1201 = Greater Than 0?(x=w2828) -> (x > 0?=w2827:bool)
            n1202 = call "QSM enque.vi"("State"=QSM_State_List."Tool CMD", "Value"=Tool_specific_commands."STROKER tool: Stop Force Mon" ("Tool command"), "error in"=w2821) -> ("error out"=w2820:errorcluster)  [unwired: 12 in]
            n1203 = Select(t=Tool_specific_commands."STROKER tool: Start Force Mon dir out" ("Tool command"), s=w2827, f=Tool_specific_commands."STROKER tool: Start Force Mon dir in" ("Tool command")) -> (s? t:f=w2823:T55)
            n1204 = call "QSM enque.vi"("State"=QSM_State_List."Tool CMD", "Value"=w2823, "error in"=w2820) -> ("error out"=w2818:errorcluster)  [unwired: 12 in]
            n1205 = call "QSM enque.vi"("State"=QSM_State_List."Tool CMD", "Value"=Tool_specific_commands."STROKER tool: Stroke go to" ("Tool command"), "error in"=w2818) -> ("error out"=w2816:errorcluster)  [unwired: 12 in]
            n1206 = property on="Stroke setpoint" class="Slide (strict)"(error in=w2816) -> (error out=w2814:errorcluster, "Caption.Text"=w2811:string)  [unwired: 1 in, 1 out]
            n1207 = Format Into String(format string="%s (%#.1f %s)", error in=w2814, w2809, w2812, w2811) -> (resulting string=w2810:string, error out=w2813:errorcluster)  [unwired: 1 in]
            n1208 = call "Send S&E EVENT message.vi"("Event Source(user)"=S&E_Event_source."User", "Event Description"=w2810, "error in (no error)"=w2813, "Loc Sub ID/Event ID(No ID)"=w2809) -> ("error out"=w2817:errorcluster)  [unwired: 10 in, 1 out]
          }
        }
      }
      event "Force Zero": Value Change {
        n1209 = event-data() -> ("NewVal"=w2838:bool)  [unwired: 1 in]
        n1210 = case shown="True" w2838 {
          tunnel: w2837 -> [w2839 w2843]
          tunnel: [w2839 w2842] -> w2836
          frame False {
          }
          frame True {
            n1211 = Two Button Dialog(message="This action will set the measured stroke force and pressure to zero. Are you sure?") -> (T button?=w2840:bool)  [unwired: 2 in]
            n1212 = case shown="True" w2840 {
              tunnel: w2843 -> [w2844 w2848]
              tunnel: [w2844 w2851] -> w2842
              frame False {
              }
              frame True {
                w2852 = User_Event_List."Stroker - Set force and pressure to ZERO" ("User Events")
                n1213 = Build Array(Variable_List_Tool_Analog."Stroker Pressure 1" ("Variable ID"), Variable_List_Tool_Analog."Stroker Pressure 2" ("Variable ID"), Variable_List_Tool_Analog."Stroke Force" ("Variable ID")) -> (w2850:T84[])
                n1214 = call "ZERO tool variable.vi"("error in (no error)"=w2848, "Var index"=w2850) -> ("error out"=w2849:errorcluster)  [unwired: 9 in]
                n1215 = Format Into String(error in=w2849, w2852) -> (resulting string=w2853:string, error out=w2854:errorcluster)  [unwired: 2 in]
                n1216 = call "Send S&E EVENT message.vi"("Event Source(user)"=S&E_Event_source."User", "Event Description"=w2853, "error in (no error)"=w2854, "Loc Sub ID/Event ID(No ID)"=w2852) -> ("error out"=w2851:errorcluster)  [unwired: 10 in, 1 out]
              }
            }
          }
        }
      }
      event "Stroker Tension Sub Zero": Value Change {
        n1217 = event-data() -> ("NewVal"=w2858:bool)  [unwired: 1 in]
        n1218 = case shown="True" w2858 {
          tunnel: w2857 -> [w2859 w2863]
          tunnel: [w2859 w2862] -> w2856
          frame False {
          }
          frame True {
            n1219 = Two Button Dialog(message="This action will set the measured tension to zero. Are you sure?") -> (T button?=w2860:bool)  [unwired: 2 in]
            n1220 = case shown="True" w2860 {
              tunnel: w2863 -> [w2864 w2866]
              tunnel: [w2864 w2870] -> w2862
              frame False {
              }
              frame True {
                w2871 = User_Event_List."Stroker - Set tension subs to ZERO" ("User Events")
                n1221 = Build Array(Variable_List_Tool_Analog."Stroker Upper Tension Sub" ("Variable ID"), Variable_List_Tool_Analog."Stroker Lower Tension Sub" ("Variable ID")) -> (w2867:T84[])
                n1222 = call "ZERO tool variable.vi"("error in (no error)"=w2866, "Var index"=w2867) -> ("error out"=w2865:errorcluster)  [unwired: 9 in]
                n1223 = Format Into String(error in=w2865, w2871) -> (resulting string=w2872:string, error out=w2873:errorcluster)  [unwired: 2 in]
                n1224 = call "Send S&E EVENT message.vi"("Event Source(user)"=S&E_Event_source."User", "Event Description"=w2872, "error in (no error)"=w2873, "Loc Sub ID/Event ID(No ID)"=w2871) -> ("error out"=w2870:errorcluster)  [unwired: 10 in, 1 out]
              }
            }
          }
        }
      }
      event "Tractor Tension Sub Zero": Value Change {
        n1225 = event-data() -> ("NewVal"=w2877:bool)  [unwired: 1 in]
        n1226 = case shown="True" w2877 {
          tunnel: w2876 -> [w2878 w2882]
          tunnel: [w2878 w2881] -> w2875
          frame False {
          }
          frame True {
            n1227 = Two Button Dialog(message="This action will set the measured tension to zero. Are you sure?") -> (T button?=w2879:bool)  [unwired: 2 in]
            n1228 = case shown="True" w2879 {
              tunnel: w2882 -> [w2883 w2886]
              tunnel: [w2883 w2889] -> w2881
              frame False {
              }
              frame True {
                w2890 = User_Event_List."Tractor - Set Tension Subs to ZERO" ("User Events")
                n1229 = Build Array(Variable_List_Tool_Analog."Tractor Upper Tension Sub" ("Variable ID"), Variable_List_Tool_Analog."Tractor Lower Tension Sub" ("Variable ID")) -> (w2884:T84[])
                n1230 = call "ZERO tool variable.vi"("error in (no error)"=w2886, "Var index"=w2884) -> ("error out"=w2885:errorcluster)  [unwired: 9 in]
                n1231 = Format Into String(error in=w2885, w2890) -> (resulting string=w2891:string, error out=w2892:errorcluster)  [unwired: 2 in]
                n1232 = call "Send S&E EVENT message.vi"("Event Source(user)"=S&E_Event_source."User", "Event Description"=w2891, "error in (no error)"=w2892, "Loc Sub ID/Event ID(No ID)"=w2890) -> ("error out"=w2889:errorcluster)  [unwired: 10 in, 1 out]
              }
            }
          }
        }
      }
      event "Start sequence": Value Change {
        n1233 = event-data() -> ("NewVal"=w2894:bool)  [unwired: 1 in]
        n1234 = case shown="True" w2894 {
          tunnel: w2896 -> [w2897 w2909]
          tunnel: [w2897 w2910] -> w2895
          frame False {
          }
          frame True {
            n1235 = local read "Sequence to run"() -> (w2907:u16)
            n1236 = property on="Sequence to run" class="Ring (strict)"(error in=w2909) -> (error out=w2908:errorcluster, "Strings []"=w2903:string[])  [unwired: 1 in, 1 out]
            n1237 = Index Array(array=w2903) -> (element=w2902:string)  [unwired: 1 in]
            n1238 = Array Size(array=w2903) -> (size(s)=w2905:i32)
            n1239 = Index Array(array=w2903, index=w2907) -> (element=w2906:string)
            n1240 = Less Or Equal?(x=w2905, y=1) -> (x <= y?=w2899:bool)
            n1241 = Equal?(x="", y=w2902) -> (x = y?=w2900:bool)
            n1242 = And(x=w2899, y=w2900) -> (x .and. y?=w2898:bool)
            n1243 = case shown="False" w2898 {
              tunnel: [w2916 w2924] -> w2910
              tunnel: w2908 -> [w2915 w2924]
              tunnel: w2906 -> [w2912 _]
              frame False {
                w2918 = User_Event_List."Sequence start" ("User Events")
                n1244 = call-poly "emi_SMLoop Control.vi"("Loop ID in"=Loop_ID."Sequence runner" ("Loop ID"), "Enable"=TRUE, "error in (no error)"=w2915) -> ("error out"=w2917:errorcluster)  [unwired: 11 in, 1 out]
                n1245 = Format Into String(error in=w2917, w2918) -> (resulting string=w2914:string, error out=w2919:errorcluster)  [unwired: 2 in]
                n1246 = Concatenate Strings(w2914, ": " ("string"), w2912) -> (w2913:string)
                n1247 = call "Send S&E EVENT message.vi"("Event Source(user)"=S&E_Event_source."User", "Event Description"=w2913, "error in (no error)"=w2919, "Loc Sub ID/Event ID(No ID)"=w2918) -> ("error out"=w2916:errorcluster)  [unwired: 10 in, 1 out]
              }
              frame True {
                # "Intet i listen"
                n1248 = One Button Dialog(message="One or more sequences must be defined.") -> ()  [unwired: 1 in, 1 out]
              }
            }
          }
        }
      }
      event "Stopp sequence": Value Change {
        n1249 = event-data() -> ("NewVal"=w2925:bool)  [unwired: 1 in]
        n1250 = case shown="True" w2925 {
          tunnel: w2927 -> [w2928 w2936]
          tunnel: [w2928 w2929] -> w2926
          frame False {
          }
          frame True {
            w2932 = User_Event_List."Sequence stop" ("User Events")
            n1251 = call-poly "emi_SMLoop Control.vi"("Loop ID in"=Loop_ID."Sequence runner" ("Loop ID"), "Enable"=FALSE, "error in (no error)"=w2936) -> ("error out"=w2930:errorcluster)  [unwired: 11 in, 1 out]
            n1252 = Format Into String(error in=w2930, w2932) -> (resulting string=w2931:string, error out=w2933:errorcluster)  [unwired: 2 in]
            n1253 = call "Send S&E EVENT message.vi"("Event Source(user)"=S&E_Event_source."User", "Event Description"=w2931, "error in (no error)"=w2933, "Loc Sub ID/Event ID(No ID)"=w2932) -> ("error out"=w2929:errorcluster)  [unwired: 10 in, 1 out]
          }
        }
      }
      event "String Check Rec": Value Change {
        n1254 = event-data() -> ()  [unwired: 1 in, 1 out]
        n1255 = Select(t="Are you sure you want to log data during the string check?", s="String Check Rec", f="Are you sure you want to stop logging of data?") -> (s? t:f=w2939:string)
        n1256 = Two Button Dialog(message=w2939) -> (T button?=w2938:bool)  [unwired: 2 in]
        n1257 = case shown="True" w2938 {
          tunnel: w2944 -> [w2945 w2969]
          tunnel: [w2945 w2949] -> w2943
          tunnel: "String Check Rec" -> [w2947 w2960]
          frame False {
            # "Operator Cancelled dialog. Reset the Boolean Control"
            n1258 = Not(x=w2947) -> (.not. x?=w2946:bool)
            n1259 = local write "String Check Rec"(w2946) -> ()
          }
          frame True {
            w2961 = FALSE ("Run Information.Active Run")
            # "Reset Active Run cmd button"
            # "Write Project info FGV"
            n1260 = call "GFV project info.vi"("error in (no error)"=w2969) -> ("Project info out"=w2966:T96, "error out"=w2957:errorcluster)  [unwired: 13 in]
            n1261 = Get Date/Time In Seconds() -> (seconds since 1Jan1904=w2959:timestamp)
            n1262 = Unbundle By Name(w2966) -> ("Project path"=w2972:path, "Comment"=w2971:string, "data"=w2970:T97)
            n1263 = Format Into String(format string="%<%Y%m%d %H%M%S>T", error in=w2957, w2959) -> (resulting string=w2955:string, error out=w2956:errorcluster)  [unwired: 1 in]
            n1264 = Bundle By Name(cluster=w2970, "Run Information.Time of File Start"=w2955, "Run Information.String Check Rec"=w2960, "Run Information.Active Run"=w2961) -> (w2965:T97)
            n1265 = local write "Start Run"(w2961) -> ()
            n1266 = case shown="False" w2960 {
              tunnel: [w2974 w2978] -> w2962
              tunnel: [User_Event_List."String Check Recording Stopped" ("User Events") User_Event_List."String Check Recording Started" ("User Events")] -> w2948
              frame True {
                n1267 = Build Array(QSM_State_List."Stop Logging" ("State"), QSM_State_List."Start New Loggfile" ("State")) -> (w2974:T30[])
              }
              frame False {
                n1268 = Build Array(QSM_State_List."Stop Logging" ("State")) -> (w2978:T30[])
              }
            }
            n1269 = call "Create or update project ini file.vi"("Project file path"=w2972, "Comment"=w2971, "Project information"=w2965, "error in (no error)"=w2956) -> ("error out"=w2967:errorcluster)  [unwired: 11 in]
            n1270 = Bundle By Name(cluster=w2966, "data"=w2965) -> (w2964:T96)
            n1271 = call "GFV project info.vi"("Action(GET)"=enum16{"GET", "SET"}."SET", "Project info in"=w2964, "error in (no error)"=w2967) -> ("error out"=w2963:errorcluster)  [unwired: 11 in, 1 out]
            n1272 = for {
              shift-right: [w2982] -> w2950
              shift-left: w2963 -> [w2981]
              tunnel: w2962 -> [w2980] mode=indexing
              n1273 = call "QSM enque.vi"("State"=w2980, "error in"=w2981) -> ("error out"=w2982:errorcluster)  [unwired: 13 in]
            }
            n1274 = Format Into String(format string="%s", error in=w2950, w2948) -> (resulting string=w2952:string, error out=w2953:errorcluster)  [unwired: 1 in]
            n1275 = call "Send S&E EVENT message.vi"("Event Source(user)"=S&E_Event_source."User", "Event Description"=w2952, "error in (no error)"=w2953, "Loc Sub ID/Event ID(No ID)"=w2948) -> ("error out"=w2949:errorcluster)  [unwired: 10 in, 1 out]
          }
        }
      }
      event "Start Run": Value Change {
        n1276 = event-data() -> ()  [unwired: 1 in, 1 out]
        n1277 = Select(t="Are you sure you want to start a new run?", s="Start Run", f="Are you sure you want to stop the current run?") -> (s? t:f=w2985:string)
        n1278 = Two Button Dialog(message=w2985) -> (T button?=w2984:bool)  [unwired: 2 in]
        n1279 = case shown="True" w2984 {
          tunnel: w2989 -> [w2990 w3017]
          tunnel: [w2990 w2995] -> w2988
          tunnel: "Start Run" -> [w2992 w3007]
          frame False {
            n1280 = Not(x=w2992) -> (.not. x?=w2991:bool)
            n1281 = local write "Start Run"(w2991) -> ()
          }
          frame True {
            w3006 = FALSE ("Run Information.String Check Rec")
            # "Reset String check cmd button"
            # "Write Project info to file"
            # "Write Project info FGV"
            # "Read Project info FGV"
            n1282 = call "GFV project info.vi"("error in (no error)"=w3017) -> ("Project info out"=w3013:T96, "error out"=w3003:errorcluster)  [unwired: 13 in]
            n1283 = Unbundle By Name(w3013) -> ("Project path"=w3020:path, "Comment"=w3019:string, "data"=w3018:T97, "data.Run Information.Run Number"=w3015:i32)
            n1284 = Get Date/Time In Seconds() -> (seconds since 1Jan1904=w3005:timestamp)
            n1285 = Format Into String(format string="%<%Y%m%d %H%M%S>T", error in=w3003, w3005) -> (resulting string=w3001:string, error out=w3002:errorcluster)  [unwired: 1 in]
            n1286 = case shown="False" w3007 {
              tunnel: [w3022 w3026] -> w3008
              tunnel: [User_Event_List."Run Started" ("User Events") User_Event_List."Run Stopped" ("User Events")] -> w2993
              frame True {
                n1287 = Build Array(QSM_State_List."Stop Logging" ("State"), QSM_State_List."Start New Loggfile" ("State")) -> (w3022:T30[])
              }
              frame False {
                n1288 = Build Array(QSM_State_List."Stop Logging" ("State")) -> (w3026:T30[])
              }
            }
            n1289 = Increment(x=w3015) -> (x+1=w3016:i32)
            n1290 = Select(t=w3016, s=w3007, f=w3015) -> (s? t:f=w2994:i32)
            n1291 = Bundle By Name(cluster=w3018, "Run Information.Time of File Start"=w3001, "Run Information.Active Run"=w3007, "Run Information.Run Number"=w2994, "Run Information.String Check Rec"=w3006) -> (w3012:T97)
            n1292 = local write "String Check Rec"(w3006) -> ()
            n1293 = call "Create or update project ini file.vi"("Project file path"=w3020, "Comment"=w3019, "Project information"=w3012, "error in (no error)"=w3002) -> ("error out"=w3010:errorcluster)  [unwired: 11 in]
            n1294 = Bundle By Name(cluster=w3013, "data"=w3012) -> (w3011:T96)
            n1295 = call "GFV project info.vi"("Action(GET)"=enum16{"GET", "SET"}."SET", "Project info in"=w3011, "error in (no error)"=w3010) -> ("error out"=w3009:errorcluster)  [unwired: 11 in, 1 out]
            n1296 = for {
              shift-right: [w3030] -> w2996
              shift-left: w3009 -> [w3029]
              tunnel: w3008 -> [w3028] mode=indexing
              n1297 = call "QSM enque.vi"("State"=w3028, "error in"=w3029) -> ("error out"=w3030:errorcluster)  [unwired: 13 in]
            }
            n1298 = Format Into String(format string="%s (%d)", error in=w2996, w2993, w2994) -> (resulting string=w2998:string, error out=w2999:errorcluster)  [unwired: 1 in]
            n1299 = call "Send S&E EVENT message.vi"("Event Source(user)"=S&E_Event_source."User", "Event Description"=w2998, "error in (no error)"=w2999, "Loc Sub ID/Event ID(No ID)"=w2993) -> ("error out"=w2995:errorcluster)  [unwired: 10 in, 1 out]
          }
        }
      }
    }
    n1300 = call "emi_Is App Closing.vi"("error in (no error)"=w2175) -> ("error out"=w2174:errorcluster, "App Close?"=w2173:bool)  [unwired: 13 in]
  }
  n1301 = disable-structure shown="Disabled" {
    frame Disabled {
      n1302 = call "QSM enque.vi"("State"=QSM_State_List."Start New Loggfile") -> ()  [unwired: 14 in, 1 out]
    }
    frame Enabled {
    }
  }
  n1303 = while "Change Stop motor to start motor when voltage falls below Stop motor voltage" {
    stop <- FALSE stop-if-true
    # "1.18.0 #130 Set stop motor to start motor, when setpoint below"
    n1304 = call "Options GFV.vi"("Action(Get Settings)"=Action_GFV_Settings."Get Settings") -> ("Options"=w3036:T60)  [unwired: 16 in, 2 out]
    n1305 = local read "Tool voltage setpoint(V)"() -> (w3032:dbl)
    n1306 = Unbundle By Name(w3036) -> ("P 3.Stop Motor Voltage"=w3034:dbl)
    n1307 = Less?(x=w3032, y=w3034) -> (x < y?=w3033:bool)
    n1308 = case shown="True" w3033 {
      frame False {
      }
      frame True {
        n1309 = local read "Start Motor"() -> (w3039:bool)
        n1310 = case shown="True" w3039 {
          frame False {
          }
          frame True {
            n1311 = property on="Start Motor" class="Bool (strict)"("Value"=FALSE ("Start Motor")) -> ()  [unwired: 2 in, 2 out]
          }
        }
      }
    }
    n1312 = Wait Until Next ms Multiple(millisecond multiple=u32 250) -> ()  [unwired: 1 out]
  }
